vi "SetUpDigi.vi"(0 "Digitizer Settings":T31={"Digitizer delay (us) "=0.0, "rf points per line"=2048, "lines per plane"=128, "Samp Rate (Hz)"=100000000.0, "Additional dig delay (us)"=0.0, "Voltage Scale"=0.4, "Pre-Looks"=0, "Offset delay (us)"=0.0, "bits A/D"=8, "Avg Num"=1, "DigTimeOut"=5.0, "Rel Dig Delay"=0.0, "Dig Ch"=0, "LeCroyCluster"={"LeCroy Channels"=[TRUE, FALSE, FALSE, FALSE], "LC read pt offset"=0.0, "Sweep Avg"=FALSE}, "Main Digitizer"=enum."NI Digitizer", "Dig Config"=enum."Single channel", "Digitizer ID Cluster"={"Acqiris/Alazar/SP ID"=[], "NI Instr Handles"=[], "LeCroy VISA"="", "GaGe Handle"={"Handle"=0, "Sample size"=0, "Resolution"=0, "Offset"=0, "Channels"=0, "Boards"=0}, "ATS Ref"="ATS9350", "Acqiris Address"=["PCI::INSTR0"], "ADQRef"=refnum, "adq_cu_ptr"=refnum}, "Trigger Settings"={"Trig Source"=1, "Trig Coupling"=0, "Trig Slope"=0, "Level (mV)"=1500.0}, "Bulk Acq"=FALSE, "Bulk Start Indexes"=[], "Data Ref RF"=refnum, "NI ID/Channel"=[], "Total Dig CH"=1, "Xtra Ann Trig delay (us)"=10.0, "Fix Z Delay?"=FALSE, "One Way Transmission?"=FALSE, "Data Ref Log"=refnum} {"Trigger Settings"."Trig Slope" items=["Positive", "Negative"]; "Trigger Settings"."Level (mV)" format="%.2f"; "Trigger Settings"."Trig Coupling" items=["DC 1 MOhm", "AC 1 MOhm", "DC 50 Ohm", "AC 50 Ohm"]; "Trigger Settings"."Trig Source" items=["Chan 1", "External"]; "Rel Dig Delay" format="%.2f"; "DigTimeOut" format="%.2f"; "Avg Num" min=1; "Offset delay (us)" format="%.2f"; "Additional dig delay (us)" format="%.2f"; "Digitizer delay (us)" format="%.2f"}, 1 "Motion Settings In":T27={"No Motion?"=FALSE, "Motion System"=enum."NI 735x", "Motion Bd ID"=1, "Motion Profile"="SMAC1", "# Axis"=1, "Reverse Z axis?"=TRUE, "SMAC Axis"=0, "scan pair"=enum."y-(x) scan", "RT fps"=6.0, "Steps per mm"=[1000, 1000, 1000, 1000], "Motor Parameters"={"velocity ct/s"=[10000.0, 10000.0, 10000.0, 50000.0], "accel ct/s^2"=[50000.0, 50000.0, 50000.0, 200000.0]}, "One Way Scan"=FALSE, "Reverse One Way Scan"=FALSE, "Global Position (mm)"=[], "Plane"=0, "Distance between\nscan lines (um)"=0.0, "Distance between\nscan planes (um)"=0.0, "number of scan planes"=1, "Total steps in line"=0, "Xtra plane\ndistance  (um)"=100, "Xtra planes "=1, "Add Axis"=FALSE, "overshoot cts"=200, "BKPT Shift"=0, "Scan Start Time (ms)"=0, "ESP VISA"="GPIB::1::INSTR", "3rd Axis"=1, "GL Ref Out"=refnum, "Galil Address"=""} {"3rd Axis" items=["x", "y", "z", "w"]; "Xtra planes" min=1; "Xtra plane\ndistance  (um)" min=0; "Distance between\nscan planes (um)" format="%.2f"; "Distance between\nscan lines (um)" format="%.2f"; "SMAC Axis" items=["None"=0, "Axis 1"=1, "Axis 2"=2, "Axis 3"=3, "Axis 4"=4, "Axis 5"=5, "Axis 6"=6, "Axis 7"=7, "Axis 8"=8, "Vector Space 1"=17, "Vector Space 2"=18, "Vector Space 3"=19, "Vector Space 4"=20]; "Motion Bd ID" min=1 max=32 step=1}, 3 "Ann Array Params":T23={"Synth Foc?"=FALSE, "Focal Zones"=41, "Switch T/R"=0, "Trans Geometry (mm)"={"Transducer"=0, "Geo Focus"=12.0, "a (radius)"=3.0, "# of rings"=5, "kerf space "=0.1, "Center Freq"=12.0}, "Sub Ap Excite?"=FALSE, "Full Array Scan?"=FALSE, "Xmt/Rcv"={"XMIT"=[TRUE, TRUE, TRUE, TRUE, TRUE], "RCV"=[TRUE, TRUE, TRUE, TRUE, TRUE]}, "PulseSpacing (us)"=0.0, "Xmit Ring"=0, "XMIT CHS"=0, "RCV CHS"=0, "GPU?"=FALSE, "Save TIFF?"=FALSE, "downfactor"=1, "RCV 1CH"=0} {"RCV 1CH" items=["All", "1", "2", "3", "4", "5"]; "Trans Geometry (mm)"."Transducer" items=["6D 12R 40 MHz"=0, "10D 31R 20 MHz"=1, "10D 23R 20 MHz"=2, "6D 23R 40 MHz"=3, "4.5D 10.7R 40 MHz"=4, "9D 23.5R 20 MHz"=5, "9D 25.8R 20MHz"=6, "Enter"=99]; "Switch T/R" min=1 max=5 step=1}, 5 "Type of scan":T2=enum."M scan", 6 "Therapy VISA session":refnum<visa-resource-name>, 7 "Therapy (T)":bool, 8 "QAM Gate?":bool, 9 "Dual XDCR Settings":T3 {"XDCR Settings"."UT340 Controls"."Low Pass Filter (MHz)" min=-6 max=60 step=1; "XDCR Settings"."UT340 Controls"."High Pass Filter (MHz)" min=1 max=20 step=1; "XDCR Settings"."UT340 Controls"."Rep Rate (Hz)" min=20 step=1; "XDCR Settings"."UT340 Controls"."Pulse Width (ns)" min=100.0 max=250.0 step=2.0; "XDCR Settings"."UT340 Controls"."Voltage" min=100 max=250 step=2; "XDCR Settings"."UT340 Controls"."PC Gain (dB)" min=2 max=72; "XDCR Settings"."UT340 Controls"."PE Gain (dB)" min=-6 max=60 step=1; "XDCR Settings"."JSR Complete"."JSR Trigger Settings"."PRF (Hz)" items=["100 Hz"=0.1, "200 Hz"=0.2, "400 Hz"=0.4, "600 Hz"=0.6, "800 Hz"=0.8, "1000 Hz"=1.0, "1250 Hz"=1.25, "1500 Hz"=1.5, "1750 Hz"=1.75, "2000 Hz"=2.0, "2500 Hz"=2.5, "3000 Hz"=3.0, "3500 Hz"=3.5, "4000 Hz"=4.0, "4500 Hz"=4.5, "5000 Hz"=5.0]; "XDCR Settings"."JSR Complete"."JSR Trigger Settings"."Trigger Source" items=["Internal", "External"]; "XDCR Settings"."JSR Complete"."JSR Trigger Settings"."External Trigger Limit" items=["No Limit", "5 kHz"]; "XDCR Settings"."JSR Complete"."JSR Receive Settings"."Gain (dB)" min=-13 max=66 step=1; "XDCR Settings"."JSR Complete"."JSR Receive Settings"."Low Pass Filter" items=["5 MHz"=5, "10 MHz"=10, "15 MHz"=15, "22.5 MHz"=22, "35 MHz"=35, "50 MHz"=50]; "XDCR Settings"."JSR Complete"."JSR Receive Settings"."High Pass Filter" items=["DC"=0, "1 MHz"=1000, "2.5 MHz"=2500, "5 MHz"=5000, "7.5 MHz"=7500, "12.5 MHz"=12500]; "XDCR Settings"."JSR Complete"."JSR Receive Settings"."Receiver Mode" items=["Echo", "Through"]; "XDCR Settings"."JSR Complete"."JSR Pulse Settings"."Pulser Voltage (V)" items=["100"=100, "125"=125, "150"=150, "175"=175, "200"=200, "225"=225, "250"=250, "275"=275, "300"=300, "325"=325, "350"=350, "375"=375, "400"=400, "425"=425, "450"=450, "475"=475]; "XDCR Settings"."JSR Complete"."JSR Pulse Settings"."Pulser Impedance" items=["High z", "Low z"]; "XDCR Settings"."JSR Complete"."JSR Pulse Settings"."Pulse Energy Level" items=["0 (Minimum)", "1", "2", "3 (Maximum)"]; "XDCR Settings"."JSR Complete"."JSR Pulse Settings"."Damping" items=["331 Ohms"=331, "198 Ohms"=198, "142 Ohms"=142, "110 Ohms"=110, "92 Ohms"=92, "77 Ohms"=77, "67 Ohms"=67, "59 Ohms"=59, "52 Ohms"=52, "47 Ohms"=47, "43 Ohms"=43, "39 Ohms"=39, "37 Ohms"=37, "34 Ohms"=34, "32 Ohms"=32, "30 Ohms"=30]; "XDCR Settings"."Panametrics Settings"."FINE ATTENUATION" items=["00.0", "00.5", "01.0", "01.5", "02.0", "02.5", "03.0", "03.5", "04.0", "04.5", "05.0", "05.5", "06.0", "06.5", "07.0", "07.5", "08.0", "08.5", "09.0", "09.5", "10.0", "10.5", "11.0", "11.5", "12.0", "12.5", "13.0", "13.5", "14.0", "14.5", "15.0", "15.5"]; "XDCR Settings"."Panametrics Settings"."COARSE ATTENUATION" items=["00.0", "10.0", "20.0", "30.0", "40.0", "50.0"]; "XDCR Settings"."Panametrics Settings"."GAIN (db)" items=["26.0", "40.0", "54.0"]; "XDCR Settings"."Panametrics Settings"."PRF (KHz)" items=["XREMT", "EXBNC", "0.200", "0.500", "1.000", "2.000", "5.000", "10.00", "20.00"]; "XDCR Settings"."Panametrics Settings"."MODE" items=["P/ E", "THRU", "RPP", "EXT_PLSR"]; "XDCR Settings"."Panametrics Settings"."LP FILT (MHz)" items=["20", "50", "100", "200"]; "XDCR Settings"."Panametrics Settings"."HP FILT (KHz)" items=["1", "1000", "3000", "10000"]; "XDCR Settings"."Panametrics Settings"."DAMPING (Ohm)" items=["7", "10", "16", "20", "26", "30", "40", "50"]; "XDCR Settings"."Panametrics Settings"."ENERGY (uJ)" items=["1", "2", "4", "8", "16", "32"]; "XDCR Settings"."Daxsonics Settings"."Freq (MHz)" items=["4"=4, "5"=5, "6"=6, "8"=8, "10"=10, "12"=12, "14"=14, "15"=15, "16"=16, "17"=17, "18"=18, "20"=20, "25"=25, "30"=30, "35"=35, "40"=40, "45"=45, "50"=50]; "XDCR Settings"."Daxsonics Settings"."Voltage (V)" items=["0"=0, "5"=5, "10"=10, "15"=15, "20"=20, "25"=25, "30"=30, "35"=35, "40"=40, "45"=45, "50"=50, "55"=55, "60"=60, "65"=65, "70"=70, "75"=75, "80"=80, "85"=85, "90"=90, "95"=95, "100"=100, "110"=110, "120"=120, "130"=130, "140"=140, "150"=150, "160"=160, "170"=170, "180"=180, "190"=190]; "XDCR Settings"."Daxsonics Settings"."Gain (dB)" items=["22"=22, "25"=25, "28"=28, "31"=31, "34"=34, "37"=37, "40"=40, "43"=43, "46"=46, "49"=49, "52"=52, "55"=55, "58"=58, "61"=61, "64"=64, "67"=67]; "XDCR Settings"."Digitizer Settings"."Additional dig delay (ms)" format="%.2f"; "XDCR Settings"."Digitizer Settings"."Time scale per Div" items=["100 ns"=0.1, "200 ns"=0.2, "500 ns"=0.5, "1 micros"=1.0, "2 micros"=2.0, "5 micros"=5.0, "10 micros"=10.0, "20 micros"=20.0, "50 micros"=50.0, "100 micros"=100.0, "200 micros"=200.0, "500 micros"=500.0, "1 ms"=1000.0, "2 ms"=2000.0, "5 ms"=5000.0, "10 ms"=10000.0, "20 ms"=20000.0, "50 ms"=50000.0, "100 ms"=100000.0, "200 ms"=200000.0]; "XDCR Settings"."Digitizer Settings"."RF data Sampling"."rf points per line" min=1; "XDCR Settings"."Digitizer Settings"."RF data Sampling"."Ref Delay (ms)" format="%.2f"}, 18 "Equivalent RT delay\ndistance (mm)":dbl=1.5 format="%.4f") -> (11 "Dual XDCR Settings Out":T3 {"XDCR Settings"."UT340 Controls"."Low Pass Filter (MHz)" min=-6 max=60 step=1; "XDCR Settings"."UT340 Controls"."High Pass Filter (MHz)" min=1 max=20 step=1; "XDCR Settings"."UT340 Controls"."Rep Rate (Hz)" min=20 step=1; "XDCR Settings"."UT340 Controls"."Pulse Width (ns)" min=100.0 max=250.0 step=2.0; "XDCR Settings"."UT340 Controls"."Voltage" min=100 max=250 step=2; "XDCR Settings"."UT340 Controls"."PC Gain (dB)" min=2 max=72; "XDCR Settings"."UT340 Controls"."PE Gain (dB)" min=-6 max=60 step=1; "XDCR Settings"."JSR Complete"."JSR Trigger Settings"."PRF (Hz)" items=["100 Hz"=0.1, "200 Hz"=0.2, "400 Hz"=0.4, "600 Hz"=0.6, "800 Hz"=0.8, "1000 Hz"=1.0, "1250 Hz"=1.25, "1500 Hz"=1.5, "1750 Hz"=1.75, "2000 Hz"=2.0, "2500 Hz"=2.5, "3000 Hz"=3.0, "3500 Hz"=3.5, "4000 Hz"=4.0, "4500 Hz"=4.5, "5000 Hz"=5.0]; "XDCR Settings"."JSR Complete"."JSR Trigger Settings"."Trigger Source" items=["Internal", "External"]; "XDCR Settings"."JSR Complete"."JSR Trigger Settings"."External Trigger Limit" items=["No Limit", "5 kHz"]; "XDCR Settings"."JSR Complete"."JSR Receive Settings"."Gain (dB)" min=-13 max=66 step=1; "XDCR Settings"."JSR Complete"."JSR Receive Settings"."Low Pass Filter" items=["5 MHz"=5, "10 MHz"=10, "15 MHz"=15, "22.5 MHz"=22, "35 MHz"=35, "50 MHz"=50]; "XDCR Settings"."JSR Complete"."JSR Receive Settings"."High Pass Filter" items=["DC"=0, "1 MHz"=1000, "2.5 MHz"=2500, "5 MHz"=5000, "7.5 MHz"=7500, "12.5 MHz"=12500]; "XDCR Settings"."JSR Complete"."JSR Receive Settings"."Receiver Mode" items=["Echo", "Through"]; "XDCR Settings"."JSR Complete"."JSR Pulse Settings"."Pulser Voltage (V)" items=["100"=100, "125"=125, "150"=150, "175"=175, "200"=200, "225"=225, "250"=250, "275"=275, "300"=300, "325"=325, "350"=350, "375"=375, "400"=400, "425"=425, "450"=450, "475"=475]; "XDCR Settings"."JSR Complete"."JSR Pulse Settings"."Pulser Impedance" items=["High z", "Low z"]; "XDCR Settings"."JSR Complete"."JSR Pulse Settings"."Pulse Energy Level" items=["0 (Minimum)", "1", "2", "3 (Maximum)"]; "XDCR Settings"."JSR Complete"."JSR Pulse Settings"."Damping" items=["331 Ohms"=331, "198 Ohms"=198, "142 Ohms"=142, "110 Ohms"=110, "92 Ohms"=92, "77 Ohms"=77, "67 Ohms"=67, "59 Ohms"=59, "52 Ohms"=52, "47 Ohms"=47, "43 Ohms"=43, "39 Ohms"=39, "37 Ohms"=37, "34 Ohms"=34, "32 Ohms"=32, "30 Ohms"=30]; "XDCR Settings"."Panametrics Settings"."FINE ATTENUATION" items=["00.0", "00.5", "01.0", "01.5", "02.0", "02.5", "03.0", "03.5", "04.0", "04.5", "05.0", "05.5", "06.0", "06.5", "07.0", "07.5", "08.0", "08.5", "09.0", "09.5", "10.0", "10.5", "11.0", "11.5", "12.0", "12.5", "13.0", "13.5", "14.0", "14.5", "15.0", "15.5"]; "XDCR Settings"."Panametrics Settings"."COARSE ATTENUATION" items=["00.0", "10.0", "20.0", "30.0", "40.0", "50.0"]; "XDCR Settings"."Panametrics Settings"."GAIN (db)" items=["26.0", "40.0", "54.0"]; "XDCR Settings"."Panametrics Settings"."PRF (KHz)" items=["XREMT", "EXBNC", "0.200", "0.500", "1.000", "2.000", "5.000", "10.00", "20.00"]; "XDCR Settings"."Panametrics Settings"."MODE" items=["P/ E", "THRU", "RPP", "EXT_PLSR"]; "XDCR Settings"."Panametrics Settings"."LP FILT (MHz)" items=["20", "50", "100", "200"]; "XDCR Settings"."Panametrics Settings"."HP FILT (KHz)" items=["1", "1000", "3000", "10000"]; "XDCR Settings"."Panametrics Settings"."DAMPING (Ohm)" items=["7", "10", "16", "20", "26", "30", "40", "50"]; "XDCR Settings"."Panametrics Settings"."ENERGY (uJ)" items=["1", "2", "4", "8", "16", "32"]; "XDCR Settings"."Daxsonics Settings"."Freq (MHz)" items=["4"=4, "5"=5, "6"=6, "8"=8, "10"=10, "12"=12, "14"=14, "15"=15, "16"=16, "17"=17, "18"=18, "20"=20, "25"=25, "30"=30, "35"=35, "40"=40, "45"=45, "50"=50]; "XDCR Settings"."Daxsonics Settings"."Voltage (V)" items=["0"=0, "5"=5, "10"=10, "15"=15, "20"=20, "25"=25, "30"=30, "35"=35, "40"=40, "45"=45, "50"=50, "55"=55, "60"=60, "65"=65, "70"=70, "75"=75, "80"=80, "85"=85, "90"=90, "95"=95, "100"=100, "110"=110, "120"=120, "130"=130, "140"=140, "150"=150, "160"=160, "170"=170, "180"=180, "190"=190]; "XDCR Settings"."Daxsonics Settings"."Gain (dB)" items=["22"=22, "25"=25, "28"=28, "31"=31, "34"=34, "37"=37, "40"=40, "43"=43, "46"=46, "49"=49, "52"=52, "55"=55, "58"=58, "61"=61, "64"=64, "67"=67]; "XDCR Settings"."Digitizer Settings"."Additional dig delay (ms)" format="%.2f"; "XDCR Settings"."Digitizer Settings"."Time scale per Div" items=["100 ns"=0.1, "200 ns"=0.2, "500 ns"=0.5, "1 micros"=1.0, "2 micros"=2.0, "5 micros"=5.0, "10 micros"=10.0, "20 micros"=20.0, "50 micros"=50.0, "100 micros"=100.0, "200 micros"=200.0, "500 micros"=500.0, "1 ms"=1000.0, "2 ms"=2000.0, "5 ms"=5000.0, "10 ms"=10000.0, "20 ms"=20000.0, "50 ms"=50000.0, "100 ms"=100000.0, "200 ms"=200000.0]; "XDCR Settings"."Digitizer Settings"."RF data Sampling"."rf points per line" min=1; "XDCR Settings"."Digitizer Settings"."RF data Sampling"."Ref Delay (ms)" format="%.2f"}, 12 "Digitizer Settings Out":T31={"Digitizer delay (us) "=0.0, "rf points per line"=2048, "lines per plane"=128, "Samp Rate (Hz)"=100000000.0, "Additional dig delay (us)"=0.0, "Voltage Scale"=0.4, "Pre-Looks"=0, "Offset delay (us)"=0.0, "bits A/D"=8, "Avg Num"=1, "DigTimeOut"=5.0, "Rel Dig Delay"=0.0, "Dig Ch"=0, "LeCroyCluster"={"LeCroy Channels"=[TRUE, FALSE, FALSE, FALSE], "LC read pt offset"=0.0, "Sweep Avg"=FALSE}, "Main Digitizer"=enum."NI Digitizer", "Dig Config"=enum."Single channel", "Digitizer ID Cluster"={"Acqiris/Alazar/SP ID"=[], "NI Instr Handles"=[], "LeCroy VISA"="", "GaGe Handle"={"Handle"=0, "Sample size"=0, "Resolution"=0, "Offset"=0, "Channels"=0, "Boards"=0}, "ATS Ref"="ATS9350", "Acqiris Address"=["PCI::INSTR0"], "ADQRef"=refnum, "adq_cu_ptr"=refnum}, "Trigger Settings"={"Trig Source"=1, "Trig Coupling"=0, "Trig Slope"=0, "Level (mV)"=1500.0}, "Bulk Acq"=FALSE, "Bulk Start Indexes"=[], "Data Ref RF"=refnum, "NI ID/Channel"=[], "Total Dig CH"=1, "Xtra Ann Trig delay (us)"=10.0, "Fix Z Delay?"=FALSE, "One Way Transmission?"=FALSE, "Data Ref Log"=refnum} {"Trigger Settings"."Trig Slope" items=["Positive", "Negative"]; "Trigger Settings"."Level (mV)" format="%.2f"; "Trigger Settings"."Trig Coupling" items=["DC 1 MOhm", "AC 1 MOhm", "DC 50 Ohm", "AC 50 Ohm"]; "Trigger Settings"."Trig Source" items=["Chan 1", "External"]; "Rel Dig Delay" format="%.2f"; "DigTimeOut" format="%.2f"; "Avg Num" min=1; "Offset delay (us)" format="%.2f"; "Additional dig delay (us)" format="%.2f"; "Digitizer delay (us)" format="%.2f"}, 13 "Motion Settings Out":T27={"No Motion?"=FALSE, "Motion System"=enum."NI 735x", "Motion Bd ID"=1, "Motion Profile"="SMAC1", "# Axis"=1, "Reverse Z axis?"=TRUE, "SMAC Axis"=0, "scan pair"=enum."y-(x) scan", "RT fps"=6.0, "Steps per mm"=[1000, 1000, 1000, 1000], "Motor Parameters"={"velocity ct/s"=[10000.0, 10000.0, 10000.0, 50000.0], "accel ct/s^2"=[50000.0, 50000.0, 50000.0, 200000.0]}, "One Way Scan"=FALSE, "Reverse One Way Scan"=FALSE, "Global Position (mm)"=[], "Plane"=0, "Distance between\nscan lines (um)"=0.0, "Distance between\nscan planes (um)"=0.0, "number of scan planes"=1, "Total steps in line"=0, "Xtra plane\ndistance  (um)"=100, "Xtra planes "=1, "Add Axis"=FALSE, "overshoot cts"=200, "BKPT Shift"=0, "Scan Start Time (ms)"=0, "ESP VISA"="GPIB::1::INSTR", "3rd Axis"=1, "GL Ref Out"=refnum, "Galil Address"=""} {"3rd Axis" items=["x", "y", "z", "w"]; "Xtra planes" min=1; "Xtra plane\ndistance  (um)" min=0; "Distance between\nscan planes (um)" format="%.2f"; "Distance between\nscan lines (um)" format="%.2f"; "SMAC Axis" items=["None"=0, "Axis 1"=1, "Axis 2"=2, "Axis 3"=3, "Axis 4"=4, "Axis 5"=5, "Axis 6"=6, "Axis 7"=7, "Axis 8"=8, "Vector Space 1"=17, "Vector Space 2"=18, "Vector Space 3"=19, "Vector Space 4"=20]; "Motion Bd ID" min=1 max=32 step=1}, 14 "Vert Settings":cluster{dbl, dbl, "Coupling":u16}, 15 "RF data Sampling Out":T36={"Sampling Rate"=6.0, "Ref Delay (ms)"=0.0, "rf points per line"=2048} {"rf points per line" min=1; "Ref Delay (ms)" format="%.2f"; "Sampling Rate" items=["10 MS/s"=10.0, "20 MS/s"=20.0, "25 MS/s"=25.0, "50 MS/s"=50.0, "100 MS/s"=100.0, "200 MS/s"=200.0, "250 MS/s"=250.0, "500 MS/s"=500.0, "1 GS/s"=1000.0]}, 17 "Waveform Graph":cluster{i32, dbl, "Array":dbl[]}(graph), 19 "Ann Array Params out":T23={"Synth Foc?"=FALSE, "Focal Zones"=41, "Switch T/R"=0, "Trans Geometry (mm)"={"Transducer"=0, "Geo Focus"=12.0, "a (radius)"=3.0, "# of rings"=5, "kerf space "=0.1, "Center Freq"=12.0}, "Sub Ap Excite?"=FALSE, "Full Array Scan?"=FALSE, "Xmt/Rcv"={"XMIT"=[TRUE, TRUE, TRUE, TRUE, TRUE], "RCV"=[TRUE, TRUE, TRUE, TRUE, TRUE]}, "PulseSpacing (us)"=0.0, "Xmit Ring"=0, "XMIT CHS"=0, "RCV CHS"=0, "GPU?"=FALSE, "Save TIFF?"=FALSE, "downfactor"=1, "RCV 1CH"=0} {"RCV 1CH" items=["All", "1", "2", "3", "4", "5"]; "Trans Geometry (mm)"."Transducer" items=["6D 12R 40 MHz"=0, "10D 31R 20 MHz"=1, "10D 23R 20 MHz"=2, "6D 23R 40 MHz"=3, "4.5D 10.7R 40 MHz"=4, "9D 23.5R 20 MHz"=5, "9D 25.8R 20MHz"=6, "Enter"=99]; "Switch T/R" min=1 max=5 step=1})   [LabVIEW 2022 SP3]
uses:
  -DigitizerRoutines/DigitizerSettings.ctl
  -DigitizerRoutines/Digitizer.ctl
  -DigitizerRoutines/DigConfig.ctl
  -DigitizerRoutines/DigitizerID.ctl
  C:/Windows/System32/ADQAPI_dotNet_helper.dll
  Windows/System32/ADQAPI_dotNet_helper.dll
  Motion Controllers/NI_controller/-NI_MotionRoutines/MotionParameters.ctl
  Motion Controllers/NI_controller/-NI_MotionRoutines/MotionSys.ctl
  Motion Controllers/-MotionRoutines/ScanAxis.ctl
  Motion Controllers/-MotionRoutines/3rdAxis.ctl
  Annular Array/-AnnularRoutines/AnnularArray.ctl
  Annular Array/-AnnularRoutines/TransGeometry.ctl
  Annular Array/-AnnularRoutines/ArrayGeometry.ctl
  Pulsers/pulser.ctl
  DualXDCR/Dual XDCR Complete Settings.ctl
  DualXDCR/XDCRSettings.ctl
  Pulsers/Daxsonics/-DaxSubroutines/Dax_Control_Cluster.ctl
  Pulsers/Panametrics/Pana5900.ctl
  Pulsers/JSR/Controls/JSR Complete.ctl
  Pulsers/JSR/Controls/JSR Pulse.ctl
  Pulsers/JSR/Controls/Damping.ctl
  Pulsers/JSR/Controls/Energy.ctl
  Pulsers/JSR/Controls/Z.ctl
  Pulsers/JSR/Controls/Volt.ctl
  Pulsers/JSR/Controls/JSR Recieve.ctl
  Pulsers/JSR/Controls/Mode.ctl
  Pulsers/JSR/Controls/HPF.ctl
  Pulsers/JSR/Controls/LPF.ctl
  Pulsers/JSR/Controls/Gain.ctl
  Pulsers/JSR/Controls/JSR Trigger.ctl
  Pulsers/JSR/Controls/Trig Limit.ctl
  Pulsers/JSR/Controls/Trig Source.ctl
  Pulsers/JSR/Controls/PRF.ctl
  Pulsers/UTEX/Controls/UTEX Controls.ctl
  -ScanSystem/Controls/ScanType2.ctl
  Motion Controllers/Galil/Command Menu.ctl
  -ScanSystem/Controls/location.ctl
  <vilib>/DAQmx/write.llb/DAQmx Write (Digital Bool 1Line 1Point).vi
  <vilib>/Analysis/2dsp.llb/Decimate (single shot, DBL).vi
  <vilib>/Analysis/baseanly.llb/Mean (DBL).vi
  Motion Controllers/-MotionRoutines/MotionGlobals.vi
  Pulsers/PulserGlobals.vi
  Switch Modules/SwitchGlobals.vi
  <vilib>/DAQmx/miscellaneous.llb/DAQmx Fill In Error Info.vi
  <vilib>/DAQmx/create/channels.llb/DAQmx Create Channel (CO-Pulse Generation-Frequency).vi
  <vilib>/DAQmx/configure/timing.llb/DAQmx Timing (Implicit).vi
  <vilib>/DAQmx/create/channels.llb/DAQmx Create Channel (CO-Pulse Generation-Time).vi
  <vilib>/DAQmx/configure/trigger.llb/DAQmx Start Trigger (Digital Edge).vi
  <instrlib>/niScope/Acquire/Fetch/niScope Fetch.vi
  <vilib>/Utility/file.llb/Write Delimited Spreadsheet (DBL).vi
  -DigitizerRoutines/DigitizerGlobals.vi
  <resource>/objmgr/daqmx.rc
  <instrlib>/Newport ESP301/Newport ESP301.lvlib
  <instrlib>/Acqiris Dx/Acqiris Dx.lvlib
  <instrlib>/Acqiris Bx/Acqiris Bx.lvlib
  <vilib>/Analysis/NI_AALBase.lvlib
  <vilib>/Analysis/NI_AALPro.lvlib
  <instrlib>/niSwitch/niSwitch.llb/niSwitch Connect Channels (Single).vi
  <vilib>/Motion/FlexMotion/FunctionsVIs/StartStopMotion.llb/Start Motion (8 axes).flx
  <vilib>/Motion/FlexMotion/FunctionsVIs/StartStopMotion.llb/Stop Motion (8 axes).flx
panel:
  out "Samp rate":dbl
  out "AlazarCluster":T1
  in  "Norm Spect?":bool
  in  "Filter":bool
  in  "Filter Prameters":T26={"low cutoff"=5, "order"=81, "high cutoff"=65}
  in  "Inc. Step Size (mm)":dbl=0.5
  in  "Settings Changes":bool
  in  "Crate Spectra":bool
  out "Crate Waveforms":cluster{i32, "Clock (s)":dbl, dbl[][]}(graph)
  in  "Display Channel":i32(slide) min=0 max=5 step=1 scale=0.0..5.0
  in  "Position (mm) (Abs)":dbl format="%.3f"
  in  "Stop Motor":bool
  in  "Axis Tune":enum32{"Axis 1", "Axis 2", "Axis 3", "Axis 4"}(radio)
  in  "Tab Control":T35(tab)
  in  "RF data Sampling":T36={"Sampling Rate"=100.0, "Ref Delay (ms)"=0.0, "rf points per line"=2048} {"rf points per line" min=1; "Ref Delay (ms)" format="%.2f"}
  in  "Trigger Settings":T37={"Trig Source"=1, "Trig Coupling"=0, "Trig Slope"=0, "Level (mV)"=1500.0} {"Trig Slope" items=["Positive", "Negative"]; "Level (mV)" format="%.2f"; "Trig Coupling" items=["DC 1 MOhm", "AC 1 MOhm", "DC 50 Ohm", "AC 50 Ohm"]; "Trig Source" items=["Chan 1", "External"]}
  out "Error Message":string
  in  "Time scale per Div":dbl(ring)=5.0 items=["200 ns"=0.2, "400 ns"=0.4, "1 micros"=1.0, "2 micros"=2.0, "5 micros"=5.0, "10 micros"=10.0, "20 micros"=20.0, "50 micros"=50.0, "100 micros"=100.0]
  out "Total Delay (ms)":dbl=1.5 format="%.3f"
  in  "Channel tab":enum32{"C1", "C2", "C3", "C4"}(tab)
  in  "Volt Scale 1":dbl(ring)=2.0 items=["8 V"=8.0, "4 V"=4.0, "2 V"=2.0, "800 mV"=0.8, "400 mV"=0.4, "200 mV"=0.2, "80 mV"=0.08]
  in  "Coupling C1":u16(ring)=2 items=["DC 1 MOhm", "AC 1 MOhm", "DC 50 Ohm", "AC 50 OHM"]
  in  "Volt Scale 2":dbl(ring)=0.4 items=["8 V"=8.0, "4 V"=4.0, "2 V"=2.0, "800 mV"=0.8, "400 mV"=0.4, "200 mV"=0.2, "80 mV"=0.08]
  in  "Coupling C2":u16(ring)=2 items=["DC 1 MOhm", "AC 1 MOhm", "DC 50 Ohm", "AC 50 OHM"]
  in  "Volt Scale 3":dbl(ring)=0.4 items=["8 V"=8.0, "4 V"=4.0, "2 V"=2.0, "800 mV"=0.8, "400 mV"=0.4, "200 mV"=0.2, "80 mV"=0.08]
  in  "Coupling C3":u16(ring)=2 items=["DC 1 MOhm", "AC 1 MOhm", "DC 50 Ohm", "AC 50 OHM"]
  in  "Volt Scale 4":dbl(ring)=0.4 items=["8 V"=8.0, "4 V"=4.0, "2 V"=2.0, "800 mV"=0.8, "400 mV"=0.4, "200 mV"=0.2, "80 mV"=0.08]
  in  "Coupling C4":u16(ring)=2 items=["DC 1 MOhm", "AC 1 MOhm", "DC 50 Ohm", "AC 50 OHM"]
  in  "Therapy Burst Set Up":T38={"Therapy Set Up"={"Cycles"=1.0, "Frequency (MHz)"=40.0, "Amplitude (mV)"=200.0}, "Divide prf by"=1, "Therapy Delay (ms) "=10.0, "Counter On (T)"=TRUE} {"Therapy Delay (ms)" min=0.025 format="%.3f"; "Therapy Set Up"."Amplitude (mV)" min=50.0 max=1000.0 format="%.2f"; "Therapy Set Up"."Frequency (MHz)" min=0.01 max=200.0 format="%.4f"; "Therapy Set Up"."Cycles" min=1 max=50000 step=1 format="%.3f"}
  out "Lines in burst":i32=1 min=1 max=50000 step=1
  in  "Gate duration (mics)":dbl=12.0 min=0.025
  in  "cycles (f), time(t)":bool=TRUE
  in  "Func Gen":u16(ring)=1 items=["Agilent", "Tabor"]
  in  "Config Breath":bool
  in  "Set Spectrometer":bool
  in  "Delay Corr?":bool=TRUE
  in  "Offset (mV)":dbl
  in  "Custom Waveform":bool
  in  "Pulser":T39
  in  "Offset delay (us)":dbl
  in  "One Way Transmission?":bool
  in  "Attenuation":u8(slide) scale=0.0..63.0
  out "Gage Delay Pts":dbl
  out "CTR Tasks":refnum<k21>[](array[refnum])
  in  "Slave Voltage Scales":bool=TRUE
  out "Nominal Samples":i32
  out "t per div":dbl
  in  "Crate Voltage Scales":dbl[](array[ring])=[2.0, 2.0, 2.0, 2.0] items=["8 V"=8.0, "4 V"=4.0, "2 V"=2.0, "800 mV"=0.8, "400 mV"=0.4, "200 mV"=0.2, "80 mV"=0.08]
  in  "Crate Delay":dbl
  in  "Display Crate?":bool
  in  "Man Cont":bool
  in  "T/R Channel":u32(slide)=1 min=1 max=8 step=1 scale=1.0..5.0
  in  "Save trace?":bool
  in  "Set Pulser":bool
  in  "go to scan type":bool
  in  "ExitSendCmd":bool
  in  "Crate Coupling":u16(ring)=2 items=["DC 1 MOhm", "AC 1 MOhm", "DC 50 Ohm", "AC 50 OHM"]
  out "dup id":i32
  # "Key Board Short Cuts\nX: \t      Autoscale in X\nY: \t      Autoscale in Y\nSpace Bar:           Exit\n\nShift:           Step * 0.1\nCtrl:          Step * 0.01"
  # "Z: \t\t             +W\nC: \t\t              -W\nPageUp:      \t+Z\nPageDown:\t   -Z\nUp Arrow:\t    +Y\nDown Arrow: \t-Y\nLeft Arrow: \t  +X\nRight Arrow:  -X"
  # "© 2000-2022 Weill Cornel"
  # "Array Mode Settings and Display"
  # "Position Adjustment"
  # "Yellow curser used for additional delay. RF data is captured between yellow and red lines."
  # "All"
  # "1-D and 2-D B scan settings"
  # "1-D and 2-D B scan settings"
  # "Scale Settings"
  # "Controls only visible\nwhen needed.."
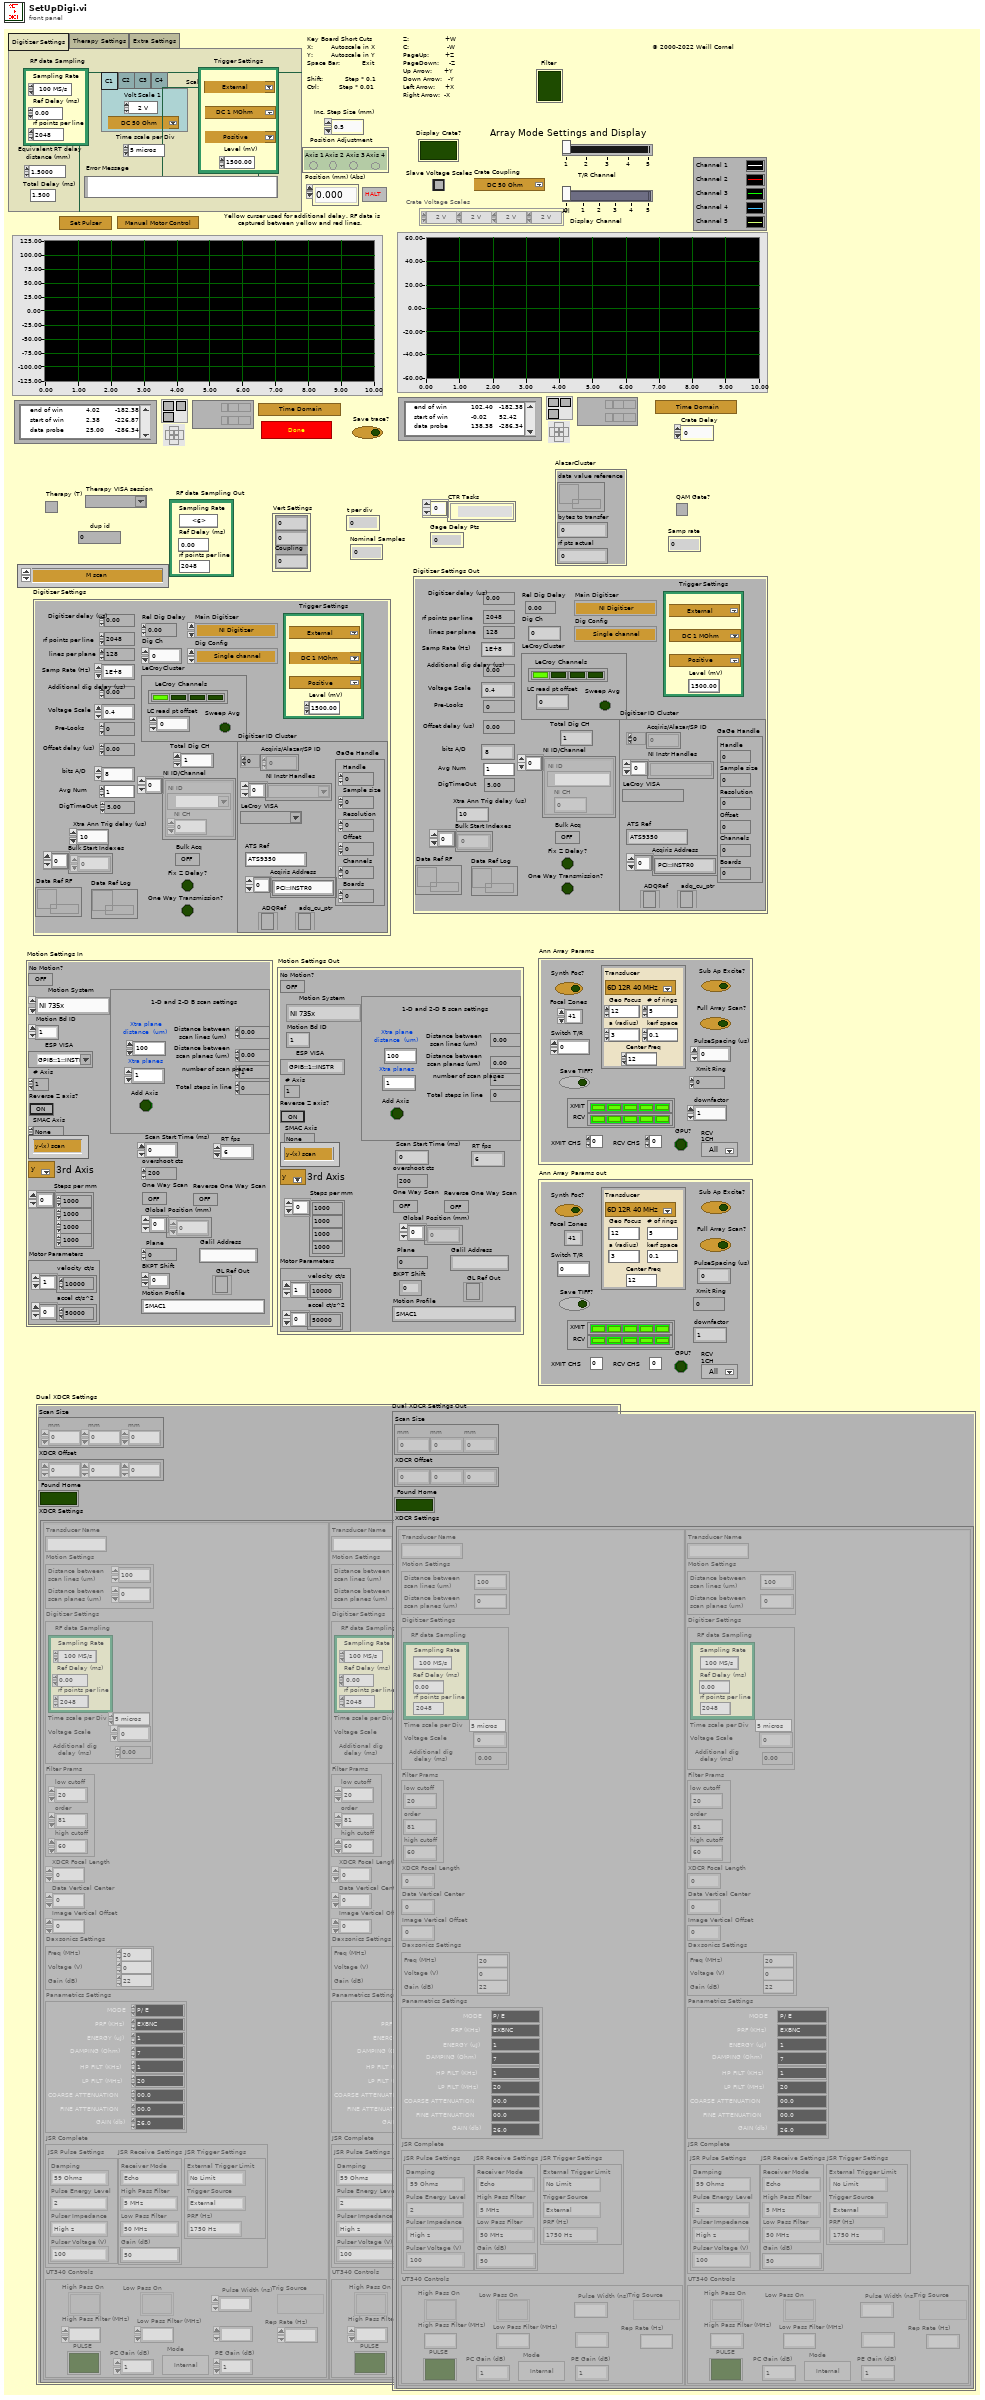
[diagram p1: front panel]
types:
  T1 = cluster{"data value reference":refnum<data-value>, "bytes to transfer":u32, "rf pts actual":u32}
  T2 = typedef "ScanType2.ctl" = enum16{"Therapy With Scan", "M scan", "M Scan With Therapy Burst", "1-D B Scan", "1-D B Scan With Therapy Burst", "2-D B Scan", "2-D B Scan With Therapy Burst", "Rotational Scan", "1-D B-Scan PRF", "2-D B-Scan PRF", "Real-Time Scan", "Contrast Agents", "1-D w/ Real-Time Set Up", "Dual Transducer", "Acoustic Microscopy", "Hydrophone Scanning"}
  T3 = typedef "Dual XDCR Complete Settings.ctl" = cluster{"Scan Size":dbl[], "XDCR Offset":dbl[], "Found Home":bool, "XDCR Settings":T4[]}
  T4 = typedef "XDCRSettings.ctl" = cluster{"Transducer Name":string, "Motion Settings":cluster{"Distance between\nscan lines (um)":sgl, "Distance between\nscan planes (um)":sgl}, "Digitizer Settings":cluster{"RF data Sampling":cluster{"Sampling Rate":dbl, "Ref Delay (ms)":dbl, "rf points per line":i32}, "Time scale per Div":dbl, "Voltage Scale":dbl, "Additional dig delay (ms)":dbl}, "Filter Prams":cluster{"low cutoff":i32, "order":i32, "high cutoff":i32}, "XDCR Focal Length":dbl, "Data Vertical Center":dbl, "Image Vertical Offset":dbl, "Daxsonics Settings":T5, "Panametrics Settings":T6, "JSR Complete":T7, "UT340 Controls":T22}
  T5 = typedef "Dax_Control_Cluster.ctl" = cluster{"Freq (MHz) ":u16, "Voltage (V)":u16, "Gain (dB)":u16}
  T6 = typedef "Pana5900.ctl" = cluster{"ENERGY (uJ)":u16, "DAMPING (Ohm)":u16, "HP FILT (KHz) ":u16, "LP FILT (MHz)":u16, "MODE":u16, "PRF (KHz)":u16, "GAIN (db)":u16, "COARSE ATTENUATION":u16, "FINE ATTENUATION":u16}
  T7 = typedef "JSR Complete.ctl" = cluster{"JSR Pulse Settings":T8, "JSR Receive Settings":T13, "JSR Trigger Settings":T18}
  T8 = typedef "JSR Pulse.ctl" = cluster{"Damping":T9, "Pulse Energy Level":T10, "Pulser Impedance":T11, "Pulser Voltage (V)":T12}
  T9 = typedef "Damping.ctl" = i16
  T10 = typedef "Energy.ctl" = u16
  T11 = typedef "Z.ctl" = u16
  T12 = typedef "Volt.ctl" = i16
  T13 = typedef "JSR Recieve.ctl" = cluster{"Receiver Mode":T14, "High Pass Filter":T15, "Low Pass Filter":T16, "Gain (dB)":T17}
  T14 = typedef "Mode.ctl" = i8
  T15 = typedef "HPF.ctl" = u16
  T16 = typedef "LPF.ctl" = u16
  T17 = typedef "Gain.ctl" = i8
  T18 = typedef "JSR Trigger.ctl" = cluster{"External Trigger Limit":T19, "Trigger Source":T20, "PRF (Hz)":T21}
  T19 = typedef "Trig Limit.ctl" = i8
  T20 = typedef "Trig Source.ctl" = i8
  T21 = typedef "PRF.ctl" = dbl
  T22 = typedef "UTEX Controls.ctl" = cluster{"High Pass On":bool, "High Pass Filter (MHz)":i16, "Low Pass On":bool, "Low Pass Filter (MHz)":i16, "PE Gain (dB)":i16, "Voltage":i16, "Pulse Width (ns)":dbl, "Mode":bool, "PC Gain (dB)":i16, "Trig Source":bool, "Rep Rate (Hz)":i16, "PULSE":bool}
  T23 = typedef "AnnularArray.ctl" = cluster{"Synth Foc?":bool, "Focal Zones":i16, "Switch T/R":i16, "Trans Geometry (mm)":T24, "Sub Ap Excite?":bool, "Full Array Scan?":bool, "Xmt/Rcv":cluster{"XMIT":bool[], "RCV":bool[]}, "PulseSpacing (us)":sgl, "Xmit Ring":i32, "XMIT CHS":u8, "RCV CHS":u8, "GPU?":bool, "Save TIFF?":bool, "downfactor":i32, "RCV 1CH":u16}
  T24 = typedef "TransGeometry.ctl" = cluster{"Transducer":T25, "Geo Focus":dbl, "a (radius)":dbl, "# of rings":i32, "kerf space ":dbl, "Center Freq":dbl}
  T25 = typedef "ArrayGeometry.ctl" = u16
  T26 = cluster{"low cutoff":i32, "order":i32, "high cutoff":i32}
  T27 = typedef "MotionParameters.ctl" = cluster{"No Motion?":bool, "Motion System":T28, "Motion Bd ID":u8, "Motion Profile":string, "# Axis":i8, "Reverse Z axis?":bool, "SMAC Axis":u16, "scan pair":T29, "RT fps":sgl, "Steps per mm":i32[], "Motor Parameters":cluster{"velocity ct/s":dbl[], "accel ct/s^2":dbl[]}, "One Way Scan":bool, "Reverse One Way Scan":bool, "Global Position (mm)":dbl[], "Plane":i32, "Distance between\nscan lines (um)":sgl, "Distance between\nscan planes (um)":sgl, "number of scan planes":i32, "Total steps in line":i32, "Xtra plane\ndistance  (um)":i32, "Xtra planes ":i32, "Add Axis":bool, "overshoot cts":i32, "BKPT Shift":i32, "Scan Start Time (ms)":u32, "ESP VISA":refnum<visa-resource-name>, "3rd Axis":T30, "GL Ref Out":refnum<k7>, "Galil Address":string}
  T28 = typedef "MotionSys.ctl" = enum16{"MM3000", "NI 735x", "Newport ESP", "No Motion Card", "Galil"}
  T29 = typedef "ScanAxis.ctl" = enum16{"y-(x) scan", "x-(y) scan", "z-(x) scan", "z-(y) scan", "y-(z) scan", "x-(z) scan", "w-(x) scan", "w-(y) scan", "w-(z) scan", "x-(w) scan", "y-(w) scan", "z-(w) scan"}
  T30 = typedef "3rdAxis.ctl" = u16
  T31 = typedef "DigitizerSettings.ctl" = cluster{"Digitizer delay (us) ":dbl, "rf points per line":i32, "lines per plane":i32, "Samp Rate (Hz)":dbl, "Additional dig delay (us)":dbl, "Voltage Scale":dbl, "Pre-Looks":i32, "Offset delay (us)":dbl, "bits A/D":i8, "Avg Num":i32, "DigTimeOut":sgl, "Rel Dig Delay":sgl, "Dig Ch":i32, "LeCroyCluster":cluster{"LeCroy Channels":bool[], "LC read pt offset":dbl, "Sweep Avg":bool}, "Main Digitizer":T32, "Dig Config":T33, "Digitizer ID Cluster":T34, "Trigger Settings":cluster{"Trig Source":u16, "Trig Coupling":u16, "Trig Slope":u16, "Level (mV)":dbl}, "Bulk Acq":bool, "Bulk Start Indexes":i32[], "Data Ref RF":refnum<data-value>, "NI ID/Channel":cluster{"NI ID":refnum<k15>, "NI CH":i32}[], "Total Dig CH":i32, "Xtra Ann Trig delay (us)":dbl, "Fix Z Delay?":bool, "One Way Transmission?":bool, "Data Ref Log":refnum<data-value>}
  T32 = typedef "Digitizer.ctl" = enum16{"Acqiris Digitizer", "NI Digitizer", "LeCroy", "GaGe", "AlazarTech", "No Digitizer", "Teledyne"}
  T33 = typedef "DigConfig.ctl" = enum16{"Single channel", "2 Chans w/ 2 Acqiris", "2 Chans w/ 1 Acqiris", "5-CH Pulser New", "5-CH pulser w/ ann array", "5-pass style ann array", "Empty"}
  T34 = typedef "DigitizerID.ctl" = cluster{"Acqiris/Alazar/SP ID":u32[], "NI Instr Handles":refnum<k15>[], "LeCroy VISA":refnum<visa-resource-name>, "GaGe Handle":cluster{"Handle":u32, "Sample size":u32, "Resolution":i32, "Offset":i32, "Channels":u32, "Boards":u32}, "ATS Ref":string, "Acqiris Address":string[], "ADQRef":refnum<k24>, "adq_cu_ptr":refnum<k24>}
  T35 = enum32{"Digitizer Settings", "Therapy Settings", "Extra Settings"}
  T36 = cluster{"Sampling Rate":dbl, "Ref Delay (ms)":dbl, "rf points per line":i32}
  T37 = cluster{"Trig Source":u16, "Trig Coupling":u16, "Trig Slope":u16, "Level (mV)":dbl}
  T38 = cluster{"Therapy Set Up":cluster{"Cycles":sgl, "Frequency (MHz)":dbl, "Amplitude (mV)":dbl}, "Divide prf by":i32, "Therapy Delay (ms) ":dbl, "Counter On (T)":bool}
  T39 = typedef "pulser.ctl" = enum16{"Pan 5900", "Daxsonics", "Agilent 33xxx", "UTEX", "JSR", "WMC Mono-Cycle", "No Pulser", "NYU AVTECH", "Tabor W1281A", "Pan 5800", "Unlisted", "Tabor WX2182B"}
  T40 = typedef "SwitchOption.ctl" = enum16{"Cytex", "Pickering", "NI Switch", "No Switch", "Riverside USB"}
  T41 = typedef "location.ctl" = enum16{"Automatic", "WCM Main", "Hawaii", "Columbia MM3000", "Columbia  NI System", "NYU", "RRI 2", "UHI Allen", "CUMC RT", "Chiba", "Stony Brook", "WCM Microscopy", "WCM Aeoretch", "WCM Optics Lab", "WCM Main 2Axis", "WCM Rotation", "WCM SAM SMAC", "SERI GP"}
  T42 = typedef "Command Menu.ctl" = enum16{"CommandPassThrough", "Abort Motion", "Define Pos", "Velocity", "Acceleration", "Deceleration", "Position Rel", "Postion Abs", "Begin Move", "After Move", "Home", "KI", "KD", "KP", "IL", "Config I/O", "Set Bit", "Clear Bit", "Motor Off", "Moto On", "Status", "Execute", "Halt Execute", "HX Status", "Tell Velocity", "Check Motion", "BreakPoint", "Tell Position", "Current Code Line", "Tell Switches", "OC Force On", "OC Off", "Pos Soft Limit", "Rev Soft Limit"}
  T43 = cluster{dbl, "Clock mode":enum16{"Internal", "External", "Reference"}, "RingText.Text":string, i32, i32, "time out (ms)":dbl, dbl, dbl}
  T44 = enum8{"Enabled", "Disabled", "Disabled and Grayed Out"}
  T45 = enum16{"Absolute Position", "Relative Position", "Velocity", "Relative to Cap Pos", "Modulus Position", "Absolute Contouring", "Relative Contouring"}
  T46 = typedef "LVStringsAndValuesArrayTypeDef_DBL.ctl" = cluster{"String":string, "Value":dbl}[]
  T47 = cluster{"Therapy frequency (MHz)":dbl, "Therapy amplitude (mV)":dbl, "time therapy on (s)":dbl, "Therapy Delay (ms) ":dbl, "Time (s)":dbl}
  T48 = cluster{"time therapy on (s)":dbl, "Therapy frequency (MHz)":dbl, "Therapy amplitude (mV)":dbl}
  T49 = cluster{"Samp Rate (Hz)":dbl, "Digitizer delay (us) ":dbl, "rf points per line":i32}
  T50 = cluster{"Port A bit-0 at logic level":bool, "Port A bit-1 at logic level":bool, "Port A bit-2 at logic level ":bool, "Port A bit-3 at logic level":bool, "Port A bit-4 at logic level":bool, "Port A bit-5 at logic level ":bool, "Port A bit-6 at logic level ":bool, "Port A bit-7 at logic level ":bool, "Port B bit-0 at logic level":bool, "Port B bit-1 at logic level":bool, "Port B bit-2 at logic level ":bool, "Port B bit-3 at logic level":bool, "Port B bit-4 at logic level":bool, "Port B bit-5 at logic level ":bool, "Port B bit-6 at logic level ":bool, "Port B bit-7 at logic level ":bool}
  T51 = cluster{"Handle":u32, "Sample size":u32, "Resolution":i32, "Offset":i32, "Channels":u32, "Boards":u32}
  T52 = cluster{"returnedSamplesPerSeg":i32, "indexFirstPoint":i32, "sampTime":dbl, "vGain":dbl, "vOffset":dbl, "returnedSegments":i32, "nbrAvgWforms":i32, "actualTriggersInAcqLo":u32, "actualTriggersInAcqHi":u32, "reserved3":dbl, "actualDataSize":u32, "missingValue":dbl}
  T53 = cluster{"actualSamples":i32, "absoluteInitialX":dbl, "relativeInitialX":dbl, "xIncrement":dbl, "offset":dbl, "gain":dbl, "reserved1":dbl, "reserved2":dbl}
  T54 = cluster{i32, dbl, "Power Spectrum (V^2 rms)":dbl[][]}
  T55 = typedef "lveventtype.ctl" = enum32{"Null", "Timeout", "Annotation Menu Selection", "Annotation Menu Selection?", "App Instance Close", "App Instance Close?", "Autoscale Range Change", "Bookmark Info Change", "Cell Edit", "Cell Edit?", "Cursor Grab", "Cursor Grab?", "Cursor Menu Selection", "Cursor Menu Selection?", "Cursor Move", "Cursor Release", "Data Change", "Direction Change", "Display State Change", "Drag Ended", "Drag Enter", "Drag Leave", "Drag Over", "Drag Source Update", "Drag Starting", "Drag Starting?", "Drop", "Exec State Change", "Key Down", "Key Down?", "Key Repeat", "Key Repeat?", "Key Up", "Listbox Double Click", "Menu Activation?", "Menu Selection (App)", "Menu Selection? (App)", "Menu Selection (User)", "Mouse Down", "Mouse Down?", "Mouse Enter", "Mouse Leave", "Mouse Move", "Mouse Up", "Mouse Wheel", "NI Security User Change (App)", "Pane Size", "Panel Close", "Panel Close?", "Panel Resize", "Plot Attribute Change", "Scale Range Change", "Shortcut Menu Activation?", "Shortcut Menu Selection (App)", "Shortcut Menu Selection? (App)", "Shortcut Menu Selection (User)", "Tree Double Click", "Tree Drag", "Tree Drag?", "Tree Drop", "Tree Drop?", "Tree Item Close", "Tree Item Close?", "Tree Item Open", "Tree Item Open?", "User Event", "Value Change"}
  T56 = typedef "Daxsonics_Pulsers.ctl" = enum16{"BP1", "BP2_A", "BP2_B", "10ERS8", "New2021"}
  T57 = typedef "eventvkey.ctl" = enum16{"ASCII", "Enter", "Return", "Shift", "Ctrl", "Alt", "Cmd", "Opt", "Caps", "NumLock", "Clear", "Break", "Up", "Down", "Left", "Right", "Insert", "Delete", "Home", "End", "PageUp", "PageDown", "Escape", "Help", "Pause", "ScrollLock", "F1", "F2", "F3", "F4", "F5", "F6", "F7", "F8", "F9", "F10", "F11", "F12", "F13", "F14", "F15", "F16", "F17", "F18", "F19", "F20", "F21", "F22", "F23", "F24", "Play", "VolumeUp", "VolumeDown", "Mute", "Two Byte Char"}
  T58 = cluster{"Shift":bool, "Ctrl":bool, "Alt":bool, "Cmd":bool, "Opt":bool}
  T59 = cluster{"Volt Scale 4":dbl, "Offset (mV)":dbl, "Coupling C4":u16}
  T60 = cluster{"Channel":dbl, dbl, "Crate Coupling":u16}
  T61 = typedef "Resource Out (Enum).flx" = u16
  T62 = typedef "Bd Id Out" = u8
  T63 = cluster{"Cycles":sgl, "Frequency (MHz)":dbl, "Amplitude (mV)":dbl}
  T64 = typedef "Breath_Mode.ctl" = u16
  T65 = typedef "SpectrometerType.ctl" = u16
  T66 = typedef "EKG_Mode.ctl" = u16
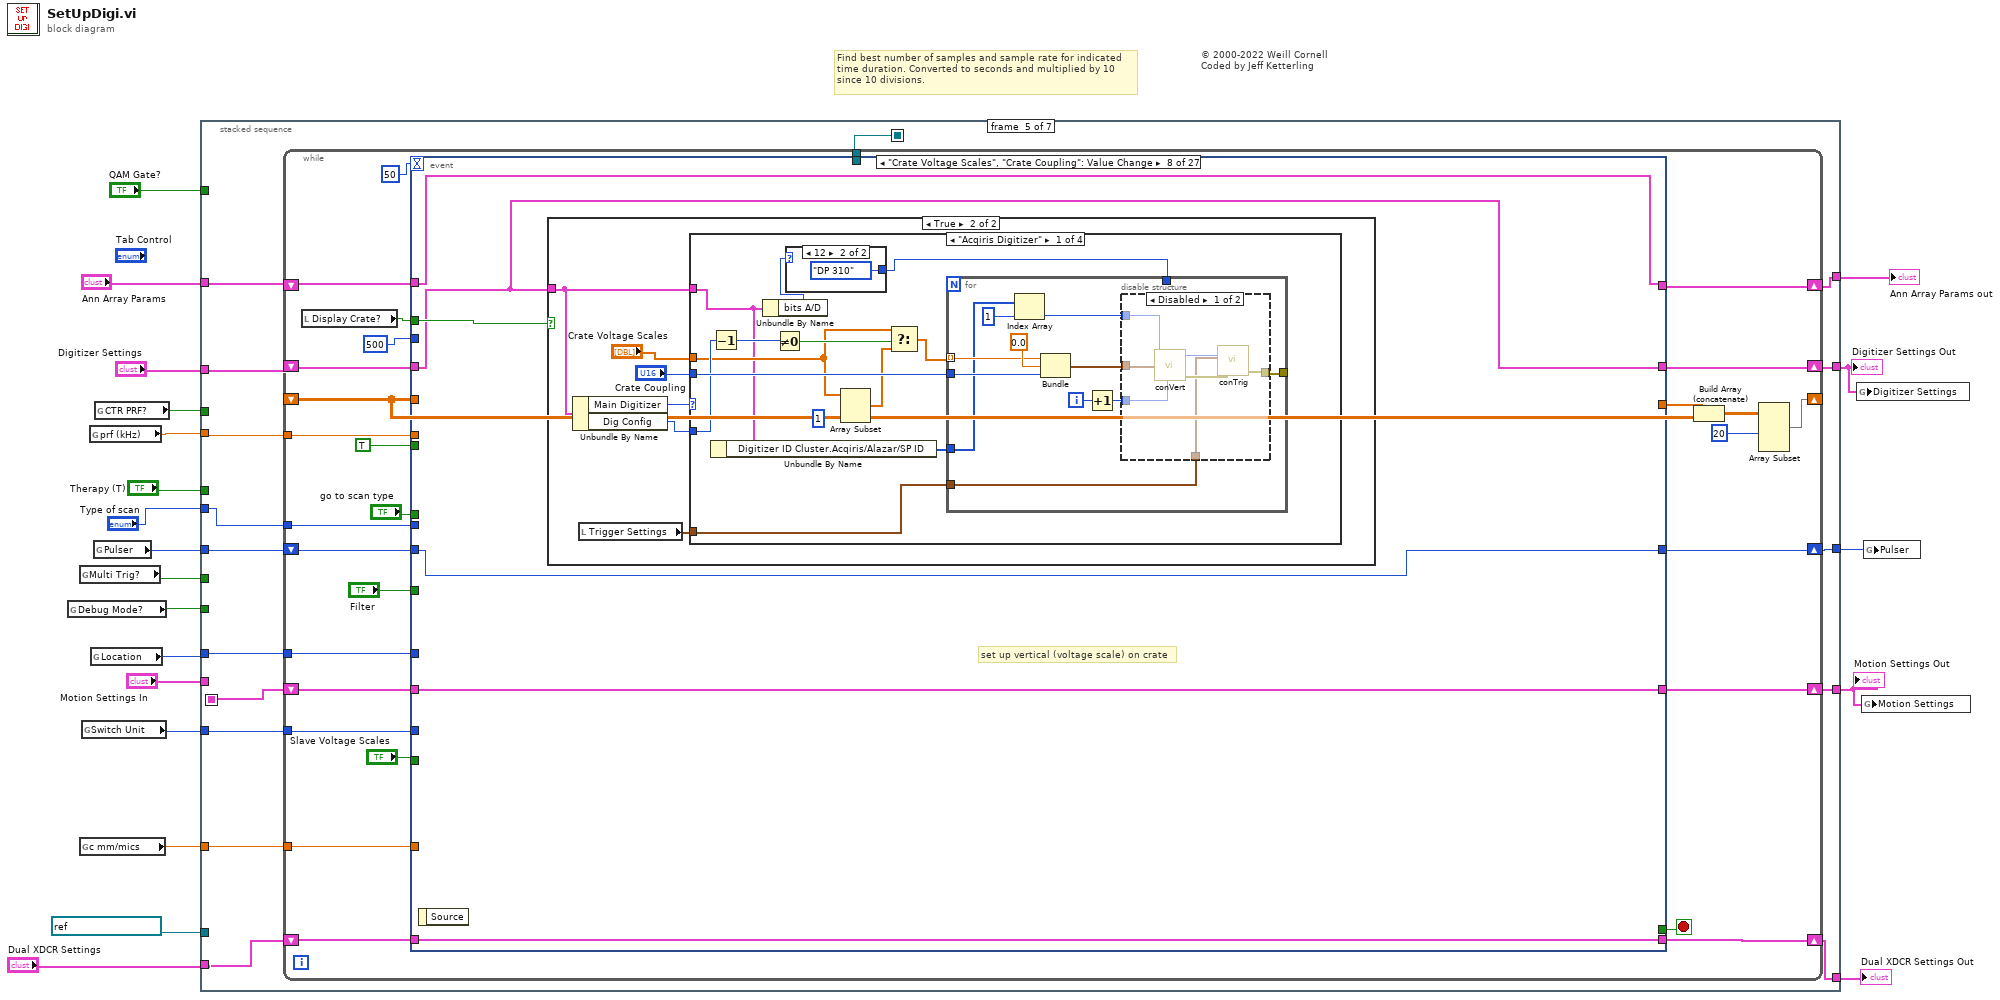
[diagram p0: block diagram]
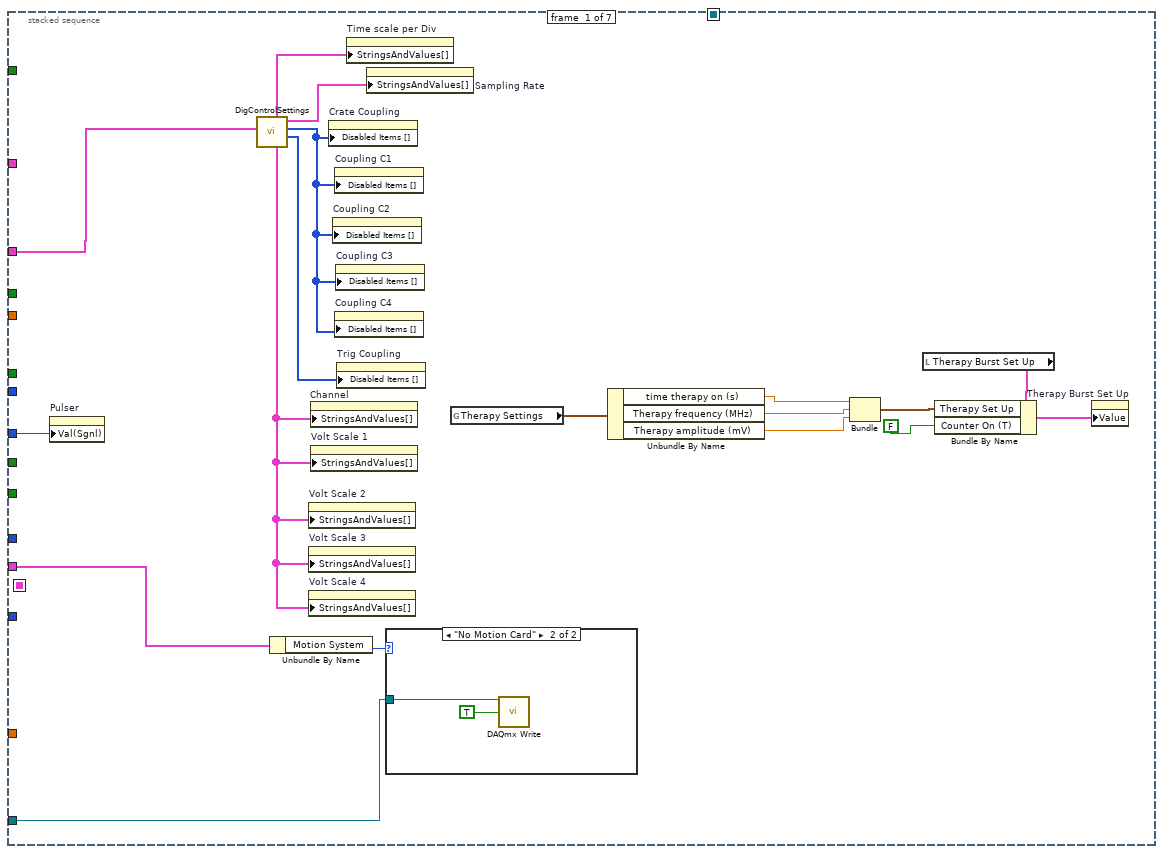
[diagram p2: hidden frame]
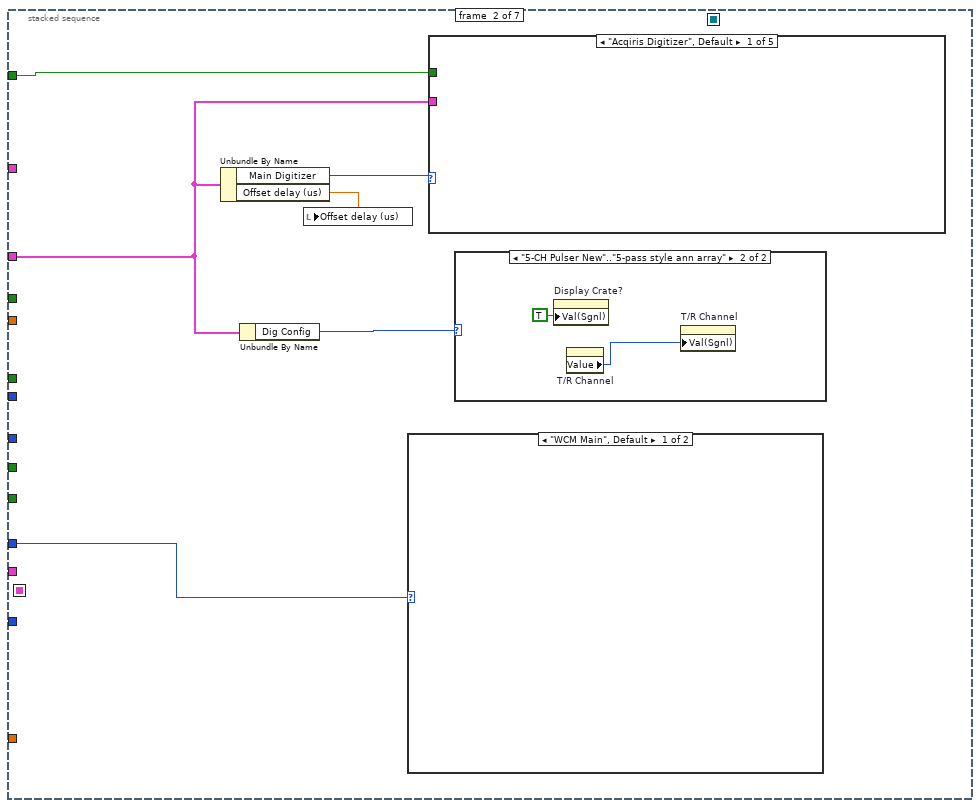
[diagram p4: hidden frame]
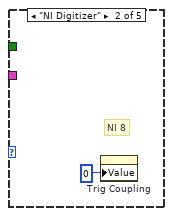
[diagram p5: hidden frame]
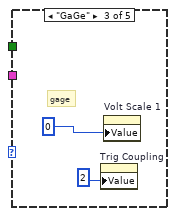
[diagram p6: hidden frame]
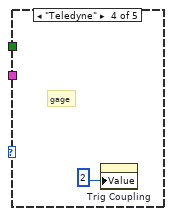
[diagram p7: hidden frame]
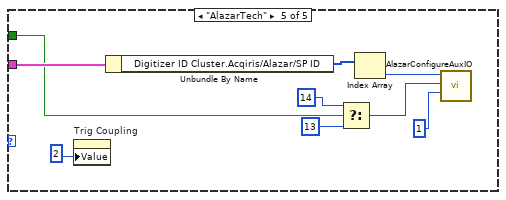
[diagram p8: hidden frame]
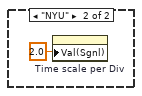
[diagram p9: hidden frame]
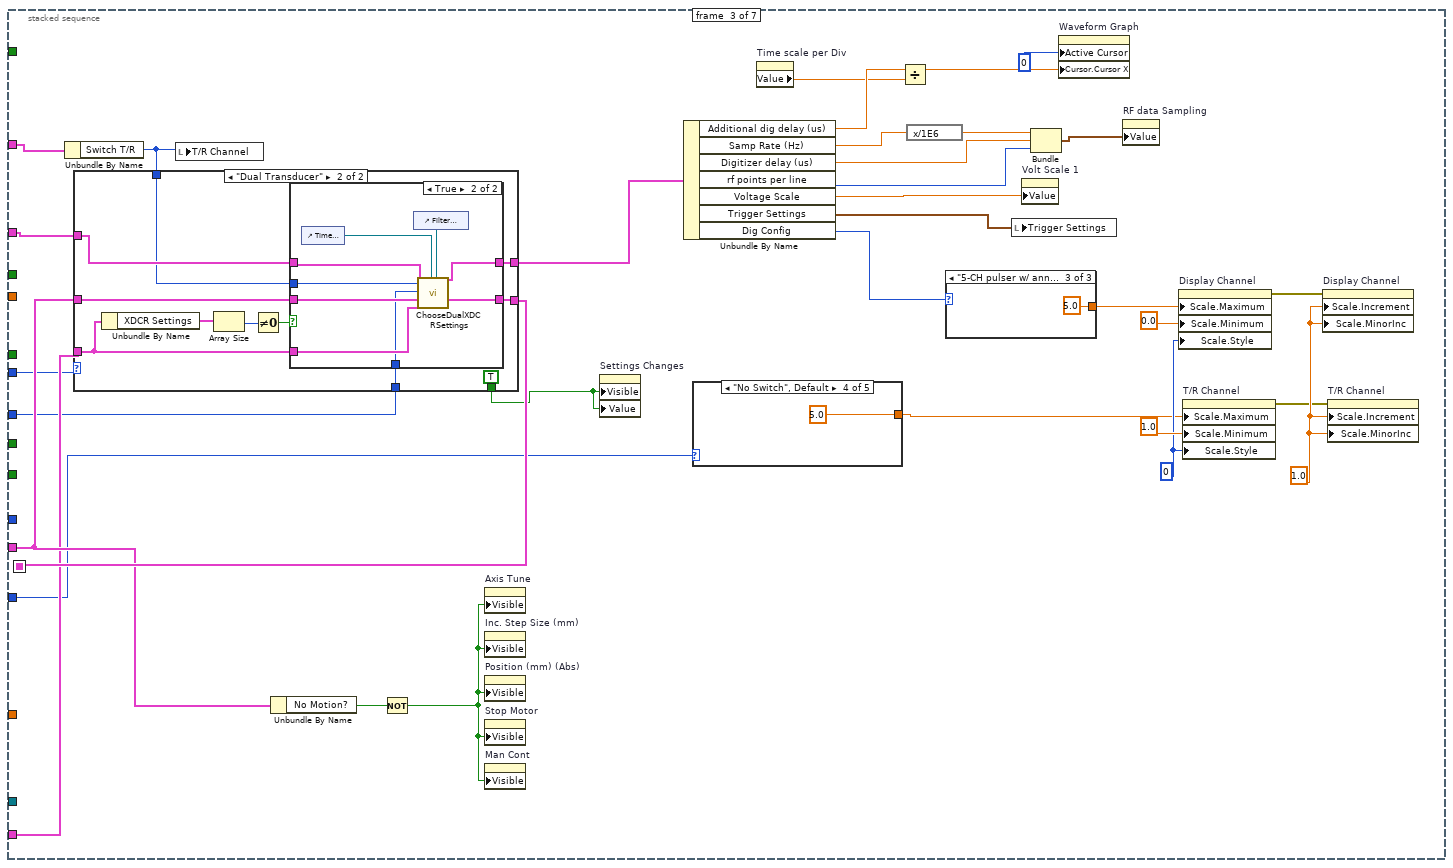
[diagram p11: hidden frame]
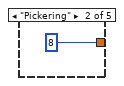
[diagram p13: hidden frame]
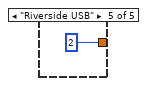
[diagram p15: hidden frame]
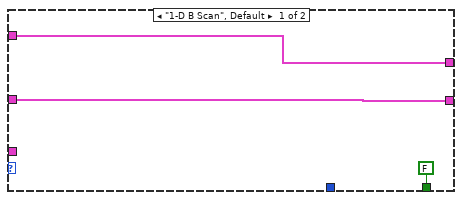
[diagram p16: hidden frame]
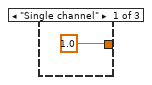
[diagram p18: hidden frame]
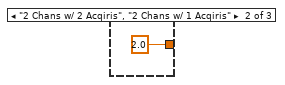
[diagram p19: hidden frame]
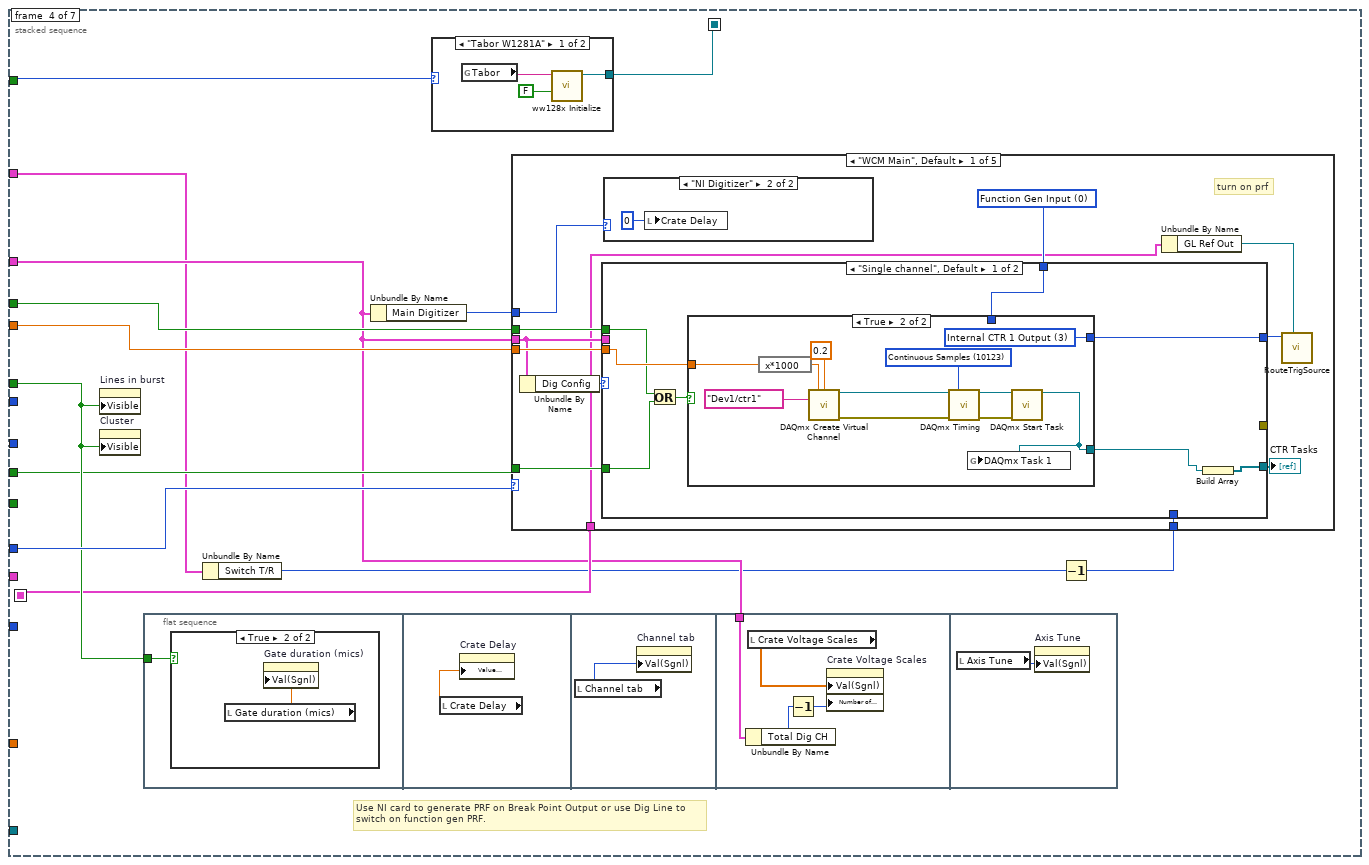
[diagram p20: hidden frame]
diagram:
  # "© 2000-2022 Weill Cornell\nCoded by Jeff Ketterling"
  # "Find best number of samples and sample rate for indicated time duration. Converted to seconds and multiplied by 10 since 10 divisions."
  n1 = global read "MotionGlobals.vi" "Debug Mode?"() -> (w7:bool)
  n2 = global read "MotionGlobals.vi" "Multi Trig?"() -> (w20:bool)
  n3 = global read "MotionGlobals.vi" "c mm/mics"() -> (w4:sgl)
  n4 = global read "SwitchGlobals.vi" "Switch Unit"() -> (w14:T40)
  n5 = global read "PulserGlobals.vi" "prf (kHz)"() -> (w15:dbl)
  n6 = global read "MotionGlobals.vi" "Location"() -> (w2:T41)
  n7 = global read "PulserGlobals.vi" "Pulser"() -> (w13:T39)
  n8 = global read "MotionGlobals.vi" "CTR PRF?"() -> (w19:bool)
  n9 = stacked-sequence {
    seq-local: [_ _ _ w139 _ _ _] -> [_ _ _ _ w263 _ w1656]
    seq-local: [_ _ w79 _ _ _ _] -> [_ _ _ w131 w256 w1631 _]
    tunnel: "Therapy (T)" -> [_ _ _ w138 _ _ w1662]
    tunnel: w2 -> [_ w45 _ w140 w264 w1628 _]
    tunnel: w15 -> [_ _ _ w137 w262 _ _]
    tunnel: w14 -> [_ _ w67 _ w261 _ w1663]
    tunnel: w20 -> [_ _ _ w135 _ _ w1660]
    tunnel: w19 -> [_ _ _ w134 _ _ w1658]
    tunnel: refnum<k21> "QuantFlipFlop" ("task/channels in") -> [w39 _ _ _ _ w1634 _]
    tunnel: w13 -> [w23 _ w68 w133 w260 _ _]
    tunnel: "Digitizer Settings" -> [w22 w43 w81 w130 w259 w1633 _]
    tunnel: [_ _ _ _ w258 _ _] -> w12
    tunnel: "Motion Settings In" -> [w28 _ w72 _ _ _ _]
    tunnel: [_ _ _ _ w257 _ _] -> w16
    tunnel: "Dual XDCR Settings" -> [_ _ w69 _ w255 _ _]
    tunnel: [_ _ _ _ w254 _ _] -> w11
    tunnel: "Ann Array Params" -> [_ _ w78 w129 w253 _ _]
    tunnel: [_ _ _ _ w252 _ _] -> w9
    tunnel: [_ _ _ _ w251 _ _] -> w8
    tunnel: w7 -> [_ _ _ _ _ _ _]
    tunnel: "Type of scan" -> [_ _ w65 _ w250 _ _]
    tunnel: w4 -> [_ _ _ _ w249 _ _]
    tunnel: "QAM Gate?" -> [_ w42 _ _ _ w1627 _]
    frame #0 {
      n10 = property on="Pulser" class="Enum (strict)"("Val(Sgnl)"=w23) -> ()  [unwired: 2 in, 2 out]
      n11 = call "DigControlSettings.vi"("Digitizer Settings"=w22) -> ("Trig Coupling Disable"=w33:i32[], "Ch Coupling Disable"=w31:i32[], "Sampling Rates"=w32:T46, "Voltage Scale"=w29:T46, "Time Scale/Div"=w34:T46)  [unwired: 6 in]
      n12 = Unbundle By Name(w28) -> ("Motion System"=w30:T28)
      n13 = property on="Volt Scale 2" class="Ring (strict)"("StringsAndValues[]"=w29) -> ()  [unwired: 2 in, 2 out]
      n14 = property on="Volt Scale 3" class="Ring (strict)"("StringsAndValues[]"=w29) -> ()  [unwired: 2 in, 2 out]
      n15 = property on="Volt Scale 4" class="Ring (strict)"("StringsAndValues[]"=w29) -> ()  [unwired: 2 in, 2 out]
      n16 = property on="Channel" class="Ring (strict)"("StringsAndValues[]"=w29) -> ()  [unwired: 2 in, 2 out]
      n17 = property on="Volt Scale 1" class="Ring (strict)"("StringsAndValues[]"=w29) -> ()  [unwired: 2 in, 2 out]
      n18 = property on="Crate Coupling" class="Ring (strict)"("Disabled Items []"=w31) -> ()  [unwired: 2 in, 2 out]
      n19 = property on="Coupling C2" class="Ring (strict)"("Disabled Items []"=w31) -> ()  [unwired: 2 in, 2 out]
      n20 = property on="Coupling C1" class="Ring (strict)"("Disabled Items []"=w31) -> ()  [unwired: 2 in, 2 out]
      n21 = property on="Coupling C4" class="Ring (strict)"("Disabled Items []"=w31) -> ()  [unwired: 2 in, 2 out]
      n22 = property on="Coupling C3" class="Ring (strict)"("Disabled Items []"=w31) -> ()  [unwired: 2 in, 2 out]
      n23 = property on="Trig Coupling" class="Ring (strict)"("Disabled Items []"=w33) -> ()  [unwired: 2 in, 2 out]
      n24 = property on="Time scale per Div" class="Ring (strict)"("StringsAndValues[]"=w34) -> ()  [unwired: 2 in, 2 out]
      n25 = property on="Sampling Rate" class="Ring (strict)"("StringsAndValues[]"=w32) -> ()  [unwired: 2 in, 2 out]
      n26 = case shown="\"No Motion Card\"" w30 {
        tunnel: w39 -> [_ w40]
        frame "NI 735x", Default {
        }
        frame "No Motion Card" {
          n27 = call-poly <vilib>:"DAQmx Write.vi"("task/channels in"=w40, "data"=TRUE) -> ()  [unwired: 11 in, 3 out]
        }
      }
      n28 = global read "PulserGlobals.vi" "Therapy Settings"() -> (w27:T47)
      n29 = Unbundle By Name(w27) -> ("time therapy on (s)"=w26:dbl, "Therapy frequency (MHz)"=w25:dbl, "Therapy amplitude (mV)"=w24:dbl)
      n30 = Bundle("time therapy on (s)"=w26, "Therapy frequency (MHz)"=w25, "Therapy amplitude (mV)"=w24) -> (w36:T48)  [unwired: 1 in]
      n31 = local read "Therapy Burst Set Up"() -> (w37:T38)
      n32 = Bundle By Name(cluster=w37, "Therapy Set Up"=w36, "Counter On (T)"=FALSE) -> (w35:T38)
      n33 = property on="Therapy Burst Set Up" class="Clust (strict)"("Value"=w35) -> ()  [unwired: 2 in, 2 out]
    }
    frame #1 {
      n34 = Unbundle By Name(w43) -> ("Main Digitizer"=w44:T32, "Offset delay (us)"=w46:dbl)
      n35 = Unbundle By Name(w43) -> ("Dig Config"=w47:T33)
      n36 = local write "Offset delay (us)"(w46) -> ()
      n37 = case shown="\"WCM Main\", Default" w45 {
        frame "WCM Main", Default {
        }
        frame "NYU" {
          n38 = property on="Time scale per Div" class="Ring (strict)"("Val(Sgnl)"=2.0 ("Value (Signaling)")) -> ()  [unwired: 2 in, 2 out]
        }
      }
      n39 = case shown="\"Acqiris Digitizer\", Default" w44 {
        tunnel: w43 -> [_ _ _ _ w57]
        tunnel: w42 -> [_ _ _ _ w54]
        frame "Acqiris Digitizer", Default {
        }
        frame "NI Digitizer" {
          # "NI 8"
          n40 = property on="Trig Coupling" class="Ring (strict)"("Value"=u16 0) -> ()  [unwired: 2 in, 2 out]
        }
        frame "GaGe" {
          # "gage"
          n41 = property on="Trig Coupling" class="Ring (strict)"("Value"=u16 2) -> ()  [unwired: 2 in, 2 out]
          n42 = property on="Volt Scale 1" class="Ring (strict)"("Value"=0) -> ()  [unwired: 2 in, 2 out]
        }
        frame "Teledyne" {
          # "gage"
          n43 = property on="Trig Coupling" class="Ring (strict)"("Value"=u16 2) -> ()  [unwired: 2 in, 2 out]
        }
        frame "AlazarTech" {
          n44 = property on="Trig Coupling" class="Ring (strict)"("Value"=u16 2) -> ()  [unwired: 2 in, 2 out]
          n45 = Unbundle By Name(w57) -> ("Digitizer ID Cluster.Acqiris/Alazar/SP ID"=w59:u32[])
          n46 = Select(t=u32 14, s=w54, f=u32 13) -> (s? t:f=w53:u32)
          n47 = Index Array(array=w59) -> (element=w58:u32)  [unwired: 1 in]
          n48 = call "AlazarConfigureAuxIO.vi"("Parameter"=u32 1, "Mode"=w53, "Handle"=w58) -> ()  [unwired: 1 in, 3 out]
        }
      }
      n49 = case shown="\"5-CH Pulser New\"..\"5-pass style ann array\"" w47 {
        frame "Single channel", Default {
        }
        frame "5-CH Pulser New".."5-pass style ann array" {
          n50 = property on="Display Crate?" class="Bool (strict)"("Val(Sgnl)"=TRUE ("Value (Signaling)")) -> ()  [unwired: 2 in, 2 out]
          n51 = property on="T/R Channel" class="Slide (strict)"() -> ("Value"=w62:u32)  [unwired: 2 in, 2 out]
          n52 = property on="T/R Channel" class="Slide (strict)"("Val(Sgnl)"=w62) -> ()  [unwired: 2 in, 2 out]
        }
      }
    }
    frame #2 {
      w89 = 1.0 ("Scale.Range:Minor Increment")
      w83 = u8 0 ("Scale.Style")
      n53 = Unbundle By Name(w78) -> ("Switch T/R"=w77:i16)
      n54 = case shown="\"Dual Transducer\"" w65 {
        tunnel: w81 -> [w102 w113]
        tunnel: [w102 w112] -> w80
        tunnel: w72 -> [w101 w111]
        tunnel: [w101 w110] -> w79
        tunnel: w77 -> [_ w109]
        tunnel: w69 -> [_ w105]
        tunnel: w68 -> [_ w104]
        tunnel: [FALSE ("Visible") TRUE ("Visible")] -> w64
        frame "1-D B Scan", Default {
        }
        frame "Dual Transducer" {
          n55 = Unbundle By Name(w105) -> ("XDCR Settings"=w107:T4[])
          n56 = Array Size(array=w107) -> (size(s)=w108:i32)
          n57 = Not Equal To 0?(x=w108) -> (x != 0?=w106:bool)
          n58 = case shown="True" w106 {
            tunnel: w113 -> [w115 w124]
            tunnel: [w115 w123] -> w112
            tunnel: w111 -> [w114 w122]
            tunnel: [w114 w121] -> w110
            tunnel: w109 -> [_ w120]
            tunnel: w105 -> [_ w119]
            tunnel: w104 -> [_ w117]
            frame False {
            }
            frame True {
              n59 = control-ref of="Time scale per Div"() -> (w118:refnum<vi>)
              n60 = control-ref of="Filter Prameters"() -> (w116:refnum<vi>)
              n61 = call "ChooseDualXDCRSettings.vi"("Digitizer Settings in"=w124, "Switch T/R"=w120, "Pulser"=w117, "Motion Settings in"=w122, "Dual XDCR Settings"=w119, "Time scale per Div Ref"=w118, "Filter Parameters Ref"=w116) -> ("Digitizer Settings"=w123:T31, "Motion Settings"=w121:T27)  [unwired: 18 in, 1 out]
            }
          }
        }
      }
      n62 = local write "T/R Channel"(w77) -> ()
      n63 = Unbundle By Name(w72) -> ("No Motion?"=w71:bool)
      n64 = Not(x=w71) -> (.not. x?=w70:bool)
      n65 = property on="Axis Tune" class="RadioBtnsControl (strict)"("Visible"=w70) -> ()  [unwired: 2 in, 2 out]
      n66 = property on="Inc. Step Size (mm)" class="DigNum (strict)"("Visible"=w70) -> ()  [unwired: 2 in, 2 out]
      n67 = property on="Position (mm) (Abs)" class="DigNum (strict)"("Visible"=w70) -> ()  [unwired: 2 in, 2 out]
      n68 = property on="Stop Motor" class="Bool"("Visible"=w70) -> ()  [unwired: 2 in, 2 out]
      n69 = property on="Man Cont" class="Bool"("Visible"=w70) -> ()  [unwired: 2 in, 2 out]
      n70 = property on="Settings Changes" class="Bool (strict)"("Visible"=w64, "Value"=w64) -> ()  [unwired: 2 in, 2 out]
      n71 = Unbundle By Name(w80) -> ("Additional dig delay (us)"=w75:dbl, "Samp Rate (Hz)"=w94:dbl, "Digitizer delay (us)"=w93:dbl, "rf points per line"=w92:i32, "Voltage Scale"=w91:dbl, "Trigger Settings"=w90:T37, "Dig Config"=w82:T33)
      n72 = case shown="\"No Switch\", Default" w67 {
        tunnel: [_ 8 _ 5.0 2] -> w66
        frame "Cytex" {
        }
        frame "Pickering" {
        }
        frame "NI Switch" {
        }
        frame "No Switch", Default {
        }
        frame "Riverside USB" {
        }
      }
      n73 = property on="Time scale per Div" class="Ring (strict)"() -> ("Value"=w73:dbl)  [unwired: 2 in, 2 out]
      n74 = Divide(x=w75, y=w73) -> (x/y=w74:dbl)
      n75 = expression code="x/1E6"(w94) -> (w96:dbl)
      n76 = case shown="\"5-CH pulser w/ ann array\", Default" w82 {
        tunnel: [1.0 2.0 5.0] -> w86
        frame "Single channel" {
        }
        frame "2 Chans w/ 2 Acqiris", "2 Chans w/ 1 Acqiris" {
        }
        frame "5-CH pulser w/ ann array", Default {
        }
      }
      n77 = local write "Trigger Settings"(w90) -> ()
      n78 = property on="Volt Scale 1" class="Ring (strict)"("Value"=w91) -> ()  [unwired: 2 in, 2 out]
      n79 = Bundle("Samp Rate (Hz)"=w96, "Digitizer delay (us)"=w93, "rf points per line"=w92) -> (w95:T49)  [unwired: 1 in]
      n80 = property on="Waveform Graph" class="WFGraph (strict)"("Active Cursor"=u32 0, "Cursor.Cursor X"=w74) -> ()  [unwired: 2 in, 2 out]
      n81 = property on="RF data Sampling" class="Clust (strict)"("Value"=w95) -> ()  [unwired: 2 in, 2 out]
      n82 = property on="Display Channel" class="Slide (strict)"("Scale.Maximum"=w86, "Scale.Minimum"=0.0, "Scale.Style"=w83) -> (error out=w88:errorcluster)  [unwired: 2 in, 1 out]
      n83 = property on="T/R Channel" class="Slide (strict)"("Scale.Maximum"=w66, "Scale.Minimum"=1.0, "Scale.Style"=w83) -> (error out=w87:errorcluster)  [unwired: 2 in, 1 out]
      n84 = property on="Display Channel" class="Slide (strict)"(error in=w88, "Scale.Increment"=w89, "Scale.MinorInc"=w89) -> ()  [unwired: 1 in, 2 out]
      n85 = property on="T/R Channel" class="Slide (strict)"(error in=w87, "Scale.Increment"=w89, "Scale.MinorInc"=w89) -> ()  [unwired: 1 in, 2 out]
    }
    frame #3 {
      # "Use NI card to generate PRF on Break Point Output or use Dig Line to switch on function gen PRF."
      n86 = property on="Lines in burst" class="DigNum (strict)"("Visible"=w138) -> ()  [unwired: 2 in, 2 out]
      n87 = property on="Cluster" class="Clust (strict)"("Visible"=w138) -> ()  [unwired: 2 in, 2 out]
      n88 = flat-sequence {
        tunnel: w138 -> [w144]
        tunnel: w130 -> [w149]
        frame #0 {
          n89 = case shown="True" w144 {
            frame False {
            }
            frame True {
              n90 = local read "Gate duration (mics)"() -> (w145:dbl)
              n91 = property on="Gate duration (mics)" class="DigNum (strict)"("Val(Sgnl)"=w145) -> ()  [unwired: 2 in, 2 out]
            }
          }
        }
        frame #1 {
          n92 = local read "Crate Delay"() -> (w146:dbl)
          n93 = property on="Crate Delay" class="DigNum (strict)"("Value (Signaling)"=w146) -> ()  [unwired: 2 in, 2 out]
        }
        frame #2 {
          n94 = local read "Channel tab"() -> (w147:enum32{"C1", "C2", "C3", "C4"})
          n95 = property on="Channel tab" class="TabCtl (strict)"("Val(Sgnl)"=w147) -> ()  [unwired: 2 in, 2 out]
        }
        frame #3 {
          n96 = Unbundle By Name(w149) -> ("Total Dig CH"=w150:i32)
          n97 = local read "Crate Voltage Scales"() -> (w151:dbl[])
          n98 = Decrement(x=w150) -> (x-1=w148:i32)
          n99 = property on="Crate Voltage Scales" class="Arr (strict)"("Val(Sgnl)"=w151, "Number of Columns"=w148) -> ()  [unwired: 2 in, 2 out]
        }
        frame #4 {
          n100 = local read "Axis Tune"() -> (w152:enum32{"Axis 1", "Axis 2", "Axis 3", "Axis 4"})
          n101 = property on="Axis Tune" class="RadioBtnsControl (strict)"("Val(Sgnl)"=w152) -> ()  [unwired: 2 in, 2 out]
        }
      }
      n102 = Unbundle By Name(w129) -> ("Switch T/R"=w128:i16)
      n103 = Unbundle By Name(w130) -> ("Main Digitizer"=w132:T32)
      n104 = case shown="\"Tabor W1281A\"" w133 {
        tunnel: [w142 _] -> w139
        frame "Tabor W1281A" {
          n105 = global read "PulserGlobals.vi" "Tabor"() -> (w141:string)
          n106 = call <instrlib>:"ww128x Initialize.vi"("reset device (Yes)"=FALSE ("reset device"), "resource name"=w141) -> ("instrument handle out"=w142:refnum<k15>)  [unwired: 2 in, 7 out]
        }
        frame "Pan 5900", Default {
        }
      }
      n107 = Decrement(x=w128) -> (x-1=w136:i16)
      n108 = case shown="\"WCM Main\", Default" w140 {
        tunnel: w132 -> [w164 _ _ _ w240]
        tunnel: w137 -> [w163 _ _ _ _]
        tunnel: w136 -> [w162 _ _ _ w239]
        tunnel: w135 -> [w161 _ _ _ _]
        tunnel: w134 -> [w160 _ _ _ _]
        tunnel: w130 -> [w156 _ _ _ _]
        tunnel: w131 -> [w154 w218 _ w228 _]
        frame "WCM Main", Default {
          w158 = u16 0 items=["Function Gen Input", "Motion Trig", "Internal RT Motion Trig", "Internal CTR 1 Output"] ("Trig Source")
          # "turn on prf"
          n109 = Unbundle By Name(w156) -> ("Dig Config"=w155:T33)
          n110 = case shown="\"Single channel\", Default" w155 {
            tunnel: w163 -> [w172 w193]
            tunnel: w162 -> [_ w192]
            tunnel: [w171 w188] -> w157
            tunnel: w158 -> [w170 w188]
            tunnel: w161 -> [w168 _]
            tunnel: w160 -> [w167 _]
            tunnel: [w166 w189] -> w159
            tunnel: w156 -> [_ w187]
            tunnel: [_ w185] -> _
            frame "Single channel", Default {
              n111 = Or(x=w167, y=w168) -> (x .or. y?=w169:bool)
              n112 = case shown="True" w169 {
                tunnel: w172 -> [_ w179]
                tunnel: [w173 w176] -> w171
                tunnel: w170 -> [w173 _]
                tunnel: [_ w174] -> w165
                frame False {
                }
                frame True {
                  w176 = u16 3 items=["Function Gen Input", "Motion Trig", "Internal RT Motion Trig", "Internal CTR 1 Output"] ("Trig Source")
                  w181 = 10123 items=["Finite Samples"=10178, "Continuous Samples"=10123, "Hardware Timed Single Point"=12522] ("sample mode")
                  n113 = expression code="x*1000"(w179) -> (w180:dbl)
                  n114 = call-poly <vilib>:"DAQmx Create Virtual Channel.vi"("frequency"=w180, "duty cycle"=0.2, "counter"=tag "Dev1/ctr1") -> ("task out"=w183:refnum<k21>, "error out"=w182:errorcluster)  [unwired: 6 in, 5 out]
                  n115 = call-poly <vilib>:"DAQmx Timing.vi"("task/channels in"=w183, "sample mode"=w181, "error in"=w182) -> ("task out"=w175:refnum<k21>, "error out"=w177:errorcluster)  [unwired: 11 in]
                  n116 = call <vilib>:"DAQmx Start Task.vi"("task/channels in"=w175, "error in"=w177) -> ("task out"=w174:refnum<k21>)  [unwired: 12 in, 1 out]
                  n117 = global write "MotionGlobals.vi" "DAQmx Task 1"(w174) -> ()
                }
              }
              n118 = Build Array(w165) -> (w166:refnum<k21>[])
            }
            frame "5-CH pulser w/ ann array" {
              n119 = Unbundle By Name(w187) -> ("Avg Num"=w186:i32)
              n120 = for {
                tunnel: [w196] -> w189 mode=indexing
                tunnel: tag[] ["Timer/ctr0", "Timer/ctr2", "Timer/ctr3", "Timer/ctr4", "Timer/ctr5"] -> [w197] mode=indexing
                tunnel: w193 -> [w195]
                tunnel: w186 -> [w194]
                n121 = case shown="-1" w194 {
                  tunnel: w197 -> [w205 w210]
                  tunnel: [w201 w209] -> w196
                  tunnel: w195 -> [w199 _]
                  frame 0, Default {
                    w200 = 10123 items=["Finite Samples"=10178, "Continuous Samples"=10123, "Hardware Timed Single Point"=12522] ("sample mode")
                    n122 = expression code="x*1000"(w199) -> (w198:dbl)
                    n123 = call-poly <vilib>:"DAQmx Create Virtual Channel.vi"("frequency"=w198, "duty cycle"=0.2, "counter"=w205) -> ("task out"=w203:refnum<k21>, "error out"=w202:errorcluster)  [unwired: 6 in, 5 out]
                    n124 = call-poly <vilib>:"DAQmx Timing.vi"("task/channels in"=w203, "sample mode"=w200, "error in"=w202) -> ("task out"=w201:refnum<k21>)  [unwired: 11 in, 1 out]
                  }
                  frame -1 {
                    n125 = call-poly <vilib>:"DAQmx Create Virtual Channel.vi"("high time"=2e-06, "low time"=1.5e-07 ("duty cycle"), "counter"=w210) -> ("task out"=w213:refnum<k21>, "error out"=w212:errorcluster)  [unwired: 6 in, 5 out]
                    n126 = call-poly <vilib>:"DAQmx Trigger.vi"("task/channels in"=w213, "source"=tag "/Dev1/PFI9", "error in"=w212) -> ("task out"=w207:refnum<k21>, "error out"=w208:errorcluster)  [unwired: 11 in]
                    n127 = property class="DAQmx Trigger"(reference=w207, error in=w208, "Start.Retriggerable"=TRUE) -> (reference out=w209:refnum<k21>)  [unwired: 1 out]
                  }
                }
              }
              n128 = Index Array(array=w189, index=w192) -> (element=w191:refnum<k21>)
              n129 = call <vilib>:"DAQmx Start Task.vi"("task/channels in"=w191) -> ("error out"=w185:errorcluster)  [unwired: 13 in, 1 out]
            }
          }
          "CTR Tasks" <- w159
          n130 = case shown="\"NI Digitizer\"" w164 {
            frame "Acqiris Digitizer", Default {
            }
            frame "NI Digitizer" {
              n131 = local write "Crate Delay"(0) -> ()
            }
          }
          n132 = Unbundle By Name(w154) -> ("GL Ref Out"=w153:refnum<k7>)
          n133 = call "RouteTrigSource.vi"("Galil.IGalil"=w153, "Trig Source"=w157) -> ()  [unwired: 9 in, 1 out]
        }
        frame "Hawaii", "SERI GP" {
          n134 = Unbundle By Name(w218) -> ("Motion System"=w217:T28)
          n135 = case shown="\"Galil\"" w217 {
            tunnel: w218 -> [_ w219 w226]
            frame "MM3000", Default {
            }
            frame "NI 735x" {
              n136 = disable-structure shown="Disabled" {
                disable-tunnel: w219 -> [w221 _]
                frame Disabled {
                  n137 = Unbundle By Name(w221) -> ("Motion Bd ID"=w220:u8)
                  n138 = call <vilib>:"Run Program.flx"("Program (1)"=3, "Board ID"=w220) -> ()  [unwired: 1 in, 6 out]
                }
                frame Enabled {
                }
              }
            }
            frame "Galil" {
              n139 = Unbundle By Name(w226) -> ("GL Ref Out"=w225:refnum<k7>)
              n140 = call "GL Command Set.vi"("Command"=Command_Menu."Execute", "Text Input"="#PRF", "Galil.IGalil"=w225) -> ()  [unwired: 4 in, 5 out]
            }
          }
        }
        frame "Columbia MM3000" {
          (unwired) "SB3"
          # "Old send command mm2k dend command"
        }
        frame "UHI Allen" {
          n141 = Unbundle By Name(w228) -> ("ESP VISA"=w227:refnum<visa-resource-name>)
          n142 = call <instrlib>:"Get DIO Port AB Bit Status.vi"("VISA resource name"=w227) -> ("error out"=w230:errorcluster, "DIO Port A status"=w233:T50, "VISA resource name out"=w229:refnum<visa-resource-name>)  [unwired: 4 in]
          n143 = Bundle By Name(cluster=w233, "Port A bit-1 at logic level"=FALSE) -> (w231:T50)
          n144 = call <instrlib>:"Set DIO Port AB Bit Status.vi"("error in (no error)"=w230, "DIO Port status"=w231, "VISA resource name"=w229) -> ()  [unwired: 3 in, 2 out]
        }
        frame "CUMC RT" {
          w235 = 0.8 items=["8 V"=8.0, "4 V"=4.0, "2 V"=2.0, "800 mV"=0.8, "400 mV"=0.4, "200 mV"=0.2] ("Voltage Scale 1")
          n145 = case shown="\"NI Digitizer\"" w240 {
            frame "Acqiris Digitizer", Default {
            }
            frame "NI Digitizer" {
              n146 = local write "Crate Delay"(0) -> ()
            }
          }
          n147 = for {
            tunnel: [w246] -> w236 mode=indexing
            tunnel: tag[] ["Timer/ctr0", "Timer/ctr2", "Timer/ctr3", "Timer/ctr4", "Timer/ctr5"] -> [w247] mode=indexing
            w241 = 10123 items=["Finite Samples"=10178, "Continuous Samples"=10123, "Hardware Timed Single Point"=12522] ("sample mode")
            n148 = call-poly <vilib>:"DAQmx Create Virtual Channel.vi"("frequency"=1000.0 ("high time"), "duty cycle"=0.2, "counter"=w247) -> ("task out"=w243:refnum<k21>, "error out"=w242:errorcluster)  [unwired: 6 in, 5 out]
            n149 = call-poly <vilib>:"DAQmx Timing.vi"("task/channels in"=w243, "sample mode"=w241, "error in"=w242) -> ("task out"=w246:refnum<k21>)  [unwired: 11 in, 1 out]
          }
          n150 = property on="Sampling Rate" class="Ring (strict)"("Value"=125.0) -> ()  [unwired: 2 in, 2 out]
          n151 = property on="Volt Scale 1" class="Ring (strict)"("Value"=w235) -> ()  [unwired: 2 in, 2 out]
          n152 = local write "CTR Tasks"(w236) -> ()
          n153 = Index Array(array=w236, index=w239) -> (element=w237:refnum<k21>)
          n154 = call <vilib>:"DAQmx Start Task.vi"("task/channels in"=w237) -> ()  [unwired: 13 in, 2 out]
        }
      }
    }
    frame #4 {
      n155 = while {
        shift-left: _ -> [w286]
        shift-right: [w291] -> _
        tunnel: w264 -> [w284]
        tunnel: w263 -> [w288]
        tunnel: w262 -> [w282]
        tunnel: w261 -> [w281]
        shift-right: [w279] -> w258
        shift-left: w259 -> [w275]
        shift-right: [w277] -> w257
        shift-left: w256 -> [w278]
        shift-right: [w273] -> w254
        shift-left: w255 -> [w274]
        shift-right: [w271] -> w252
        shift-left: w253 -> [w272]
        shift-right: [w270] -> w251
        shift-left: w260 -> [w280]
        tunnel: w250 -> [w268]
        tunnel: w249 -> [w267]
        stop <- w276 stop-if-true
        n156 = local read "Display Crate?"() -> (w285:bool)
        n157 = event shown="[7] \"Crate Voltage Scales\", \"Crate Coupling\": Value Change" {
          selector: _ -> [_ _ _ _ _ _ _ _ _ _ _ _ _ _ _ _ _ _ _ _ _ _ _ _ _ _ _]
          dyn-events: _ -> [_ _ _ _ _ _ _ _ _ _ _ _ _ _ _ _ _ _ _ _ _ _ _ _ _ _ _]
          timeout: 50 -> [_ _ _ _ _ _ _ _ _ _ _ _ _ _ _ _ _ _ _ _ _ _ _ _ _ _ _]
          tunnel: w284 -> [_ _ _ _ _ _ _ _ _ _ w1267 _ _ _ _ _ _ _ _ _ _ _ _ _ _ _ _]
          tunnel: "go to scan type" -> [w300 _ _ _ _ _ _ _ _ _ _ _ _ _ _ _ _ _ _ w1546 _ _ _ _ _ _ _]
          tunnel: w280 -> [w302 w765 w996 w1001 w1015 w1035 w1044 w1144 w1236 w1247 w1256 w1396 _ w1430 w1434 w1439 w1461 w1483 w1514 w1539 w1558 w1574 w1589 w1599 w1609 w1614 w1620]
          tunnel: w288 -> [_ _ _ _ _ _ _ _ _ _ _ w1394 _ _ _ _ _ _ _ _ _ w1582 _ _ _ _ _]
          tunnel: w286 -> [w309 _ _ _ _ _ _ _ _ _ _ _ _ _ _ _ _ _ _ _ _ _ _ _ _ _ _]
          tunnel: [w308 _ _ _ _ _ _ _ _ _ _ _ _ _ _ _ _ _ _ _ _ _ _ _ _ _ _] -> w293
          tunnel: w285 -> [w307 w764 _ _ _ _ _ w1149 _ _ _ _ _ _ _ _ _ _ _ _ _ _ _ _ _ _ _]
          tunnel: "Slave Voltage Scales" -> [_ _ _ _ _ _ w1060 _ _ _ _ _ _ _ _ _ _ _ _ _ _ _ _ _ _ _ _]
          tunnel: w282 -> [_ _ _ _ _ _ _ _ _ _ w1254 _ _ _ _ _ _ _ _ _ w1563 _ _ _ _ _ _]
          tunnel: w281 -> [_ w762 _ _ _ w1039 w1048 _ _ _ w1266 w1401 _ _ _ _ _ _ _ _ _ _ _ _ _ _ _]
          tunnel: w275 -> [w299 w763 w1000 w1008 w1034 w1042 w1046 w1148 w1241 w1251 w1265 w1399 w1421 w1429 w1438 w1445 w1467 w1487 w1518 w1543 w1562 w1578 w1593 w1603 w1613 w1618 w1626]
          tunnel: [w298 w759 w1000 w1008 w1034 w1042 w1050 w1148 w1241 w1251 w1264 w1399 w1419 w1427 w1438 w1445 w1467 w1487 w1518 w1543 w1562 w1578 w1593 w1603 w1613 w1618 w1626] -> w279
          tunnel: w278 -> [w296 w760 w999 w1014 w1017 w1041 w1051 w1147 w1240 w1250 w1262 w1400 w1426 w1433 w1437 w1444 w1466 w1474 w1513 w1542 w1561 w1577 w1592 w1602 w1612 w1617 w1625]
          tunnel: [w296 w758 w999 w1014 w1017 w1041 w1051 w1147 w1240 w1250 w1261 w1400 w1426 w1433 w1437 w1442 w1464 w1474 w1517 w1542 w1561 w1577 w1592 w1602 w1612 w1617 w1625] -> w277
          tunnel: [_ _ _ _ w1025 _ _ _ _ _ _ _ _ _ _ _ _ _ _ _ _ _ _ _ _ _ w1624] -> w276
          tunnel: w274 -> [w305 w757 w998 w1013 w1031 w1038 w1049 w1146 w1238 w1249 w1260 w1398 w1425 w1432 w1436 w1441 w1463 w1485 w1516 w1541 w1560 w1576 w1591 w1601 w1611 w1616 w1623]
          tunnel: [w305 w756 w998 w1013 w1031 w1037 w1043 w1146 w1238 w1249 w1260 w1397 w1425 w1432 w1436 w1441 w1463 w1485 w1516 w1541 w1560 w1576 w1591 w1601 w1611 w1616 w1623] -> w273
          tunnel: w272 -> [w303 w753 w997 w1012 w1024 w1036 w1045 w1145 w1237 w1248 w1259 w1395 w1424 w1431 w1435 w1440 w1462 w1484 w1515 w1540 w1559 w1575 w1590 w1600 w1610 w1615 w1621]
          tunnel: [w303 w753 w997 w1012 w1024 w1036 w1045 w1145 w1237 w1248 w1257 w1395 w1424 w1431 w1435 w1440 w1462 w1484 w1515 w1540 w1559 w1575 w1590 w1600 w1610 w1615 w1621] -> w271
          tunnel: [w302 w765 w996 w1001 w1015 w1035 w1044 w1144 w1236 w1247 w1256 w1396 "Pulser" w1430 w1434 w1439 w1461 w1483 w1514 w1539 w1558 w1574 w1589 w1599 w1609 w1614 w1620] -> w270
          tunnel: "Filter" -> [w301 _ _ _ _ _ _ _ _ _ _ _ _ _ _ _ _ _ _ _ _ _ _ _ _ _ _]
          tunnel: w268 -> [_ _ _ _ _ _ _ _ _ _ w1255 _ _ _ _ _ _ _ _ _ _ _ _ _ _ _ _]
          tunnel: w267 -> [_ w754 w992 _ _ _ _ _ _ _ _ _ _ _ _ _ _ _ _ _ _ _ _ _ _ _ _]
          tunnel: TRUE -> [w295 w752 _ _ _ _ _ _ _ _ _ _ _ _ _ _ _ _ _ _ _ _ _ _ _ _ _]
          tunnel: 500 ("Channels") -> [w294 w751 _ _ _ _ _ _ _ _ _ _ _ _ _ _ _ _ _ _ _ _ _ _ _ _ _]
          event Timeout {
            n158 = event-data() -> ()  [unwired: 2 out]
            n159 = local read "Nominal Samples"() -> (w306:i32)
            n160 = Unbundle By Name(w299) -> ("Main Digitizer"=w304:T32)
            n161 = property on="Norm Spect?" class="Bool (strict)"("Visible"=w300) -> ()  [unwired: 2 in, 2 out]
            n162 = local read "AlazarCluster"() -> (w297:T1)
            n163 = stacked-sequence {
              seq-local: [_ w461 _ _] -> [_ _ w615 _]
              seq-local: [w311 _ _ _] -> [_ w448 w608 _]
              seq-local: [_ w449 _ _] -> [_ _ w609 _]
              tunnel: w307 -> [w317 _ w617 _]
              tunnel: w309 -> [_ w452 _ _]
              tunnel: [_ w465 _ _] -> w308
              tunnel: w300 -> [_ w464 w616 _]
              tunnel: w306 -> [_ w460 w614 _]
              tunnel: w304 -> [w314 w463 w613 _]
              tunnel: w299 -> [w312 w456 w612 w744]
              tunnel: w301 -> [_ w457 w611 _]
              tunnel: [w312 _ _ _] -> w298
              tunnel: w297 -> [_ w450 w610 _]
              tunnel: w295 -> [w310 _ _ w743]
              tunnel: w294 -> [_ w447 _ _]
              frame #0 {
                n164 = case shown="\"Acqiris Digitizer\", Default" w314 {
                  tunnel: w317 -> [w320 w363 w391 _ _]
                  tunnel: [w319 w361 w388 _ w430] -> w313
                  tunnel: w312 -> [w318 w360 w385 w418 w440]
                  tunnel: [_ _ _ w414 _] -> w311
                  tunnel: [_ _ _ w404 _] -> _
                  tunnel: [_ _ _ w403 _] -> _
                  tunnel: [_ _ _ w402 _] -> _
                  tunnel: w310 -> [_ _ _ w401 _]
                  frame "Acqiris Digitizer", Default {
                    n165 = disable-structure shown="Disabled" {
                      disable-tunnel: w320 -> [w326 _]
                      disable-tunnel: [w322 _] -> w319
                      disable-tunnel: w318 -> [w321 _]
                      frame Disabled {
                        n166 = flat-sequence {
                          tunnel: w326 -> [w336]
                          tunnel: [w333] -> w332
                          tunnel: [w337] -> w331
                          tunnel: [w335] -> w330
                          tunnel: w321 -> [w334]
                          tunnel: w332 -> [w347]
                          tunnel: w331 -> [w346]
                          tunnel: [w347] -> w329
                          tunnel: [w346] -> w328
                          tunnel: [w344] -> w327
                          tunnel: w330 -> [w344]
                          tunnel: w329 -> [w349]
                          tunnel: w328 -> [w352]
                          tunnel: [w351] -> w323
                          tunnel: [w350] -> w324
                          tunnel: w327 -> [w348]
                          frame #0 {
                            # "Start Acq"
                            n167 = Unbundle By Name(w334) -> ("Digitizer ID Cluster.Acqiris/Alazar/SP ID"=w335:u32[])
                            n168 = Select(t=2, s=w336, f=1) -> (s? t:f=w333:i32)
                            n169 = for {
                              N: w333 -> [_]
                              tunnel: [w343] -> w337
                              tunnel: w335 -> [w341] mode=indexing
                              n170 = call <instrlib>:"Stop Acquisition.vi"("Instrument ID"=w341) -> ("error out"=w342:errorcluster, "dup Instrument ID"=w340:u32)  [unwired: 1 in, 4 out]
                              n171 = call <instrlib>:"Start Acquisition.vi"("error in (no error)"=w342, "Instrument ID"=w340) -> ("error out"=w343:errorcluster)  [unwired: 2 in, 1 out]
                            }
                          }
                          frame #1 {
                            n172 = Wait (ms)(milliseconds to wait=10) -> ()  [unwired: 1 out]
                          }
                          frame #2 {
                            # "wait for end of acquistion"
                            n173 = for {
                              N: w349 -> [_]
                              tunnel: [w358] -> _
                              shift-right: [w357] -> w351
                              shift-left: w352 -> [w354]
                              tunnel: [w356] -> w350
                              tunnel: w348 -> [w355] mode=indexing
                              n174 = call "WaitForSegs.vi"("Acqiris ID"=w355, "lines per plane"=1, "error in"=w354, "Timeout"=500) -> ("dup Instrument ID"=w356:u32, "status"=w358:bool, "error out"=w357:errorcluster)  [unwired: 1 out]
                            }
                          }
                        }
                        n175 = call <instrlib>:"Error Message.vi"("Instrument ID"=w324, "Type of Dialog (1: OK Msg)"=i16 0, "error in (no error)"=w323) -> ("Error Message"=w322:string)  [unwired: 6 out]
                      }
                      frame Enabled {
                      }
                    }
                  }
                  frame "NI Digitizer" {
                    n176 = case shown="True" w363 {
                      tunnel: [w367 w371] -> w362
                      tunnel: w360 -> [w365 w369]
                      frame False {
                        n177 = Unbundle By Name(w365) -> ("Digitizer ID Cluster.NI Instr Handles"=w364:refnum<k15>[])
                        n178 = Index Array(array=w364) -> (element=w366:refnum<k15>)  [unwired: 1 in]
                        n179 = call <instrlib>:"niScope Initiate Acquisition.vi"("instrument handle"=w366) -> ("error out"=w367:errorcluster)  [unwired: 1 in, 13 out]
                      }
                      frame True {
                        # "Arm other cards"
                        n180 = Unbundle By Name(w369) -> ("Digitizer ID Cluster.NI Instr Handles"=w368:refnum<k15>[])
                        n181 = case shown="0, Default" 0 {
                          tunnel: [w373 w379] -> w371
                          tunnel: w368 -> [w372 w376]
                          frame 0, Default {
                            n182 = for {
                              tunnel: w372 -> [w374] mode=indexing
                              tunnel: [w375] -> w373
                              n183 = call <instrlib>:"niScope Initiate Acquisition.vi"("instrument handle"=w374) -> ("error out"=w375:errorcluster)  [unwired: 1 in, 13 out]
                            }
                          }
                          frame 4, 5 {
                            n184 = for {
                              tunnel: w376 -> [w384] mode=indexing
                              tunnel: [w383] -> w378 mode=indexing
                              tunnel: [w382] -> w377
                              n185 = call <instrlib>:"niScope Get Session Reference.vi"("instrument handle"=w384) -> ("session reference"=w383:refnum<k20>, "error out"=w382:errorcluster)  [unwired: 1 in, 12 out]
                            }
                            n186 = call <instrlib>:"niTClk Configure For Homogeneous Triggers.vi"("error in (no error)"=w377, "sessions"=w378) -> ("error out"=w380:errorcluster, "sessions out"=w381:refnum<k20>[])  [unwired: 8 out]
                            n187 = call <instrlib>:"niTClk Initiate.vi"("error in (no error)"=w380, "sessions"=w381) -> ("error out"=w379:errorcluster)  [unwired: 9 out]
                          }
                        }
                      }
                    }
                    n188 = Unbundle(w362) -> ("source"=w361:string)  [unwired: 2 out]
                  }
                  frame "GaGe" {
                    n189 = flat-sequence {
                      tunnel: w391 -> [_]
                      tunnel: w385 -> [w394]
                      tunnel: [w393] -> w390
                      tunnel: [w392] -> w386
                      tunnel: w390 -> [w397]
                      tunnel: [w397] -> w389
                      tunnel: [w395] -> w387
                      tunnel: w386 -> [w395]
                      tunnel: w389 -> [_]
                      tunnel: [w400] -> w388
                      tunnel: w387 -> [w398]
                      frame #0 {
                        # "Start Acq"
                        n190 = Unbundle By Name(w394) -> ("Digitizer ID Cluster.GaGe Handle"=w392:T51)
                        n191 = call "CsTool-CaptureFill.vi"("Handle Cluster"=w392) -> ("Error Code"=w393:i32)
                      }
                      frame #1 {
                        n192 = Wait (ms)(milliseconds to wait=u32 20) -> ()  [unwired: 1 out]
                      }
                      frame #2 {
                        # "wait for end of acquistion"
                        n193 = call "GaGe_TimeoutFill.vi"("TimeOut (s)"=sgl 0.5, "GaGe Handle"=w398) -> ("String"=w400:string)  [unwired: 8 in, 1 out]
                      }
                    }
                  }
                  frame "AlazarTech" {
                    w407 = u32 268435537 items=["Data Width"=268435465, "Set/Get Async BuffSize"=268435513, "Set/Get Async Buffcount"=268435520, "Get Data Format"=268435522, "Get Samples Per Timestamp Clock"=268435524, "Get Records Captured"=268435525, "Get Async Buffers Pending"=268435536, "Get Async Buffers Pending Full"=268435537, "Get Async Buffers Pending Empty"=268435538, "ECC Mode"=268435528, "Get Aux Input Level"=268435529, "Get Channels Per Board"=268435568, "Pack Mode"=268435570, "Get FPGA Temperature"=268435584] ("Parameter")
                    w406 = u32 268435536 items=["Data Width"=268435465, "Set/Get Async BuffSize"=268435513, "Set/Get Async Buffcount"=268435520, "Get Data Format"=268435522, "Get Samples Per Timestamp Clock"=268435524, "Get Records Captured"=268435525, "Get Async Buffers Pending"=268435536, "Get Async Buffers Pending Full"=268435537, "Get Async Buffers Pending Empty"=268435538, "ECC Mode"=268435528, "Get Aux Input Level"=268435529, "Get Channels Per Board"=268435568, "Pack Mode"=268435570, "Get FPGA Temperature"=268435584] ("Parameter")
                    w405 = u32 268435520 items=["Data Width"=268435465, "Set/Get Async BuffSize"=268435513, "Set/Get Async Buffcount"=268435520, "Get Data Format"=268435522, "Get Samples Per Timestamp Clock"=268435524, "Get Records Captured"=268435525, "Get Async Buffers Pending"=268435536, "Get Async Buffers Pending Full"=268435537, "Get Async Buffers Pending Empty"=268435538, "ECC Mode"=268435528, "Get Aux Input Level"=268435529, "Get Channels Per Board"=268435568, "Pack Mode"=268435570, "Get FPGA Temperature"=268435584] ("Parameter")
                    w415 = 0.0 ("Offset delay (us)")
                    n194 = Unbundle By Name(w418) -> ("Digitizer ID Cluster.Acqiris/Alazar/SP ID"=w422:u32[])
                    n195 = local read "Samp rate"() -> (w416:dbl)
                    n196 = Bundle By Name(cluster=w418, "Offset delay (us)"=w415, "Additional dig delay (us)"=w415, "Samp Rate (Hz)"=w416) -> (w417:T31)
                    n197 = Index Array(array=w422) -> (element=w421:u32)  [unwired: 1 in]
                    n198 = call "DelayPtsAdjust.vi"("Digitizer Settings"=w417) -> ("PostDelayCorrection"=w414:u32)  [unwired: 9 in, 1 out]
                    n199 = case shown="False" w401 {
                      tunnel: w421 -> [w426 w427]
                      tunnel: [w425 w427] -> w413
                      tunnel: [w424 _] -> w412
                      tunnel: u32 50 ("milliseconds to wait") -> [w423 w428]
                      tunnel: [w423 w428] -> w419
                      frame False {
                        n200 = call "AlazarStartCapture.vi"("Handle"=w426) -> ("Handle"=w425:u64, "error out"=w424:errorcluster)  [unwired: 1 in, 1 out]
                      }
                      frame True {
                      }
                    }
                    n201 = Wait (ms)(milliseconds to wait=w419) -> ()  [unwired: 1 out]
                    n202 = call "AlazarGetParameter.vi"("error in (no error)"=w412, "Parameter"=w405, "Handle"=w413) -> ("error out"=w411:errorcluster, "Value"=w404:i32, "Handle"=w409:u64)  [unwired: 1 in, 1 out]
                    n203 = call "AlazarGetParameter.vi"("error in (no error)"=w411, "Parameter"=w406, "Handle"=w409) -> ("error out"=w410:errorcluster, "Value"=w403:i32, "Handle"=w408:u64)  [unwired: 1 in, 1 out]
                    n204 = call "AlazarGetParameter.vi"("error in (no error)"=w410, "Parameter"=w407, "Handle"=w408) -> ("Value"=w402:i32)  [unwired: 1 in, 3 out]
                  }
                  frame "Teledyne" {
                    n205 = Unbundle By Name(w440) -> ("Digitizer ID Cluster.ADQRef"=w435:refnum<k24>, "Digitizer ID Cluster.adq_cu_ptr"=w431:refnum<k24>, "Digitizer ID Cluster.GaGe Handle.Boards"=w433:u32)
                    n206 = call "SPADQ_DisarmArmTrigger.vi"("adq_num"=w433, "adq_cu_ptr in"=w431, "ADQAPI Ref"=w435) -> ("error out"=w432:errorcluster, "ADQAPI Ref (out)"=w434:refnum<k24>)  [unwired: 7 in]
                    n207 = call "SPADQ_ArmTrigger.vi"("error in (no error)"=w432, "adq_num"=w433, "adq_cu_ptr in"=w431, "ADQAPI Ref"=w434) -> ("error out"=w438:errorcluster, "ADQAPI Ref (out)"=w439:refnum<k24>)  [unwired: 6 in]
                    n208 = call "SPADQ_AcquisitionStatus.vi"("WaitTime (ms)"=1000.0, "error in (no error)"=w438, "adq_num"=w433, "adq_cu_ptr in"=w431, "ADQAPI Ref"=w439) -> ("error out"=w436:errorcluster, "Error Text"=w430:string, "ADQAPI Ref (out)"=w437:refnum<k24>)  [unwired: 3 in, 1 out]
                    n209 = disable-structure shown="Disabled" {
                      disable-tunnel: w437 -> [w444 _]
                      disable-tunnel: w436 -> [w443 _]
                      disable-tunnel: w433 -> [w442 _]
                      disable-tunnel: w431 -> [w441 _]
                      frame Disabled {
                        n210 = call "SPADQ_DisarmArmTrigger.vi"("error in (no error)"=w443, "adq_num"=w442, "adq_cu_ptr in"=w441, "ADQAPI Ref"=w444) -> ()  [unwired: 6 in, 2 out]
                      }
                      frame Enabled {
                      }
                    }
                  }
                }
                "Error Message" <- w313
                n211 = property class="VI"() -> (reference out=w316:refnum<vi>, "Front Panel.IsFrontmost"=w315:bool)  [unwired: 2 in, 1 out]
                n212 = case shown="False" w315 {
                  tunnel: w316 -> [w446 _]
                  frame False {
                    n213 = property class="VI"(reference=w446, "Front Panel.IsFrontmost"=TRUE) -> ()  [unwired: 1 in, 2 out]
                  }
                  frame True {
                  }
                }
              }
              frame #1 {
                # "Can View Spectrum Also"
                # "Read voltage and convery to MV. Make plot\nshowing what will be captured as RF data. Yellow\ncurser can be moved to provide addtional time shift for digitizer\ndealy."
                n214 = local read "Channel tab"() -> (w462:enum32{"C1", "C2", "C3", "C4"})
                n215 = case shown="\"Acqiris Digitizer\"" w463 {
                  tunnel: [w483 w504 w512 w538 w569] -> w458
                  tunnel: w460 -> [w478 w495 w506 w537 w574]
                  tunnel: w462 -> [w481 w500 w516 w534 _]
                  tunnel: w456 -> [w479 w497 w509 w535 w572]
                  tunnel: [_ w496 _ _ _] -> _
                  tunnel: [w482 w502 w507 w539 w579] -> w449
                  tunnel: [w478 w495 w506 w537 w573] -> w451
                  tunnel: w450 -> [_ _ _ w536 _]
                  tunnel: w448 -> [_ _ _ w533 _]
                  tunnel: w447 -> [_ _ _ w532 _]
                  frame "Acqiris Digitizer" {
                    n216 = Unbundle By Name(w479) -> ("Digitizer ID Cluster.Acqiris/Alazar/SP ID"=w480:u32[])
                    n217 = disable-structure shown="Disabled" {
                      disable-tunnel: [w494 _] -> w483
                      disable-tunnel: [w491 _] -> w482
                      disable-tunnel: w481 -> [w488 _]
                      disable-tunnel: w480 -> [w485 _]
                      disable-tunnel: w478 -> [w484 _]
                      frame Disabled {
                        w487 = 1
                        n218 = Index Array(array=w485) -> (element=w493:u32)  [unwired: 1 in]
                        n219 = Add(x=w487, y=w488) -> (x+y=w486:u32)
                        n220 = call "GetWaveform.vi"("Acq ID Out"=w493, "Read Mode"=enum32{"ADC", "Volts"}."Volts", "Num Samps"=w484, "Num Segs"=w487, "Channel"=w486) -> ("Acq ID Out"=→"dup id":u32, "first row"=w494:dbl[], "dataDesc"=w492:T52)  [unwired: 1 in, 7 out]
                        n221 = Unbundle By Name(w492) -> ("sampTime"=w491:dbl)
                      }
                      frame Enabled {
                      }
                    }
                  }
                  frame "NI Digitizer", Default {
                    n222 = Unbundle By Name(w497) -> ("Digitizer ID Cluster.NI Instr Handles"=w498:refnum<k15>[])
                    n223 = Index Array(array=w498) -> (element=w499:refnum<k15>)  [unwired: 1 in]
                    n224 = Number To Decimal String(number=w500) -> (decimal integer string=w501:string)  [unwired: 1 out]
                    n225 = call-poly <instrlib>:"niScope Fetch (poly).vi"("timeout"=2.0, "numSamples"=w495, "channels"=w501, "instrument handle"=w499) -> ("error out"=w496:errorcluster, "wfm"=w504:dbl[], "wfm info"=w503:T53)  [unwired: 1 in, 4 out]
                    n226 = Unbundle By Name(w503) -> ("xIncrement"=w502:dbl)
                  }
                  frame "GaGe" {
                    n227 = Unbundle By Name(w509) -> ("Digitizer ID Cluster.GaGe Handle"=w510:T51)
                    n228 = flat-sequence {
                      tunnel: w516 -> [w521]
                      tunnel: [w523] -> w515
                      tunnel: [w521] -> w514
                      tunnel: w510 -> [w522]
                      tunnel: [w522] -> w508
                      tunnel: [w531] -> w513
                      tunnel: [w530] -> w507
                      tunnel: w515 -> [w530]
                      tunnel: w514 -> [w529]
                      tunnel: [w528] -> w511
                      tunnel: w508 -> [w526]
                      tunnel: w506 -> [w525]
                      frame #0 {
                        n229 = call "CsTool-QueryAcquisitionParametersFill.vi"("Handle Cluster"=w522) -> ("Sample Rate"=w524:dbl)  [unwired: 10 out]
                        n230 = Reciprocal(x=w524) -> (1/x=w523:dbl)
                      }
                      frame #1 {
                        n231 = call "CsTool-TransferFill.vi"("Channel (0)"=w529, "Handle Cluster"=w526) -> ("Actual Length"=w527:dbl, "Data in Volts"=w531:dbl[])  [unwired: 4 in, 2 out]
                        n232 = Greater?(x=w527, y=w525) -> (0:w528:bool)
                      }
                    }
                    n233 = case shown="True" w511 {
                      tunnel: [w517 w520] -> w512
                      tunnel: w513 -> [w517 w519]
                      tunnel: w506 -> [_ w518]
                      frame False {
                      }
                      frame True {
                        n234 = Array Subset(array=w519, length=w518) -> (w520:dbl[])  [unwired: 1 in]
                      }
                    }
                  }
                  frame "AlazarTech" {
                    n235 = stacked-sequence {
                      seq-local: [_ w552 _] -> [_ _ w565]
                      seq-local: [w543 _ _] -> [_ w551 _]
                      seq-local: [w541 _ _] -> [_ w550 _]
                      seq-local: [w540 _ _] -> [_ w549 _]
                      tunnel: [_ w562 _] -> w539
                      tunnel: [_ w561 _] -> w538
                      tunnel: w536 -> [_ w560 _]
                      tunnel: w535 -> [w546 _ _]
                      tunnel: w534 -> [w542 _ _]
                      tunnel: w533 -> [_ w553 _]
                      tunnel: w532 -> [_ w547 _]
                      frame #0 {
                        n236 = call "AlazarCardChannel.vi"("Channel tab"=w542, "Digitizer Settings"=w546) -> ("ChansOnOneCard"=w540:i32, "Channel"=w541:u32, "Card ID"=w545:u32)  [unwired: 7 in]
                        n237 = Build Array(w545) -> (w544:u32[])
                        n238 = Bundle By Name(cluster=w546, "Digitizer ID Cluster.Acqiris/Alazar/SP ID"=w544) -> (w543:T31)
                      }
                      frame #1 {
                        w557 = 1000
                        n239 = call "AlazarStackChannels5Pass.vi"("lines per plane"=w547, "AlazarCluster"=w560, "Digitizer Settings"=w551, "Channels"=w549) -> ("Voltage Scale"=w555:dbl, "Return Code"=w552:u32, "ChStackDataOut"=w559:i16[][][])  [unwired: 4 in, 1 out]
                        n240 = local read "Time scale per Div"() -> (w564:dbl)
                        n241 = Decrement(x=w550) -> (x-1=w548:u32)
                        n242 = Index Array(array=w559, index (dim 0)=w548, index (dim 1)=0) -> (element=w558:i16[])  [unwired: 1 in]
                        n243 = Array Subset(array=w558, index=w553, length=w557) -> (w556:i16[])
                        n244 = expression code="x*1E-5"(w564) -> (w563:dbl)
                        n245 = Multiply(x=w555, y=w556) -> (x*y=w561:dbl[])
                        n246 = Divide(x=w563, y=w557) -> (x/y=w562:dbl)
                      }
                      frame #2 {
                        n247 = local read "Crate Delay"() -> (w566:dbl)
                        n248 = case shown="0, Default" w565 {
                          tunnel: w566 -> [w567 _]
                          frame 0, Default {
                            n249 = property on="Crate Delay" class="DigNum (strict)"("Val(Sgnl)"=w567) -> ()  [unwired: 2 in, 2 out]
                          }
                          frame 512 {
                          }
                        }
                      }
                    }
                  }
                  frame "Teledyne" {
                    n250 = local read "Time scale per Div"() -> (w582:dbl)
                    n251 = Bundle By Name(cluster=w572, "lines per plane"=1, "rf points per line"=w574) -> (w577:T31)
                    n252 = Multiply(x=w582, y=100.0) -> (x*y=w575:dbl)
                    n253 = call "SPADQ_GetData.vi"("Digitizer Settings"=w577) -> ("Data Out"=w578:i16[][])  [unwired: 8 in, 2 out]
                    n254 = Multiply(x=w575, y=1e-10) -> (x*y=w579:dbl)
                    n255 = Index Array(array=w578) -> (element=w580:i16[])  [unwired: 2 in]
                    n256 = call "Alazar_ConvertRaw.vi"("Digitizer Settings"=w572) -> ("Voltage multiplier"=w570:dbl)  [unwired: 9 in, 1 out]
                    n257 = Divide(x=w574, y=w575) -> (x/y=w573:dbl)
                    n258 = call-poly <vilib>:"Decimate (single shot).vi"("decimating factor"=w575, "X"=w580) -> ("Decimated Array"=w571:dbl[])  [unwired: 8 in, 1 out]
                    n259 = Multiply(x=w570, y=w571) -> (x*y=w569:dbl[])
                  }
                }
                n260 = Unbundle By Name(w456) -> ("bits A/D"=w455:i8)
                n261 = property on="Filter Prameters" class="Clust (strict)"("Visible"=w457) -> ()  [unwired: 2 in, 2 out]
                n262 = case shown="True" w457 {
                  tunnel: w458 -> [w468 w477]
                  tunnel: [w468 w470] -> w459
                  tunnel: w449 -> [_ w472]
                  tunnel: w455 -> [_ w469]
                  frame False {
                  }
                  frame True {
                    w473 = u16 4 items=["Mean from lines", "Mean just lines", "Poly Mean", "No mean", "Filter"] ("Type of Mean")
                    n263 = Build Array(w477) -> (w476:dbl[][])
                    n264 = expression code="1/x*1E-6"(w472) -> (w471:dbl)
                    n265 = call "SubMean.vi"("Bit Depth"=w469, "Scan Data In"=w476, "Samp Rate (MHz)"=w471, "Filter Prams"="Filter Prameters", "Type of Mean"=w473) -> ("Array"=w475:dbl[][])  [unwired: 1 in, 2 out]
                    n266 = Index Array(array=w475) -> (element=w470:dbl[])  [unwired: 2 in]
                  }
                }
                n267 = case shown="False" w464 {
                  tunnel: [w586 w593] -> w453
                  tunnel: w459 -> [w587 w598]
                  tunnel: [w584 w592] -> w454
                  tunnel: w452 -> [_ w597]
                  tunnel: w449 -> [_ w596]
                  tunnel: [i32[] [] w594] -> w465
                  tunnel: w451 -> [w583 _]
                  frame False {
                    n268 = Divide(x=10, y=w583) -> (x/y=w584:dbl)
                    n269 = expression code="x*1000"(w587) -> (w586:dbl[])
                  }
                  frame True {
                    n270 = Transpose 2D Array(2D array=w597) -> (transposed array=w599:dbl[][])
                    n271 = for {
                      tunnel: w599 -> [w607] mode=indexing
                      tunnel: [w606] -> w591 mode=indexing
                      n272 = call-poly <vilib>:"Mean.vi"("X"=w607) -> ("mean"=w606:dbl)  [unwired: 1 out]
                    }
                    n273 = case shown="True" "Norm Spect?" {
                      tunnel: [w601 w603] -> w590
                      tunnel: w591 -> [w601 w604]
                      frame False {
                      }
                      frame True {
                        n274 = Absolute Value(x=w604) -> (abs(x)=w605:dbl[])
                        n275 = Array Max & Min(array=w605) -> (max value=w602:dbl)  [unwired: 3 out]
                        n276 = Divide(x=w604, y=w602) -> (x/y=w603:dbl[])
                      }
                    }
                    n277 = call <vilib>:"Auto Power Spectrum.vi"("dt"=w596, "Signal (V)"=w598) -> ("df"=w595:dbl, "Power Spectrum (V^2 rms)"=w594:dbl[])
                    n278 = expression code="log(x)*10"(w590) -> (w593:dbl[])
                    n279 = Multiply(x=w595, y=1e-06) -> (x*y=w592:dbl)
                  }
                }
                n280 = expression code="x*1000"(w458) -> (w461:dbl[])
                n281 = Bundle(0, w454, "Array"=w453) -> (→"Waveform Graph":cluster{i32, dbl, "Array":dbl[]})  [unwired: 1 out]
              }
              frame #2 {
                n282 = case shown="True" w617 {
                  tunnel: w615 -> [_ w638]
                  tunnel: w616 -> [_ w637]
                  tunnel: w614 -> [_ w628]
                  tunnel: w613 -> [_ w636]
                  tunnel: w612 -> [_ w622]
                  tunnel: w611 -> [_ w624]
                  tunnel: w610 -> [_ w620]
                  tunnel: w609 -> [_ w619]
                  tunnel: w608 -> [_ w618]
                  frame False {
                  }
                  frame True {
                    n283 = Unbundle By Name(w622) -> ("bits A/D"=w623:i8)
                    n284 = Unbundle By Name(w622) -> ("Dig Config"=w621:T33)
                    n285 = case shown="\"Acqiris Digitizer\"" w636 {
                      tunnel: [w689 w714 w733 _] -> w635
                      tunnel: w638 -> [w688 w712 _ _]
                      tunnel: w637 -> [w687 _ _ _]
                      tunnel: w628 -> [w686 w716 _ _]
                      tunnel: w622 -> [w681 w713 w735 _]
                      tunnel: w621 -> [w677 _ _ _]
                      tunnel: w620 -> [_ _ w732 _]
                      tunnel: w618 -> [_ _ w734 _]
                      frame "Acqiris Digitizer" {
                        w682 = 1
                        n286 = Not Equal?(x=w682, y=w677) -> (x != y?=w684:bool)
                        n287 = Unbundle By Name(w681) -> ("Digitizer ID Cluster.Acqiris/Alazar/SP ID"=w679:u32[])
                        n288 = Select(t=4, s=w684, f=w682) -> (s? t:f=w685:i32)
                        n289 = Index Array(array=w679, index=1) -> (element=w678:u32)
                        n290 = for {
                          N: w685 -> [_]
                          tunnel: w686 -> [w695]
                          tunnel: [w692] -> w690 mode=indexing
                          tunnel: w687 -> [w694]
                          tunnel: w678 -> [w691]
                          i -> [w696]
                          n291 = disable-structure shown="Disabled" {
                            disable-tunnel: w696 -> [w702 _]
                            disable-tunnel: w695 -> [w700 _]
                            disable-tunnel: [w699 _] -> w693
                            disable-tunnel: w691 -> [w697 _]
                            frame Disabled {
                              n292 = Increment(x=w702) -> (x+1=w703:i32)
                              n293 = call "GetWaveform.vi"("Acq ID Out"=w697, "Read Mode"=enum32{"ADC", "Volts"}."Volts", "Num Samps"=w700, "Num Segs"=1, "Channel"=w703) -> ("first row"=w699:dbl[])  [unwired: 1 in, 9 out]
                            }
                            frame Enabled {
                            }
                          }
                          n294 = case shown="True" w694 {
                            tunnel: w693 -> [w705 w708]
                            tunnel: [w704 w706] -> w692
                            frame False {
                              n295 = expression code="x*1000"(w705) -> (w704:dbl[])
                            }
                            frame True {
                              n296 = call <vilib>:"Auto Power Spectrum.vi"("Signal (V)"=w708) -> ("Power Spectrum (V^2 rms)"=w707:dbl[])  [unwired: 1 in, 1 out]
                              n297 = expression code="log(x)*10"(w707) -> (w706:dbl[])
                            }
                          }
                        }
                        n298 = Build Array (concatenate)(w690, w688) -> (w689:dbl[][])
                      }
                      frame "NI Digitizer" {
                        n299 = Unbundle By Name(w713) -> ("NI ID/Channel"=w711:cluster{"NI ID":refnum<k15>, "NI CH":i32}[])
                        n300 = Array Subset(array=w711, index=1) -> (w709:cluster{"NI ID":refnum<k15>, "NI CH":i32}[])  [unwired: 1 in]
                        n301 = for {
                          tunnel: [w722] -> w715 mode=indexing
                          tunnel: w716 -> [w724]
                          tunnel: [w723] -> _ mode=indexing
                          tunnel: w709 -> [w720] mode=indexing
                          n302 = Unbundle By Name(w720) -> ("NI ID"=w719:refnum<k15>, "NI CH"=w718:i32)
                          n303 = Number To Decimal String(number=w718) -> (decimal integer string=w717:string)  [unwired: 1 out]
                          n304 = call-poly <instrlib>:"niScope Fetch (poly).vi"("timeout"=0.1, "numSamples"=w724, "channels"=w717, "instrument handle"=w719) -> ("error out"=w723:errorcluster, "wfm"=w721:dbl[])  [unwired: 1 in, 5 out]
                          n305 = expression code="x*1000"(w721) -> (w722:dbl[])
                        }
                        n306 = Build Array (concatenate)(w712, w715) -> (w714:dbl[][])
                      }
                      frame "AlazarTech" {
                        w726 = 4
                        # "Annular array 4 channel grab"
                        n307 = call "AlazarStackChannels5Pass.vi"("lines per plane"=1, "AlazarCluster"=w732, "Digitizer Settings"=w735, "Channels"=w726) -> ("Voltage Scale"=w729:dbl, "ChStackDataOut"=w728:i16[][][])  [unwired: 4 in, 2 out]
                        n308 = for {
                          N: w726 -> [_]
                          tunnel: w734 -> [w739]
                          tunnel: [w737] -> w730 mode=indexing
                          tunnel: w728 -> [w736]
                          i -> [w742]
                          n309 = Index Array(array=w736, index (dim 0)=w742, index (dim 1)=0 ("disabled index (row)")) -> (element=w740:i16[])  [unwired: 1 in]
                          n310 = Array Subset(array=w740, index=w739, length=1000) -> (w737:i16[])
                        }
                        n311 = Multiply(x=w730, y=w729) -> (x*y=w731:dbl[][])
                        n312 = expression code="x*1000"(w731) -> (w733:dbl[][])
                      }
                      frame "No Digitizer", Default {
                      }
                    }
                    n313 = Decrement(x="Display Channel") -> (x-1=w633:i32)
                    n314 = case shown="-1" w633 {
                      selector: w633 -> [_ w676]
                      tunnel: [w672 w673] -> w625
                      tunnel: w635 -> [w672 w675]
                      frame -1 {
                      }
                      frame 0, Default {
                        n315 = Array Subset(array=w675, index (row)=w676, length (row)=1 ("length")) -> (w673:dbl[][])  [unwired: 2 in]
                      }
                    }
                    n316 = for {
                      tunnel: [w642] -> w626 mode=indexing
                      tunnel: w625 -> [w643] mode=indexing
                      tunnel: w624 -> [w641]
                      tunnel: w623 -> [w640]
                      tunnel: w619 -> [w639]
                      n317 = case shown="True" w641 {
                        tunnel: w643 -> [w644 w653]
                        tunnel: [w644 w647] -> w642
                        tunnel: w639 -> [_ w649]
                        tunnel: w640 -> [_ w645]
                        frame False {
                        }
                        frame True {
                          w650 = u16 4 items=["Mean from lines", "Mean just lines", "Poly Mean", "No mean", "Filter"] ("Type of Mean")
                          n318 = property on="Filter Prameters" class="Clust (strict)"() -> ("Value"=w646:T26)  [unwired: 2 in, 2 out]
                          n319 = Build Array(w653) -> (w652:dbl[][])
                          n320 = expression code="1/x*1E-6"(w649) -> (w648:dbl)
                          n321 = call "SubMean.vi"("Bit Depth"=w645, "Scan Data In"=w652, "Samp Rate (MHz)"=w648, "Filter Prams"=w646, "Type of Mean"=w650) -> ("Array"=w651:dbl[][])  [unwired: 1 in, 2 out]
                          n322 = Index Array(array=w651) -> (element=w647:dbl[])  [unwired: 2 in]
                        }
                      }
                    }
                    n323 = case shown="False" "Crate Spectra" {
                      tunnel: w626 -> [w657 w660]
                      tunnel: [w654 w662] -> w627
                      tunnel: [w657 w661] -> w629
                      tunnel: w628 -> [w655 _]
                      frame False {
                        n324 = Divide(x=10, y=w655) -> (x/y=w654:dbl)
                      }
                      frame True {
                        n325 = Array Size(array=w660) -> (size(s)=w659:i32[])
                        n326 = Index Array(array=w659) -> (element=w658:i32)  [unwired: 1 in]
                        n327 = for {
                          N: w658 -> [_]
                          tunnel: [w666] -> w661 mode=indexing
                          tunnel: [w669] -> w662
                          tunnel: w660 -> [w668]
                          i -> [w667]
                          n328 = Index Array(array=w668, index (row)=w667) -> (element=w664:dbl[])  [unwired: 1 in]
                          n329 = expression code="x/1000"(w664) -> (w665:dbl[])
                          n330 = call <vilib>:"Auto Power Spectrum.vi"("Signal (V)"=w665) -> ("df"=w670:dbl, "Power Spectrum (V^2 rms)"=w663:dbl[])  [unwired: 1 in]
                          n331 = expression code="log(x)*10"(w663) -> (w666:dbl[])
                          n332 = Multiply(x=w670, y=1e-06) -> (x*y=w669:dbl)
                        }
                      }
                    }
                    n333 = Bundle(0, w627, "Power Spectrum (V^2 rms)"=w629) -> (→"Crate Waveforms":T54)  [unwired: 1 out]
                  }
                }
              }
              frame #3 {
                n334 = case shown="True" w743 {
                  tunnel: w744 -> [w745 _]
                  frame False {
                    n335 = Unbundle By Name(w745) -> ("Digitizer ID Cluster.Acqiris/Alazar/SP ID"=w746:u32[])
                    n336 = Index Array(array=w746) -> (element=w747:u32)  [unwired: 1 in]
                    n337 = call "AlazarAbortAsyncRead.vi"("Handle"=w747) -> ()  [unwired: 1 in, 3 out]
                  }
                  frame True {
                    n338 = case shown="True" FALSE {
                      frame False {
                      }
                      frame True {
                        # "Hack to better deal with no trigger source"
                        n339 = property on="Crate Delay" class="DigNum (strict)"() -> (error out=w749:errorcluster, "Value"=w750:dbl)  [unwired: 2 in, 1 out]
                        n340 = property on="Crate Delay" class="DigNum (strict)"(error in=w749, "Val(Sgnl)"=w750) -> ()  [unwired: 1 in, 2 out]
                      }
                    }
                  }
                }
              }
            }
          }
          event "Waveform Graph": Cursor Move; "Crate Delay", "RF data Sampling", "Delay Corr?": Value Change; "Waveform Graph": Cursor Release {
            n341 = event-data() -> ("Type"=w755:T55)  [unwired: 1 out]
            n342 = stacked-sequence {
              seq-local: [w773 _ _] -> [_ w811 _]
              seq-local: [w771 _ _] -> [_ w785 _]
              seq-local: [w770 _ _] -> [_ w797 _]
              seq-local: [_ w794 _] -> [_ _ w977]
              seq-local: [_ w784 _] -> [_ _ w971]
              tunnel: w765 -> [_ _ _]
              tunnel: "RF data Sampling" -> [w772 w795 _]
              tunnel: w764 -> [_ _ _]
              tunnel: w763 -> [w766 w793 _]
              tunnel: w762 -> [_ _ w978]
              tunnel: w760 -> [_ _ w974]
              tunnel: [_ w794 _] -> w759
              tunnel: [_ _ w974] -> w758
              tunnel: w757 -> [_ _ w976]
              tunnel: [_ _ w975] -> w756
              tunnel: w755 -> [_ _ _]
              tunnel: w754 -> [_ w790 _]
              tunnel: w752 -> [_ w781 _]
              tunnel: w751 -> [_ w780 _]
              frame #0 {
                # "Set up delays"
                # "in microseconds"
                # "in microseconds"
                n343 = Unbundle By Name(w772) -> ("Ref Delay (ms)"=w771:dbl, "rf points per line"=w769:i32)
                n344 = Unbundle By Name(w766) -> ("Offset delay (us)"=w767:dbl)
                n345 = Bundle By Name(cluster=w766, "Digitizer delay (us)"=w771, "rf points per line"=w769, "Rel Dig Delay"="Crate Delay") -> (w770:T31)
                n346 = Add(x=w767, y=w771) -> (x+y=w779:dbl)
                n347 = Add(x=w779, y="Crate Delay") -> (x+y=w778:dbl)
                n348 = Build Array(w779, w778) -> (w777:dbl[])
                n349 = expression code="x*1E-6"(w777) -> (w776:dbl[])
                n350 = In Range and Coerce(upper limit=1, x=w776, lower limit=0) -> (coerced(x)=w773:dbl[])  [unwired: 1 out]
                "RF data Sampling Out" <- w772
              }
              frame #1 {
                w817 = u32 1 ("Write Attribute")
                # "TGC Settings"
                # "Handle neg delay case"
                # "Take care of data window display"
                n351 = Unbundle By Name(w795) -> ("Ref Delay (ms)"=w789:dbl, "rf points per line"=w807:i32, "Sampling Rate"=w800:dbl)
                n352 = property on="Waveform Graph" class="WFGraph (strict)"("Active Cursor"=w817) -> ("Cursor.Cursor Position:Cursor X"=w819:dbl)  [unwired: 2 in, 2 out]
                n353 = Unbundle By Name(w793) -> ("Main Digitizer"=w792:T32)
                n354 = expression code="x*10"("Time scale per Div") -> (w806:dbl)
                n355 = expression code="x*1E-5"("Time scale per Div") -> (w809:dbl)
                n356 = Less Than 0?(x=w819) -> (x < 0?=w818:bool)
                n357 = case shown="True" w818 {
                  tunnel: w819 -> [w967 _]
                  tunnel: [w967 w968] -> w815
                  tunnel: w817 -> [_ w970]
                  frame False {
                  }
                  frame True {
                    w968 = 0
                    n358 = property on="Waveform Graph" class="WFGraph (strict)"("X Scale.Range:Minimum"=w968, "X Scale.Range:Maximum"=10, "Active Cursor"=w970, "Cursor.Cursor Position:Cursor X"=w968) -> ()  [unwired: 2 in, 2 out]
                  }
                }
                n359 = Divide(x=w789, y=w806) -> (x/y=w805:dbl)
                n360 = expression code="x*100"(w805) -> (w804:dbl)
                n361 = In Range and Coerce(upper limit=100.0, x=w804, lower limit=0.0) -> (coerced(x)=w801:dbl)  [unwired: 1 out]
                n362 = case shown="\"Acqiris Digitizer\", Default" w792 {
                  tunnel: w811 -> [w828 w860 w884 w906 w964]
                  tunnel: "Display Crate?" -> [w827 w854 _ _ _]
                  tunnel: [w826 w858 w894 w907 w944] -> w814
                  tunnel: [w825 w855 w881 w905 w946] -> w808
                  tunnel: w809 -> [w824 w859 w895 w908 w966]
                  tunnel: w801 -> [_ w856 _ _ _]
                  tunnel: w793 -> [w823 w850 w880 w904 w949]
                  tunnel: "Time scale per Div" -> [_ _ _ _ w963]
                  tunnel: w781 -> [_ _ _ w903 _]
                  tunnel: w780 -> [_ _ _ w902 _]
                  frame "Acqiris Digitizer", Default {
                    n363 = Unbundle By Name(w823) -> ("Digitizer ID Cluster.Acqiris/Alazar/SP ID"=w822:u32[])
                    n364 = disable-structure shown="Disabled" {
                      disable-tunnel: w828 -> [w837 _]
                      disable-tunnel: w827 -> [w833 _]
                      disable-tunnel: [w832 _] -> w826
                      disable-tunnel: [w831 _] -> w825
                      disable-tunnel: w824 -> [w830 _]
                      disable-tunnel: w822 -> [w829 _]
                      frame Disabled {
                        n365 = Select(t=2, s=w833, f=1) -> (s? t:f=w834:i32)
                        n366 = for {
                          N: w834 -> [_]
                          tunnel: w830 -> [w845]
                          tunnel: w837 -> [w847] mode=indexing
                          tunnel: [w846] -> w832
                          tunnel: [w840] -> w831
                          tunnel: w829 -> [w844] mode=indexing
                          n367 = call <instrlib>:"Query Best Sampling Interval.vi"("Time Window (1E-6 s)"=w845, "Maximum Samples (10000)"=2000, "Instrument ID"=w844) -> ("error out"=w838:errorcluster, "Sampling Interval (s)"=w846:dbl, "Nominal Samples"=w840:i32, "dup Instrument ID"=w839:u32)  [unwired: 1 in]
                          n368 = call <instrlib>:"Configure Horizontal Settings.vi"("error in (no error)"=w838, "Delay Time (0 s)"=w847, "Sampling Interval (10 ns)"=w846, "Instrument ID"=w839) -> ("error out"=w842:errorcluster, "dup Instrument ID"=w843:u32)  [unwired: 2 out]
                          n369 = call <instrlib>:"Configure Memory Settings.vi"("error in (no error)"=w842, "Number of Samples (1000)"=w840, "Number of Segments (1)"=1, "Instrument ID"=w843) -> ()  [unwired: 4 out]
                        }
                      }
                      frame Enabled {
                      }
                    }
                  }
                  frame "NI Digitizer" {
                    w855 = 1000
                    n370 = Unbundle By Name(w850) -> ("Digitizer ID Cluster.NI Instr Handles"=w849:refnum<k15>[])
                    n371 = Divide(x=w859, y=w855) -> (x/y=w858:dbl)
                    n372 = Array Size(array=w849) -> (size(s)=w853:i32)
                    n373 = Reciprocal(x=w858) -> (1/x=w857:dbl)
                    n374 = Select(t=w853, s=w854, f=1) -> (s? t:f=w851:i32)
                    n375 = for {
                      N: w851 -> [_]
                      tunnel: w860 -> [w869]
                      tunnel: w857 -> [w874]
                      tunnel: w856 -> [_]
                      tunnel: w855 -> [w861]
                      tunnel: w849 -> [w870] mode=indexing
                      tunnel: [w863] -> _
                      i -> [w867]
                      n376 = In Range and Coerce(upper limit=1, x=w867, lower limit=0) -> (coerced(x)=w864:i32)  [unwired: 1 out]
                      n377 = call <instrlib>:"niScope Configure Horizontal Timing.vi"("instrument handle"=w870, "min sample rate"=w874, "reference position"=0.0 ("lower limit"), "min record length"=w861) -> ("instrument handle out"=w875:refnum<k15>, "error out"=w873:errorcluster)  [unwired: 3 in, 7 out]
                      n378 = Index Array(array=w869, index=w864) -> (element=w868:dbl)
                      n379 = property class="niScope"(reference=w875, error in=w873, "Trigger Delay"=w868, "Fetch Record Number"=0, "Fetch Number of Records"=-1 ("Fetch:Fetch Number of Records")) -> (error out=w863:errorcluster)  [unwired: 1 out]
                    }
                  }
                  frame "GaGe" {
                    w888 = u16 0 items=["Single", "Dual", "Quad", "Octal"] ("Mode")
                    w881 = 1000
                    # "Pt total\nw/ delay"
                    # "Delay in pts"
                    n380 = Unbundle By Name(w880) -> ("Digitizer ID Cluster.GaGe Handle"=w879:T51)
                    n381 = Divide(x=w895, y=w881) -> (x/y=w894:dbl)
                    n382 = Reciprocal(x=w894) -> (1/x=w890:dbl)
                    n383 = Index Array(array=w884) -> (element=w891:dbl)  [unwired: 1 in]
                    n384 = Multiply(x=w890, y=w891) -> (x*y=w882:dbl)
                    "Gage Delay Pts" <- w882
                    n385 = Index Array(array=string[] ["Single", "Dual", "Quad", "Octal"], index=w888) -> (element=w887:string)
                    n386 = Add(x=w882, y=w881) -> (x+y=w883:dbl)
                    n387 = Bundle(cluster=T43 {0.0, "Clock mode"=enum."Internal", "RingText.Text"="", 1024, 1024, "time out (ms)"=0.0, 0.0, 0.0} ("output cluster"), w890, "RingText.Text"=w887, w883, w883) -> (w893:T43)  [unwired: 4 in]
                    n388 = call "CsTool-ErrorHandlerAll.vi"("StopOnError (true)"=FALSE, "Error Code"=w886, "Handle Cluster"=w876) -> ()  [unwired: 1 out]
                    n389 = flat-sequence {
                      tunnel: w893 -> [w897]
                      tunnel: w879 -> [w896]
                      tunnel: [w896] -> w878
                      tunnel: [w896] -> w877
                      tunnel: [w900] -> w886
                      tunnel: w878 -> [w899]
                      tunnel: [w898] -> w876
                      tunnel: w877 -> [w898]
                      frame #0 {
                        n390 = call "CsTool-ConfigureAcquisitionAll.vi"("Handle Cluster"=w896, "Acquisition"=w897) -> ()  [unwired: 3 in, 1 out]
                      }
                      frame #1 {
                        w901 = TRUE
                        n391 = call "CsTool-CommitAll.vi"("OnlyOnChange (t)"=w901, "Coerce Flag (f)"=w901, "Handle Cluster"=w899) -> ("Error Code"=w900:i32)  [unwired: 1 out]
                      }
                    }
                    n392 = call "CsTool-QueryAcquisitionParametersFill.vi"("Handle Cluster"=w876) -> ()  [unwired: 11 out]
                  }
                  frame "AlazarTech" {
                    n393 = stacked-sequence {
                      seq-local: [w910 _] -> [_ w927]
                      tunnel: w908 -> [w918 _]
                      tunnel: [w909 _] -> w907
                      tunnel: w906 -> [w917 _]
                      tunnel: [w916 _] -> w905
                      tunnel: w904 -> [w911 _]
                      tunnel: w903 -> [_ w920]
                      tunnel: w902 -> [_ w919]
                      frame #0 {
                        w912 = 0.0 ("Additional dig delay (us)")
                        w916 = 1000
                        n394 = Divide(x=w918, y=w916) -> (x/y=w909:dbl)
                        n395 = Index Array(array=w917) -> (element=w914:dbl)  [unwired: 1 in]
                        n396 = Reciprocal(x=w909) -> (1/x=w915:dbl)
                        "Samp rate" <- w915
                        n397 = expression code="x*1E6"(w914) -> (w913:dbl)
                        n398 = Bundle By Name(cluster=w911, "Digitizer delay (us)"=w913, "rf points per line"=w916, "Samp Rate (Hz)"=w915, "Additional dig delay (us)"=w912, "Offset delay (us)"=w912) -> (w910:T31)
                      }
                      frame #1 {
                        n399 = Unbundle By Name(w927) -> ("rf points per line"=w924:i32, "Digitizer ID Cluster.Acqiris/Alazar/SP ID"=w923:u32[], "Digitizer ID Cluster.GaGe Handle.Boards"=w921:u32)
                        n400 = case shown="2, Default" w921 {
                          tunnel: [w937 w938] -> w925
                          frame 2, Default {
                            w937 = u32 3 items=["A"=1, "B"=2, "A + B"=3, "C"=4, "A + C"=5, "A + B"=6, "D"=8, "A + D"=9, "B + D"=10, "C + D"=12, "A + B + C + D"=15] ("Channel")
                          }
                          frame 16 {
                            w938 = u32 15 items=["A"=1, "B"=2, "A + B"=3, "C"=4, "A + C"=5, "A + B"=6, "D"=8, "A + D"=9, "B + D"=10, "C + D"=12, "A + B + C + D"=15] ("Channel")
                          }
                        }
                        n401 = Index Array(array=w923) -> (element=w922:u32)  [unwired: 1 in]
                        n402 = for {
                          tunnel: [w936] -> w928
                          tunnel: w923 -> [w935] mode=indexing
                          tunnel: w927 -> [w933]
                          tunnel: [w932] -> w926
                          tunnel: w925 -> [w931]
                          tunnel: w924 -> [w930]
                          tunnel: w919 -> [w929]
                          n403 = call "AlazarAcqPrep - ATS-SDK.vi"("Handle"=w935, "Digitizer Settings"=w933, "Channel"=w931, "BuffCount"=4, "rf points per line"=w930, "rf lines per buffer"=w929) -> ("AlazarCluster"=w932:T1, "error out"=w936:errorcluster)  [unwired: 6 in, 2 out]
                        }
                        "AlazarCluster" <- w926
                        n404 = case shown="True" w920 {
                          tunnel: w922 -> [w939 w943]
                          tunnel: [w939 w941] -> _
                          tunnel: [_ w940] -> _
                          tunnel: w928 -> [_ w942]
                          frame False {
                          }
                          frame True {
                            n405 = call "AlazarStartCapture.vi"("Handle"=w943, "error in (no error)"=w942) -> ("Handle"=w941:u64, "error out"=w940:errorcluster)  [unwired: 1 out]
                          }
                        }
                      }
                    }
                  }
                  frame "Teledyne" {
                    (unwired) 1e-10  # samp rate (10 GS/s)
                    # "extra shift needed to hit delay"
                    # "Delay in pts"
                    n406 = Multiply(x=w963, y=100.0) -> (x*y=w961:dbl)
                    n407 = Unbundle By Name(w949) -> ("Digitizer ID Cluster.ADQRef"=w956:refnum<k24>, "Digitizer ID Cluster.adq_cu_ptr"=w958:refnum<k24>, "Digitizer ID Cluster.GaGe Handle.Boards"=w957:u32)
                    n408 = Multiply(x=w961, y=1000) -> (x*y=w946:dbl)
                    n409 = Divide(x=w966, y=w946) -> ()  [unwired: 1 out]
                    n410 = Index Array(array=w964) -> (element=w965:dbl)  [unwired: 1 in]
                    n411 = call "SPADQ_ConfigSampRate.vi"("adq_num"=w957, "adq_cu_ptr in"=w958, "ADQAPI Ref"=w956) -> ("error out"=w952:errorcluster, "SampleRateHz"=w945:dbl, "ADQAPI Ref (out)"=w955:refnum<k24>)  [unwired: 5 in, 1 out]
                    n412 = Reciprocal(x=w945) -> (1/x=w944:dbl)
                    n413 = Multiply(x=w945, y=w965) -> (x*y=w951:dbl)
                    n414 = call "DelayPtsAdjust.vi"("CalcPt?"=FALSE, "Digitizer Settings"=w949, "Delay in Pts"=w951) -> ("Actual Delay pts"=w950:u32, "PostDelayCorrection"=w947:u32)  [unwired: 7 in]
                    n415 = call "SPADQ_TrigDelay.vi"("Delay in Pts"=w950, "error in (no error)"=w952, "adq_num"=w957, "adq_cu_ptr in"=w958, "ADQAPI Ref"=w955) -> ("error out"=w953:errorcluster, "ADQAPI Ref (out)"=w954:refnum<k24>)  [unwired: 4 in, 1 out]
                    n416 = Add(x=w947, y=w946) -> ()  [unwired: 1 out]
                    n417 = call "SPADQ_MultiRecord.vi"("Records"=u32 1 ("nofRecords"), "Pts to Acquire"=w946, "error in (no error)"=w953, "adq_num"=w957, "adq_cu_ptr in"=w958, "ADQAPI Ref"=w954) -> ()  [unwired: 3 in, 3 out]
                  }
                }
                "Nominal Samples" <- w808
                n418 = expression code="x*1E6"(w800) -> (w799:dbl)
                n419 = Multiply(x="Time scale per Div", y=w815) -> (x*y=w796:dbl)
                n420 = call "RFWindow.vi"("rf points per line"=w807, "Sample Time"=w814, "Sampling (Hz) In"=w799) -> ("curser position"=w812:dbl, "Sampling (Hz)"=w798:dbl)  [unwired: 1 in, 2 out]
                n421 = Add(x=w796, y=w785) -> (x+y=w783:dbl)
                "Total Delay (ms)" <- w783
                n422 = Divide(x=10, y=w808) -> (x/y=w813:dbl)
                n423 = Multiply(x=w812, y=w813) -> (x*y=w816:dbl)
                n424 = Bundle By Name(cluster=w797, "Samp Rate (Hz)"=w798, "Additional dig delay (us)"=w796) -> (w794:T31)
                n425 = Multiply(x=w783, y=w790) -> (x*y=w791:dbl)
                n426 = Add(x=w816, y=w815) -> (x+y=w788:dbl)
                n427 = property on="Equivalent RT delay\ndistance (mm)" class="DigNum (strict)"("Value"=w791) -> ()  [unwired: 2 in, 2 out]
                n428 = Multiply(x=w788, y="Time scale per Div") -> (x*y=w786:dbl)
                n429 = property on="Waveform Graph" class="WFGraph (strict)"("Active Cursor"=u32 0, "Cursor.Cursor Position:Cursor X"=w788) -> ()  [unwired: 2 in, 2 out]
                n430 = Add(x=w786, y=w785) -> (x+y=w782:dbl)
                n431 = Bundle(w783, w782) -> (w784:cluster{dbl, dbl})  [unwired: 1 in]
                "t per div" <- "Time scale per Div"
              }
              frame #2 {
                n432 = global read "PulserGlobals.vi" "Daxsonics Name"() -> (w972:T56)
                n433 = local read "Settings Changes"() -> (w973:bool)
                n434 = case shown="True" w973 {
                  tunnel: w974 -> [_ w987]
                  tunnel: w978 -> [_ w986]
                  tunnel: w977 -> [_ w985]
                  tunnel: w976 -> [w982 w984]
                  tunnel: [w982 w983] -> w975
                  frame False {
                  }
                  frame True {
                    n435 = local read "T/R Channel"() -> (w988:u32)
                    n436 = call "UpdateDualXDCRSettings.vi"("Digitizer Settings in"=w985, "Motion Settings in"=w987, "Switch T/R"=w988, "Dual XDCR Settings In"=w984, "Switch Unit"=w986) -> ("Dual XDCR Settings"=w983:T3)  [unwired: 3 in]
                  }
                }
                n437 = case shown="\"New2021\"" w972 {
                  selector: w972 -> [_ w979]
                  tunnel: w971 -> [_ w981]
                  frame "BP1", Default {
                  }
                  frame "New2021" {
                    n438 = global read "PulserGlobals.vi" "Daxsonics VISA"() -> (w980:refnum<visa-resource-name>)
                    n439 = call "DAXSetTGC.vi"("Daxsonics Name"=w979, "TGC Times"=w981, "VISA resource name"=w980) -> ()  [unwired: 8 in, 1 out]
                  }
                }
              }
            }
          }
          event "Equivalent RT delay\ndistance (mm)": Value Change {
            n440 = event-data() -> ("NewVal"=w995:dbl, "OldVal"=w994:dbl)  [unwired: 1 out]
            n441 = Subtract(x=w995, y=w994) -> (x-y=w993:dbl)
            n442 = property on="Ref Delay (ms)" class="DigNum (strict)"() -> ("Value"=w990:dbl)  [unwired: 2 in, 2 out]
            n443 = Divide(x=w993, y=w992) -> (x/y=w991:dbl)
            n444 = Add(x=w990, y=w991) -> (x+y=w989:dbl)
            n445 = property on="Ref Delay (ms)" class="DigNum (strict)"("Val(Sgnl)"=w989) -> ()  [unwired: 2 in, 2 out]
          }
          event "Time scale per Div": Value Change {
            n446 = event-data() -> ()  [unwired: 7 out]
            n447 = Unbundle By Name(w1008) -> ("Additional dig delay (us)"=w1007:dbl)
            n448 = property on="Time scale per Div" class="Ring (strict)"() -> ("Value"=w1010:dbl)  [unwired: 2 in, 2 out]
            n449 = Divide(x=w1007, y=w1010) -> (x/y=w1009:dbl)
            n450 = In Range and Coerce(upper limit=9.9, x=w1009, lower limit=0.0) -> (coerced(x)=w1004:dbl)  [unwired: 1 out]
            n451 = property on="Waveform Graph" class="WFGraph (strict)"("Active Cursor"=u32 1, "Cursor.Cursor X"=w1004) -> ()  [unwired: 2 in, 2 out]
            n452 = property on="RF data Sampling" class="Clust (strict)"() -> (error out=w1006:errorcluster, "Value"=w1005:T36)  [unwired: 2 in, 1 out]
            n453 = property on="RF data Sampling" class="Clust (strict)"(error in=w1006, "Val(Sgnl)"=w1005) -> ()  [unwired: 1 in, 2 out]
          }
          event Key Down {
            n454 = event-data() -> ("VKey"=w1032:T57, "Char"=w1029:i16, "PlatMods"=w1030:T58)  [unwired: 1 out]
            n455 = property on="Position (mm) (Abs)" class="DigNum (strict)"() -> ("Key Focus"=w1018:bool)  [unwired: 2 in, 2 out]
            n456 = property on="Inc. Step Size (mm)" class="DigNum (strict)"() -> ("Key Focus"=w1023:bool)  [unwired: 2 in, 2 out]
            n457 = property on="Level (mV)" class="DigNum (strict)"() -> ("Key Focus"=w1022:bool)  [unwired: 2 in, 2 out]
            n458 = property on="rf points per line" class="DigNum (strict)"() -> ("Key Focus"=w1021:bool)  [unwired: 2 in, 2 out]
            n459 = property on="Ref Delay (ms)" class="DigNum (strict)"() -> ("Key Focus"=w1020:bool)  [unwired: 2 in, 2 out]
            n460 = Unbundle By Name(w1017) -> ("No Motion?"=w1016:bool)
            n461 = control-ref of="Axis Tune"() -> (w1027:refnum<vi>)
            n462 = control-ref of="Position (mm) (Abs)"() -> (w1026:refnum<vi>)
            n463 = Compound Arithmetic op=OR(w1016, w1023, w1022, w1021, w1020, w1018) -> (w1019:bool)
            n464 = control-ref of="Waveform Graph"() -> (w1028:refnum<vi>)
            n465 = call "KeyboardNudge.vi"("WaveformGraph Refnum"=w1028, "Axis Tune Refnum"=w1027, "Char"=w1029, "Position (mm) Refnum"=w1026, "Ignore Key Down"=w1019, "VKey"=w1032, "PlatMods"=w1030, "Inc. Step Size (mm)"="Inc. Step Size (mm)", "Motion Settings"=w1017) -> ("Quit"=w1025:bool)  [unwired: 9 in, 1 out]
          }
          event "Settings Changes": Value Change {
            n466 = event-data() -> ()  [unwired: 7 out]
            n467 = local read "T/R Channel"() -> (w1040:u32)
            n468 = call "UpdateDualXDCRSettings.vi"("Digitizer Settings in"=w1042, "Motion Settings in"=w1041, "Switch T/R"=w1040, "Dual XDCR Settings In"=w1038, "Switch Unit"=w1039) -> ("Dual XDCR Settings"=w1037:T3)  [unwired: 3 in]
          }
          event "Volt Scale 1", "Coupling C1", "Trigger Settings", "Channel tab", "Volt Scale 2", "Coupling C2", "Volt Scale 3", "Coupling C3", "Coupling C4", "Volt Scale 4", "Offset (mV)": Value Change {
            # "Slave all voltage scales to center element."
            # "set up vertical (voltage scale)"
            n469 = event-data() -> ()  [unwired: 2 out]
            n470 = case shown="\"C1\", Default" "Channel tab" {
              tunnel: ["Coupling C1" "Coupling C2" "Coupling C3" "Coupling C4"] -> w1059
              tunnel: ["Volt Scale 1" "Volt Scale 2" "Volt Scale 3" "Volt Scale 4"] -> w1053
              tunnel: w1046 -> [w1070 w1073 w1076 w1079]
              tunnel: [w1069 w1073 w1076 w1079] -> w1057
              frame "C1", Default {
                n471 = Bundle By Name(cluster=w1070, "Voltage Scale"="Volt Scale 1") -> (w1069:T31)
              }
              frame "C2" {
              }
              frame "C3" {
              }
              frame "C4" {
              }
            }
            n472 = Unbundle By Name(w1046) -> ("Main Digitizer"=w1052:T32)
            n473 = case shown="True" w1060 {
              tunnel: w1053 -> [_ w1086]
              tunnel: w1046 -> [_ w1085]
              frame False {
              }
              frame True {
                n474 = Unbundle By Name(w1085) -> ("Total Dig CH"=w1084:i32)
                n475 = Decrement(x=w1084) -> (x-1=w1083:i32)
                n476 = Initialize Array(w1086, w1083) -> (w1082:dbl[])
                n477 = property on="Crate Voltage Scales" class="Arr (strict)"("Val(Sgnl)"=w1082) -> ()  [unwired: 2 in, 2 out]
              }
            }
            n478 = expression code="x/1000"("Offset (mV)") -> (w1054:dbl)
            n479 = Bundle("Volt Scale 4"=w1053, "Offset (mV)"=w1054, "Coupling C4"=w1059) -> (w1061:T59)  [unwired: 1 out]
            "Vert Settings" <- w1061
            n480 = case shown="\"Acqiris Digitizer\"" w1052 {
              tunnel: w1061 -> [w1093 w1110 w1118 w1130 w1139]
              tunnel: "Trigger Settings" -> [w1094 w1109 w1115 w1128 w1141]
              tunnel: "Channel tab" -> [w1092 w1108 _ w1129 w1137]
              tunnel: [_ w1107 w1119 _ _] -> _
              tunnel: w1057 -> [w1089 w1106 w1120 w1124 w1138]
              tunnel: w1053 -> [w1087 _ _ _ w1140]
              frame "Acqiris Digitizer" {
                n481 = Unbundle By Name(w1089) -> ("Digitizer ID Cluster.Acqiris/Alazar/SP ID"=w1088:u32[])
                n482 = Add(x=1, y=w1092) -> (x+y=w1090:u32)
                n483 = disable-structure shown="Disabled" {
                  disable-tunnel: w1094 -> [w1100 _]
                  disable-tunnel: w1093 -> [w1099 _]
                  disable-tunnel: w1090 -> [w1098 _]
                  disable-tunnel: w1088 -> [w1097 _]
                  disable-tunnel: w1087 -> [w1096 _]
                  frame Disabled {
                    n484 = Index Array(array=w1097) -> (element=w1095:u32)  [unwired: 1 in]
                    n485 = call "conVert.vi"("InstrumentID"=w1095, "V scale"=w1099, "Channel (1)"=w1098) -> ("Status"=w1101:i32, "error out"=w1102:errorcluster)  [unwired: 2 in, 1 out]
                    n486 = call "conTrig.vi"("error in"=w1102, "Voltage Scale"=w1096, "Trigger"=w1100, "InstrumentID"=w1101) -> ()  [unwired: 1 in, 2 out]
                  }
                  frame Enabled {
                  }
                }
              }
              frame "NI Digitizer", Default {
                n487 = Unbundle By Name(w1106) -> ("NI ID/Channel"=w1105:cluster{"NI ID":refnum<k15>, "NI CH":i32}[])
                n488 = Index Array(array=w1105) -> (element=w1104:cluster{"NI ID":refnum<k15>, "NI CH":i32})  [unwired: 1 in]
                n489 = Unbundle By Name(w1104) -> ("NI ID"=w1103:refnum<k15>)
                n490 = call "NIconVert.vi"("InstrumentID"=w1103, "V scale"=w1110, "Channel (0)"=w1108) -> ("Status"=w1111:refnum<k15>, "error out"=w1112:errorcluster)  [unwired: 1 in, 2 out]
                n491 = call "NIconTrig.vi"("error in"=w1112, "Trigger"=w1109, "InstrumentID"=w1111) -> ("error out"=w1107:errorcluster)  [unwired: 2 out]
              }
              frame "Teledyne" {
                (unwired) u32 1 ("channel")
                n492 = Unbundle By Name(w1120) -> ("Digitizer ID Cluster.ADQRef"=w1113:refnum<k24>, "Digitizer ID Cluster.adq_cu_ptr"=w1116:refnum<k24>, "Digitizer ID Cluster.GaGe Handle.Boards"=w1114:u32)
                n493 = Unbundle By Name(w1118) -> ("Coupling C4"=w1117:u16)
                n494 = case shown="2, Default" w1117 {
                  tunnel: [1 0] -> _
                  frame 0 {
                  }
                  frame 2, Default {
                  }
                }
                n495 = call "SPconTrig.vi"("Trigger"=w1115, "adq_num"=w1114, "adq_cu_ptr"=w1116, "ADQAPI Ref"=w1113) -> ("error out"=w1119:errorcluster)  [unwired: 5 in, 2 out]
              }
              frame "GaGe" {
                w1126 = TRUE
                n496 = Unbundle By Name(w1124) -> ("Digitizer ID Cluster.GaGe Handle"=w1123:T51)
                n497 = call "GaGe_ChannelConfigAll.vi"("Channel (0)"=w1129, "V scale"=w1130, "Handle Cluster"=w1123) -> ("Handle Cluster Out"=w1127:T51)  [unwired: 2 in]
                n498 = call "GaGe_TrigConfigAll.vi"("Trigger"=w1128, "Handle Cluster"=w1127) -> ("Handle Cluster Out"=w1125:T51)  [unwired: 3 in]
                n499 = call "CsTool-CommitAll.vi"("OnlyOnChange (t)"=w1126, "Coerce Flag (f)"=w1126, "Handle Cluster"=w1125) -> ()  [unwired: 2 out]
              }
              frame "AlazarTech" {
                n500 = call "AlazarCardChannel.vi"("Channel tab"=w1137, "Digitizer Settings"=w1138) -> ("Channel"=w1136:u32, "Card ID"=w1133:u32)  [unwired: 7 in, 1 out]
                n501 = call "AlazarAbortAsyncRead.vi"("Handle"=w1133) -> ("Handle"=w1132:u64, "error out"=w1131:errorcluster)  [unwired: 1 in, 1 out]
                n502 = call "Alazar_ChannelConfig - ATS-SDK.vi"("error in (no error)"=w1131, "V scale"=w1139, "Channel"=w1136, "Handle in"=w1132) -> ("error out"=w1142:errorcluster, "Handle_Out"=w1143:u32)  [unwired: 1 in, 1 out]
                n503 = property on="Crate Delay" class="DigNum (strict)"() -> (error out=w1135:errorcluster, "Value"=w1134:dbl)  [unwired: 2 in, 1 out]
                n504 = call "Alazar_conTrig - ATS-SDK.vi"("error in (no error)"=w1142, "Trigger"=w1141, "Voltage Scale"=w1140, "Handle in"=w1143) -> ()  [unwired: 1 in, 2 out]
                n505 = property on="Crate Delay" class="DigNum (strict)"(error in=w1135, "Val(Sgnl)"=w1134) -> ()  [unwired: 1 in, 2 out]
              }
            }
            n506 = local read "Settings Changes"() -> (w1047:bool)
            n507 = Bundle By Name(cluster=w1057, "Trigger Settings"="Trigger Settings") -> (w1050:T31)
            n508 = case shown="True" w1047 {
              tunnel: w1051 -> [_ w1067]
              tunnel: w1048 -> [_ w1066]
              tunnel: w1050 -> [_ w1065]
              tunnel: w1049 -> [w1062 w1064]
              tunnel: [w1062 w1063] -> w1043
              frame False {
              }
              frame True {
                n509 = local read "T/R Channel"() -> (w1068:u32)
                n510 = call "UpdateDualXDCRSettings.vi"("Digitizer Settings in"=w1065, "Motion Settings in"=w1067, "Switch T/R"=w1068, "Dual XDCR Settings In"=w1064, "Switch Unit"=w1066) -> ("Dual XDCR Settings"=w1063:T3)  [unwired: 3 in]
              }
            }
          }
          event "Crate Voltage Scales", "Crate Coupling": Value Change {
            # "set up vertical (voltage scale) on crate"
            n511 = event-data() -> ()  [unwired: 2 out]
            n512 = case shown="True" w1149 {
              tunnel: w1148 -> [_ w1152]
              frame False {
              }
              frame True {
                n513 = Unbundle By Name(w1152) -> ("Main Digitizer"=w1151:T32, "Dig Config"=w1150:T33)
                n514 = local read "Trigger Settings"() -> (w1154:T37)
                n515 = case shown="\"Acqiris Digitizer\"" w1151 {
                  tunnel: "Crate Voltage Scales" -> [w1161 w1194 w1215 _]
                  tunnel: w1154 -> [w1168 w1193 w1214 _]
                  tunnel: "Crate Coupling" -> [w1167 w1195 w1216 _]
                  tunnel: w1150 -> [w1165 _ _ _]
                  tunnel: w1152 -> [w1156 w1192 w1213 _]
                  frame "Acqiris Digitizer" {
                    n516 = Decrement(x=w1165) -> (x-1=w1166:T33)
                    n517 = Unbundle By Name(w1156) -> ("Digitizer ID Cluster.Acqiris/Alazar/SP ID"=w1158:u32[])
                    n518 = Unbundle By Name(w1156) -> ("bits A/D"=w1157:i8)
                    n519 = Not Equal To 0?(x=w1166) -> (x != 0?=w1164:bool)
                    n520 = case shown="12" w1157 {
                      tunnel: [enum16{"DP 110", "DP 310"}."DP 110" ("Card Type") enum16{"DP 110", "DP 310"}."DP 310" ("Card Type")] -> w1159
                      frame 8, Default {
                      }
                      frame 12 {
                      }
                    }
                    n521 = Array Subset(array=w1161, length=1) -> (w1162:dbl[])  [unwired: 1 in]
                    n522 = Select(t=w1161, s=w1164, f=w1162) -> (s? t:f=w1163:dbl[])
                    n523 = for {
                      tunnel: w1167 -> [w1175]
                      tunnel: w1168 -> [w1174]
                      tunnel: [w1173] -> _
                      tunnel: w1163 -> [w1172] mode=indexing
                      tunnel: w1159 -> [_]
                      tunnel: w1158 -> [w1171]
                      i -> [w1179]
                      n524 = Index Array(array=w1171, index=1) -> (element=w1176:u32)
                      n525 = Bundle("Channel"=w1172, 0.0, "Crate Coupling"=w1175) -> (w1180:T60)  [unwired: 1 out]
                      n526 = Increment(x=w1179) -> (x+1=w1178:i32)
                      n527 = disable-structure shown="Disabled" {
                        disable-tunnel: w1180 -> [w1188 _]
                        disable-tunnel: w1178 -> [w1185 _]
                        disable-tunnel: w1176 -> [w1184 _]
                        disable-tunnel: w1174 -> [w1183 _]
                        disable-tunnel: [w1182 _] -> w1173
                        frame Disabled {
                          n528 = call "conVert.vi"("InstrumentID"=w1184, "V scale"=w1188, "Channel (1)"=w1185) -> ("Status"=w1186:i32, "error out"=w1187:errorcluster)  [unwired: 2 in, 1 out]
                          n529 = call "conTrig.vi"("error in"=w1187, "Trigger"=w1183, "InstrumentID"=w1186) -> ("error out"=w1182:errorcluster)  [unwired: 2 in, 1 out]
                        }
                        frame Enabled {
                        }
                      }
                    }
                  }
                  frame "NI Digitizer" {
                    n530 = Unbundle By Name(w1192) -> ("NI ID/Channel"=w1191:cluster{"NI ID":refnum<k15>, "NI CH":i32}[])
                    n531 = Array Subset(array=w1191, index=1) -> (w1190:cluster{"NI ID":refnum<k15>, "NI CH":i32}[])  [unwired: 1 in]
                    n532 = for {
                      tunnel: w1195 -> [w1205]
                      tunnel: w1194 -> [w1204] mode=indexing
                      tunnel: w1193 -> [w1200]
                      tunnel: [w1199] -> _
                      tunnel: w1190 -> [w1198] mode=indexing
                      n533 = Unbundle By Name(w1198) -> ("NI ID"=w1196:refnum<k15>, "NI CH"=w1197:i32)
                      n534 = Bundle("Channel"=w1204, 0.0, "Crate Coupling"=w1205) -> (w1203:T60)  [unwired: 1 out]
                      n535 = call "NIconVert.vi"("InstrumentID"=w1196, "V scale"=w1203, "Channel (0)"=w1197) -> ("Status"=w1202:refnum<k15>, "error out"=w1201:errorcluster)  [unwired: 1 in, 2 out]
                      n536 = call "NIconTrig.vi"("error in"=w1201, "Trigger"=w1200, "InstrumentID"=w1202) -> ("error out"=w1199:errorcluster)  [unwired: 2 out]
                    }
                  }
                  frame "AlazarTech" {
                    # "Handle two card case"
                    n537 = Unbundle By Name(w1213) -> ("Digitizer ID Cluster.Acqiris/Alazar/SP ID"=w1211:u32[])
                    n538 = Array Size(array=w1211) -> (size(s)=w1212:i32)
                    n539 = case shown="2" w1212 {
                      tunnel: w1211 -> [w1229 w1235]
                      tunnel: [w1226 w1232] -> w1210
                      tunnel: [w1230 w1231] -> w1209
                      frame 2 {
                        w1230 = u32[] [2, 1, 2] items=["A"=1, "B"=2, "C"=4, "D"=8]
                        n540 = Index Array(array=w1229) -> (element #1=w1228:u32, element #2=w1227:u32)  [unwired: 2 in]
                        n541 = Build Array(w1228, w1227, w1227) -> (w1226:u32[])
                      }
                      frame 1, Default {
                        w1231 = u32[] [2, 4, 8] items=["A"=1, "B"=2, "C"=4, "D"=8]
                        n542 = Index Array(array=w1235) -> (element=w1234:u32)  [unwired: 1 in]
                        n543 = Initialize Array(w1234, 3 ("dimension size")) -> (w1232:u32[])
                      }
                    }
                    n544 = for {
                      tunnel: w1216 -> [w1224]
                      tunnel: w1215 -> [w1218] mode=indexing
                      tunnel: w1214 -> [w1222]
                      tunnel: w1210 -> [w1221] mode=indexing
                      tunnel: w1209 -> [w1219] mode=indexing
                      n545 = Bundle("Channel"=w1218, 0.0, "Crate Coupling"=w1224) -> (w1220:T60)  [unwired: 1 out]
                      n546 = call "Alazar_ChannelConfig - ATS-SDK.vi"("V scale"=w1220, "Channel"=w1219, "Handle in"=w1221) -> ("error out"=w1217:errorcluster, "Handle_Out"=w1223:u32)  [unwired: 2 in, 1 out]
                      n547 = call "Alazar_conTrig - ATS-SDK.vi"("error in (no error)"=w1217, "Trigger"=w1222, "Voltage Scale"=w1218, "Handle in"=w1223) -> ()  [unwired: 1 in, 2 out]
                    }
                    n548 = property on="Crate Delay" class="DigNum (strict)"() -> (error out=w1208:errorcluster, "Value"=w1207:dbl)  [unwired: 2 in, 1 out]
                    n549 = property on="Crate Delay" class="DigNum (strict)"(error in=w1208, "Val(Sgnl)"=w1207) -> ()  [unwired: 1 in, 2 out]
                  }
                  frame "No Digitizer", Default {
                  }
                }
              }
            }
          }
          event "Slave Voltage Scales": Value Change {
            n550 = event-data() -> ("NewVal"=w1242:bool)  [unwired: 2 out]
            n551 = case shown="True" w1242 {
              frame False {
              }
              frame True {
                n552 = local read "Channel tab"() -> (w1246:enum32{"C1", "C2", "C3", "C4"})
                n553 = property on="Channel tab" class="TabCtl (strict)"("Val(Sgnl)"=w1246) -> ()  [unwired: 2 in, 2 out]
              }
            }
            n554 = Select(t=T44."Disabled and Grayed Out" ("Disabled"), s=w1242, f=T44."Enabled" ("Disabled")) -> (s? t:f=w1243:T44)
            n555 = property on="Crate Voltage Scales" class="Arr (strict)"("DisabledEnum"=w1243) -> ()  [unwired: 2 in, 2 out]
            n556 = property on="Crate Voltage Scales" class="Arr (strict)"("Visible"=TRUE) -> ()  [unwired: 2 in, 2 out]
          }
          event "Display Crate?": Value Change {
            n557 = event-data() -> ()  [unwired: 2 out]
            n558 = local read "Crate Voltage Scales"() -> (w1252:dbl[])
            n559 = local read "Crate Delay"() -> (w1253:dbl)
            n560 = property on="Crate Delay" class="DigNum (strict)"("Val(Sgnl)"=w1253) -> ()  [unwired: 2 in, 2 out]
            n561 = property on="Crate Voltage Scales" class="Arr (strict)"("Val(Sgnl)"=w1252) -> ()  [unwired: 2 in, 2 out]
          }
          event "T/R Channel": Value Change {
            n562 = event-data() -> ("NewVal"=w1258:u32, "OldVal"=w1263:u32)  [unwired: 1 out]
            n563 = Bundle By Name(cluster=w1259, "Switch T/R"=w1258) -> (w1257:T23)
            n564 = case shown="\"No Switch\", Default" w1266 {
              tunnel: w1258 -> [w1270 w1273 w1277 w1298 w1353]
              tunnel: w1267 -> [_ _ _ w1296 _]
              tunnel: w1263 -> [_ _ _ w1297 _]
              tunnel: w1265 -> [w1268 w1271 w1275 w1291 w1352]
              tunnel: [w1268 w1271 w1275 w1291 w1349] -> w1264
              tunnel: w1262 -> [w1269 w1272 w1276 w1292 w1351]
              tunnel: [w1269 w1272 w1276 w1292 w1350] -> w1261
              tunnel: w1260 -> [_ _ _ _ w1348]
              tunnel: w1257 -> [_ _ _ w1293 _]
              tunnel: w1256 -> [_ _ _ _ w1347]
              tunnel: w1255 -> [_ _ _ _ w1346]
              tunnel: w1254 -> [_ _ _ w1289 _]
              frame "Cytex" {
                n565 = call "Cytex.vi"("Xmit Ring"=w1270) -> ()  [unwired: 2 in, 3 out]
              }
              frame "Pickering" {
                n566 = disable-structure shown="Disabled" {
                  disable-tunnel: w1273 -> [w1274 _]
                  frame Disabled {
                    n567 = call "PickeringBlank.vi"("Xmit Ring"=w1274) -> ()  [unwired: 5 out]
                  }
                  frame Enabled {
                  }
                }
              }
              frame "NI Switch" {
                n568 = disable-structure shown="Disabled" {
                  disable-tunnel: w1277 -> [w1288 _]
                  frame Disabled {
                    n569 = Decrement(x=w1288) -> (x-1=w1287:u32)
                    n570 = Number To Decimal String(number=w1287) -> (decimal integer string=w1286:string)  [unwired: 1 in]
                    n571 = Concatenate Strings("ch", w1286) -> (w1278:string)
                    n572 = global read "MotionGlobals.vi" "NI Switch"() -> (w1280:refnum<k15>)
                    n573 = call <instrlib>:"niSwitch Disconnect All Channels.vi"("instrument handle"=w1280) -> ("error out"=w1282:errorcluster, "instrument handle out"=w1281:refnum<k15>)  [unwired: 9 in]
                    n574 = call-poly <instrlib>:"niSwitch Connect Channels.vi"("error in (no error)"=w1282, "channel 2"="com0", "channel 1"=w1278, "instrument handle"=w1281) -> ("error out"=w1283:errorcluster, "instrument handle out"=w1284:refnum<k15>)  [unwired: 6 in]
                    n575 = call <instrlib>:"niSwitch Wait For Debounce.vi"("error in (no error)"=w1283, "instrument handle"=w1284) -> ()  [unwired: 8 in, 2 out]
                  }
                  frame Enabled {
                  }
                }
              }
              frame "No Switch", Default {
                n576 = Unbundle By Name(w1291) -> ("Dig Config"=w1290:T33)
                n577 = Unbundle By Name(w1293) -> ("Trans Geometry (mm)"=w1295:T24, "Sub Ap Excite?"=w1294:bool)
                n578 = case shown="\"5-CH Pulser New\"" w1290 {
                  tunnel: w1298 -> [w1305 w1341]
                  tunnel: w1297 -> [w1304 _]
                  tunnel: w1296 -> [w1303 _]
                  tunnel: w1291 -> [w1301 _]
                  tunnel: w1295 -> [w1300 _]
                  tunnel: w1294 -> [w1299 _]
                  tunnel: w1289 -> [_ w1338]
                  frame "Single channel", Default {
                    n579 = local read "CTR Tasks"() -> (w1302:refnum<k21>[])
                    n580 = case shown="False" w1299 {
                      tunnel: w1305 -> [w1312 w1331]
                      tunnel: w1304 -> [w1310 _]
                      tunnel: [_ w1328] -> _
                      tunnel: w1303 -> [_ w1327]
                      tunnel: w1302 -> [w1306 w1324]
                      tunnel: w1301 -> [_ w1321]
                      tunnel: w1300 -> [_ w1320]
                      frame False {
                        w1307 = 5
                        w1308 = 1
                        n581 = In Range and Coerce(upper limit=w1308, x=w1312, lower limit=w1307) -> (coerced(x)=w1311:u32)  [unwired: 1 out]
                        n582 = In Range and Coerce(upper limit=w1308, x=w1310, lower limit=w1307) -> (coerced(x)=w1309:u32)  [unwired: 1 out]
                        n583 = Decrement(x=w1311) -> (x-1=w1319:u32)
                        n584 = Decrement(x=w1309) -> (x-1=w1315:u32)
                        n585 = Array Subset(array=w1306, length=5) -> (w1314:refnum<k21>[])  [unwired: 1 in]
                        n586 = Index Array(array=w1314, index=w1319) -> (element=w1318:refnum<k21>)
                        n587 = Index Array(array=w1314, index=w1315) -> (element=w1316:refnum<k21>)
                        n588 = call <vilib>:"DAQmx Stop Task.vi"("task/channels in"=w1316) -> ("error out"=w1317:errorcluster)  [unwired: 13 in, 1 out]
                        n589 = call <vilib>:"DAQmx Start Task.vi"("task/channels in"=w1318, "error in"=w1317) -> ()  [unwired: 12 in, 2 out]
                      }
                      frame True {
                        n590 = Equal?(x=location."WCM Main" ("Location"), y=w1327) -> (x = y?=w1322:bool)
                        n591 = for {
                          tunnel: w1324 -> [w1333] mode=indexing
                          tunnel: [w1332] -> w1323
                          n592 = call <vilib>:"DAQmx Clear Task.vi"("task in"=w1333) -> ("error out"=w1332:errorcluster)  [unwired: 14 in]
                        }
                        n593 = Decrement(x=w1331) -> (x-1=w1330:u32)
                        n594 = call "5ChTrigs_ABUT.vi"("xmit ring"=w1330, "Trans Geometry (mm)"=w1320, "Digitizer Settings"=w1321, "M-mode?"=w1322, "error in"=w1323) -> ("5CH Pulser Tasks"=w1325:refnum<k21>[], "error out"=w1329:errorcluster)  [unwired: 4 in]
                        n595 = local write "CTR Tasks"(w1325) -> ()
                        n596 = for {
                          tunnel: w1325 -> [w1336] mode=indexing
                          shift-right: [w1334] -> w1328
                          shift-left: w1329 -> [w1335]
                          n597 = call <vilib>:"DAQmx Start Task.vi"("task/channels in"=w1336, "error in"=w1335) -> ("error out"=w1334:errorcluster)  [unwired: 12 in, 1 out]
                        }
                      }
                    }
                  }
                  frame "5-CH Pulser New" {
                    # "Turn off transmits except for selected"
                    n598 = Decrement(x=w1341) -> (x-1=w1340:u32)
                    n599 = expression code="1E6/x"(w1338) -> (w1337:dbl)
                    n600 = Replace Array Subset(array=i32[] [-1, -1, -1, -1, -1], new element=0, index=w1340) -> (w1343:i32[])
                    n601 = Build Array(w1343) -> (w1342:i32[][])
                    n602 = global read "PulserGlobals.vi" "Daxsonics VISA"() -> (w1345:refnum<visa-resource-name>)
                    n603 = call "DelayTableLoad.vi"("PRI (ns)"=w1337, "Delay Table (ns)"=w1342, "VISA Refnum in"=w1345) -> ()  [unwired: 9 in]
                  }
                }
              }
              frame "Riverside USB" {
                n604 = case shown="\"Dual Transducer\"" w1346 {
                  tunnel: w1353 -> [w1355 w1374]
                  tunnel: w1352 -> [w1358 w1373]
                  tunnel: w1351 -> [w1357 w1372]
                  tunnel: [w1357 w1370] -> w1350
                  tunnel: [w1358 w1368] -> w1349
                  tunnel: w1348 -> [_ w1362]
                  tunnel: w1347 -> [_ w1360]
                  frame "Therapy With Scan", Default {
                    n605 = global read "SwitchGlobals.vi" "USB Switch"() -> (w1356:string)
                    n606 = Decrement(x=w1355) -> (x-1=w1354:u32)
                    n607 = call "RiversideRelaySetChannel.vi"("serial_number"=w1356, "Transducer"=w1354) -> ()  [unwired: 3 in, 3 out]
                  }
                  frame "Dual Transducer" {
                    n608 = control-ref of="Time scale per Div"() -> (w1366:refnum<vi>)
                    n609 = control-ref of="RF data Sampling"() -> (w1365:refnum<vi>)
                    n610 = Unbundle By Name(w1362) -> ("XDCR Offset"=w1361:dbl[])
                    n611 = control-ref of="Filter Prameters"() -> (w1359:refnum<vi>)
                    n612 = call "ChooseDualXDCRSettings.vi"("Digitizer Settings in"=w1373, "Switch T/R"=w1374, "Pulser"=w1360, "Motion Settings in"=w1372, "Dual XDCR Settings"=w1362, "Time scale per Div Ref"=w1366, "RF data Sampling Ref"=w1365, "Filter Parameters Ref"=w1359) -> ("Digitizer Settings"=w1368:T31, "Change Polarity"=w1369:i32, "Motion Settings"=w1371:T27)  [unwired: 17 in]
                    n613 = Array Size(array=w1361) -> (size(s)=w1364:i32)
                    n614 = Not Equal To 0?(x=w1364) -> (x != 0?=w1363:bool)
                    n615 = case shown="True" w1363 {
                      tunnel: w1371 -> [w1375 w1383]
                      tunnel: [w1375 w1381] -> w1370
                      tunnel: w1369 -> [_ w1382]
                      tunnel: w1361 -> [_ w1376]
                      frame False {
                      }
                      frame True {
                        n616 = Two Button Dialog(message="Move XDCR Offset?", 1:"Dont Move" ("F button name (\"Cancel\")"), 2:"Move" ("T button name (\"OK\")")) -> (T button?=w1377:bool)
                        n617 = case shown="True" w1377 {
                          tunnel: w1383 -> [w1384 w1393]
                          tunnel: w1382 -> [_ w1391]
                          tunnel: [w1384 w1388] -> w1381
                          tunnel: w1376 -> [_ w1385]
                          frame False {
                          }
                          frame True {
                            n618 = local read "Axis Tune"() -> (w1392:enum32{"Axis 1", "Axis 2", "Axis 3", "Axis 4"})
                            n619 = call "MultiAxisMove.vi"("Find Location"=TRUE, "Position Mode (Rel)"=T45."Relative Position" ("Position Mode (Absolute)"), "Distance to move (mm)"=w1385, "Move Polarity"=w1391, "Motion Settings"=w1393) -> ("location (mm)"=w1389:dbl[], "Motion Settings Out"=w1388:T27)  [unwired: 4 in, 1 out]
                            n620 = Index Array(array=w1389, index=w1392) -> (element=w1387:dbl)
                            n621 = property on="Position (mm) (Abs)" class="DigNum (strict)"("Value"=w1387) -> ()  [unwired: 2 in, 2 out]
                          }
                        }
                      }
                    }
                    n622 = Unbundle By Name(w1368) -> ("Voltage Scale"=w1367:dbl)
                    n623 = property on="Volt Scale 1" class="Ring (strict)"("Val(Sgnl)"=w1367) -> ()  [unwired: 2 in, 2 out]
                  }
                }
              }
            }
          }
          event "Set Pulser": Value Change {
            # "set up Panametrics if option is selected"
            n624 = event-data() -> ()  [unwired: 2 out]
            n625 = flat-sequence {
              tunnel: w1396 -> [w1403]
              tunnel: w1394 -> [w1402]
              tunnel: w1401 -> [w1410]
              tunnel: w1400 -> [w1409]
              tunnel: w1399 -> [w1408]
              tunnel: w1398 -> [w1407]
              tunnel: [w1406] -> w1397
              frame #0 {
                n626 = call "SetAllPulsersGUI.vi"("Init Tabor?"=FALSE ("Init?"), "Tabor handle in"=w1402, "Pulser"=w1403) -> ()  [unwired: 9 in]
              }
              frame #1 {
                n627 = local read "Settings Changes"() -> (w1405:bool)
                n628 = case shown="True" w1405 {
                  tunnel: w1409 -> [_ w1417]
                  tunnel: w1408 -> [_ w1416]
                  tunnel: w1410 -> [_ w1414]
                  tunnel: w1407 -> [w1411 w1413]
                  tunnel: [w1411 w1412] -> w1406
                  frame False {
                  }
                  frame True {
                    n629 = local read "T/R Channel"() -> (w1415:u32)
                    n630 = call "UpdateDualXDCRSettings.vi"("Digitizer Settings in"=w1416, "Motion Settings in"=w1417, "Switch T/R"=w1415, "Dual XDCR Settings In"=w1413, "Switch Unit"=w1414) -> ("Dual XDCR Settings"=w1412:T3)  [unwired: 3 in]
                  }
                }
              }
            }
          }
          event Value Change {
            n631 = event-data() -> ()  [unwired: 7 out]
            n632 = call "PulserSettingsSwitch.vi"("Pulser"="Pulser", "Digitizer Settings in"=w1421, "Offset delay (us)"="Offset delay (us)", "Delay Corr?"="Delay Corr?") -> ("Digitizer Settings out"=w1419:T31)  [unwired: 9 in, 2 out]
            n633 = Unbundle By Name(w1419) -> ("Offset delay (us)"=w1418:dbl)
            n634 = property on="Offset delay (us)" class="DigNum (strict)"("Value"=w1418) -> ()  [unwired: 2 in, 2 out]
          }
          event "One Way Transmission?": Value Change {
            n635 = event-data() -> ()  [unwired: 7 out]
            n636 = Bundle By Name(cluster=w1429, "One Way Transmission?"="One Way Transmission?") -> (w1427:T31)
          }
          event "Custom Waveform": Value Change {
            n637 = event-data() -> ()  [unwired: 3 out]
            n638 = call "Chirp.vi"() -> ()  [unwired: 6 in, 1 out]
          }
          event "Man Cont": Value Change {
            n639 = event-data() -> ()  [unwired: 2 out]
            n640 = Unbundle By Name(w1444) -> ("Motion System"=w1443:T28)
            n641 = case shown="\"NI 735x\", Default" w1443 {
              tunnel: w1444 -> [w1447 w1449 w1455 w1457 w1460]
              tunnel: [w1447 w1448 w1454 w1457 w1459] -> w1442
              frame "MM3000" {
                # "Old send command mm2k control"
              }
              frame "NI 735x", Default {
                n642 = disable-structure shown="Disabled" {
                  disable-tunnel: w1449 -> [w1451 w1453]
                  disable-tunnel: [w1450 w1453] -> w1448
                  frame Disabled {
                    n643 = call "NI_controller.VI"("Motion Settings"=w1451, "Initialize"=FALSE) -> ("Motion Settings Out"=w1450:T27)  [unwired: 3 in, 1 out]
                  }
                  frame Enabled {
                  }
                }
              }
              frame "Newport ESP" {
                n644 = call "ESPControl.vi"("Motion Settings"=w1455, "# Axis"=u16 2) -> ("Motion Settings Out"=w1454:T27)  [unwired: 3 in, 1 out]
              }
              frame "No Motion Card" {
              }
              frame "Galil" {
                n645 = call "GL_controller.VI"("Motion Settings"=w1460, "Initialize"=FALSE) -> ("Motion Settings Out"=w1459:T27)  [unwired: 3 in, 1 out]
              }
            }
            n646 = local read "Axis Tune"() -> (w1446:enum32{"Axis 1", "Axis 2", "Axis 3", "Axis 4"})
            n647 = property on="Axis Tune" class="RadioBtnsControl (strict)"("Val(Sgnl)"=w1446) -> ()  [unwired: 2 in, 2 out]
          }
          event "Axis Tune": Value Change {
            # "move to global location"
            n648 = event-data() -> ()  [unwired: 4 out]
            n649 = Unbundle By Name(w1466) -> ("Motion System"=w1465:T28)
            n650 = case shown="\"NI 735x\", Default" w1465 {
              tunnel: w1466 -> [w1469 w1473]
              tunnel: [w1468 w1473] -> w1464
              frame "NI 735x", Default {
                n651 = call "FindLocation.vi"("Motion Settings"=w1469) -> ("Motion Settings Out"=w1468:T27, "location (mm)"=w1471:dbl[])  [unwired: 2 in, 2 out]
                n652 = Index Array(array=w1471, index="Axis Tune") -> (element=w1470:dbl)
                n653 = local write "Position (mm) (Abs)"(w1470) -> ()
              }
              frame "MM3000", "Newport ESP", "No Motion Card" {
              }
            }
          }
          event "Position (mm) (Abs)": Value Change {
            # "Update axis location"
            n654 = event-data() -> ()  [unwired: 4 out]
            n655 = Unbundle By Name(w1474) -> ("Reverse Z axis?"=w1479:bool, "Steps per mm"=w1481:i32[])
            n656 = local read "Axis Tune"() -> (w1476:enum32{"Axis 1", "Axis 2", "Axis 3", "Axis 4"})
            n657 = Index Array(array=w1481, index=w1476) -> (element=w1480:i32)
            n658 = Multiply(x="Position (mm) (Abs)", y=w1480) -> (x*y=w1477:dbl)
            n659 = To Byte Integer(number=w1476) -> (8bit integer=w1478:i8)
            n660 = case shown="2" w1478 {
              tunnel: w1477 -> [w1488 w1491]
              tunnel: [w1488 w1490] -> w1475
              tunnel: w1479 -> [_ w1489]
              frame 0, Default {
              }
              frame 2 {
                n661 = Negate(x=w1491) -> (-x=w1492:dbl)
                n662 = Select(t=w1492, s=w1489, f=w1491) -> (s? t:f=w1490:dbl)
              }
            }
            n663 = Unbundle By Name(w1474) -> ("Motion System"=w1486:T28)
            n664 = case shown="\"NI 735x\", Default" w1486 {
              tunnel: w1474 -> [_ w1494 w1511]
              tunnel: w1478 -> [_ w1495 w1508]
              tunnel: w1475 -> [_ w1493 w1507]
              frame "MM3000", "Newport ESP", "No Motion Card" {
              }
              frame "NI 735x", Default {
                n665 = disable-structure shown="Disabled" {
                  disable-tunnel: w1495 -> [w1499 _]
                  disable-tunnel: w1494 -> [w1498 _]
                  disable-tunnel: w1493 -> [w1496 _]
                  frame Disabled {
                    n666 = Unbundle By Name(w1498) -> ("Motion Bd ID"=w1497:u8)
                    n667 = Increment(x=w1499) -> (x+1=w1506:i8)
                    n668 = call <vilib>:"Set Operation Mode.flx"("Axis or Vector Space"=w1506, "Board ID"=w1497) -> ("error out"=w1505:errorcluster, "Resource Output"=w1503:T61, "Bd ID Out"=w1504:T62)  [unwired: 4 in]
                    n669 = call <vilib>:"Load Target Position.flx"("Target Position (0)"=w1496, "error in (no error)"=w1505, "Axis"=w1503, "Board ID"=w1504) -> ("error out"=w1501:errorcluster, "Resource Output"=w1500:T61, "Bd ID Out"=w1502:T62)  [unwired: 3 in]
                    n670 = call-poly <vilib>:"Start Motion.flx"("error in (no error)"=w1501, "Axis or Vector Space"=w1500, "Board ID"=w1502) -> ()  [unwired: 3 in, 3 out]
                  }
                  frame Enabled {
                  }
                }
              }
              frame "Galil" {
                n671 = Unbundle By Name(w1511) -> ("GL Ref Out"=w1510:refnum<k7>)
                n672 = call "GL Set Operation Mode.vi"("position cts (abs/rel)"=w1507, "Start Now?"=TRUE, "Axis"=w1508, "Galil.IGalil"=w1510) -> ()  [unwired: 5 in, 3 out]
              }
            }
          }
          event "Stop Motor": Value Change {
            n673 = event-data() -> ()  [unwired: 4 out]
            n674 = Unbundle By Name(w1513) -> ("Motion System"=w1512:T28)
            n675 = case shown="\"NI 735x\"" w1512 {
              tunnel: w1513 -> [w1519 w1521 w1536]
              tunnel: [w1519 w1520 w1535] -> w1517
              frame "MM3000", Default {
              }
              frame "NI 735x" {
                n676 = disable-structure shown="Disabled" {
                  disable-tunnel: w1521 -> [w1523 _]
                  disable-tunnel: [w1522 _] -> w1520
                  frame Disabled {
                    n677 = Unbundle By Name(w1523) -> ("Motion Bd ID"=w1524:u8)
                    n678 = local read "Axis Tune"() -> (w1527:enum32{"Axis 1", "Axis 2", "Axis 3", "Axis 4"})
                    n679 = Increment(x=w1527) -> (x+1=w1530:enum32{"Axis 1", "Axis 2", "Axis 3", "Axis 4"})
                    n680 = call-poly <vilib>:"Stop Motion.flx"("Stop Type (Decel)"=enum16{"Decelerate", "Halt", "Kill"}."Halt", "Axis or Vector Space"=w1530, "Board ID"=w1524) -> ("error out"=w1528:errorcluster)  [unwired: 4 in, 2 out]
                    n681 = call "FindLocation.vi"("Motion Settings"=w1523, "error in (no error)"=w1528) -> ("Motion Settings Out"=w1522:T27, "location (mm)"=w1526:dbl[])  [unwired: 1 in, 2 out]
                    n682 = Index Array(array=w1526, index=w1527) -> (element=w1525:dbl)
                    n683 = local write "Position (mm) (Abs)"(w1525) -> ()
                  }
                  frame Enabled {
                  }
                }
              }
              frame "Galil" {
                n684 = Unbundle By Name(w1536) -> ("GL Ref Out"=w1532:refnum<k7>)
                n685 = call "GL Command Set.vi"("Command"=Command_Menu."Abort Motion", "Galil.IGalil"=w1532) -> ("error out"=w1531:errorcluster)  [unwired: 5 in, 4 out]
                n686 = call "FindLocation.vi"("Motion Settings"=w1536, "error in (no error)"=w1531) -> ("Motion Settings Out"=w1535:T27, "location (mm)"=w1538:dbl[])  [unwired: 1 in, 2 out]
                n687 = local read "Axis Tune"() -> (w1533:enum32{"Axis 1", "Axis 2", "Axis 3", "Axis 4"})
                n688 = Index Array(array=w1538, index=w1533) -> (element=w1537:dbl)
                n689 = local write "Position (mm) (Abs)"(w1537) -> ()
              }
            }
          }
          event "Save trace?": Value Change {
            n690 = event-data() -> ()  [unwired: 2 out]
            n691 = local read "Waveform Graph"() -> (w1545:cluster{i32, dbl, "Array":dbl[]})
            n692 = local read "t per div"() -> (w1544:dbl)
            n693 = Unbundle(w1545) -> (w1554:dbl, "Array"=w1553:dbl[])  [unwired: 1 out]
            n694 = for {
              tunnel: w1554 -> [w1556]
              tunnel: w1553 -> [_] mode=indexing
              tunnel: [w1555] -> w1550 mode=indexing
              i -> [w1557]
              n695 = Multiply(x=w1556, y=w1557) -> (x*y=w1555:dbl)
            }
            n696 = Select(t=1, s=w1546, f=w1544) -> (s? t:f=w1547:dbl)
            n697 = Multiply(x=w1550, y=w1547) -> (x*y=w1549:dbl[])
            n698 = Build Array(w1549, w1553) -> (w1552:dbl[][])
            n699 = Transpose 2D Array(2D array=w1552) -> (transposed array=w1551:dbl[][])
            n700 = call-poly <vilib>:"Write Delimited Spreadsheet.vi"("2D data"=w1551) -> ()  [unwired: 13 in, 2 out]
          }
          event "Therapy Burst Set Up.Divide prf by", "Therapy Burst Set Up.Therapy Delay (ms)", "Gate duration (mics)": Value Change {
            n701 = event-data() -> ()  [unwired: 2 out]
            n702 = Unbundle("Therapy Burst Set Up") -> ("Therapy Set Up"=w1570:T63, "Divide prf by"=w1571:i32, "Therapy Delay (ms)"=w1572:dbl, "Counter On (T)"=w1564:bool)
            n703 = Multiply(x="Gate duration (mics)", y=1e-06) -> (x*y=w1566:dbl)
            n704 = Unbundle By Name(w1570) -> ("Cycles"=w1568:sgl)
            n705 = call "ExtPRFCount.vi"("Therapy Delay (ms)"=w1572, "Start Counter?"=w1564, "Divide prf by"=w1571, "pulse width (s or cycles)"=w1566) -> ()  [unwired: 12 out]
            n706 = Multiply(x=w1563, y=w1568) -> (x*y=→"Lines in burst":dbl)
          }
          event "Therapy Burst Set Up.Therapy Set Up": Value Change {
            # "Set up burst parameters"
            # "Pause Therapy if needed."
            n707 = event-data() -> ("NewVal"=w1580:T63)  [unwired: 1 out]
            n708 = case shown="1" "Func Gen" {
              tunnel: w1580 -> [w1586 w1588]
              tunnel: "cycles (f), time(t)" -> [w1585 _]
              tunnel: w1582 -> [_ w1587]
              frame 0, Default {
                n709 = global read "MotionGlobals.vi" "33250(T)/33120(F)"() -> (w1583:bool)
                n710 = call "TherapyBurst.vi"("Input Cluster"=w1586, "VISA session in"="Therapy VISA session", "33250(T)/33120(F)"=w1583, "Trigger (F) Gate(T)"=w1585) -> ()  [unwired: 1 in, 4 out]
              }
              frame 1 {
                n711 = call "TaborBurst.vi"("Input Cluster"=w1588, "instrument in"=w1587) -> ()  [unwired: 1 in, 6 out]
              }
            }
          }
          event "Therapy Burst Set Up.Counter On (T)": Value Change {
            n712 = event-data() -> ("NewVal"=w1596:bool)  [unwired: 1 out]
            n713 = local read "CTR Tasks"() -> (w1595:refnum<k21>[])
            n714 = Index Array(array=w1595) -> (element=w1594:refnum<k21>)  [unwired: 1 in]
            n715 = case shown="False" w1596 {
              tunnel: w1594 -> [w1597 w1598]
              frame False {
                n716 = call <vilib>:"DAQmx Stop Task.vi"("task/channels in"=w1597) -> ()  [unwired: 1 in, 14 out]
              }
              frame True {
                n717 = call <vilib>:"DAQmx Start Task.vi"("task/channels in"=w1598) -> ()  [unwired: 1 in, 14 out]
              }
            }
          }
          event "Config Breath": Value Change {
            n718 = event-data() -> ()  [unwired: 2 out]
            n719 = global read "MotionGlobals.vi" "Breath Trig"() -> (w1604:T64)
            n720 = local read "Time scale per Div"() -> (w1605:dbl)
            n721 = case shown="1, Default" w1604 {
              tunnel: w1603 -> [_ w1606]
              frame 0 {
              }
              frame 1, Default {
                n722 = call "BreathTrig.vi"("SetUp Mode"=TRUE, "Digitizer Settings"=w1606) -> ()  [unwired: 2 in, 8 out]
              }
            }
            n723 = property on="Time scale per Div" class="Ring (strict)"("Val(Sgnl)"=w1605) -> ()  [unwired: 2 in, 2 out]
          }
          event "Attenuation": Value Change {
            n724 = event-data() -> ()  [unwired: 7 out]
            n725 = call "SetAttn.vi"("Attenuation"="Attenuation") -> ()  [unwired: 10 in, 1 out]
          }
          event "Set Spectrometer": Value Change {
            n726 = event-data() -> ()  [unwired: 7 out]
            n727 = global read "MotionGlobals.vi" "Main Spectrometer"() -> (w1619:T65)
            n728 = case shown="1" w1619 {
              frame 0, Default {
              }
              frame 1 {
                # "OceanSetUp_ViewLV"
              }
            }
          }
          event "ExitSendCmd": Value Change {
            n729 = event-data() -> ("NewVal"=w1624:bool)  [unwired: 1 out]
            n730 = property on="ExitSendCmd" class="Bool (strict)"("Value"=FALSE ("ExitSendCmd")) -> ()  [unwired: 2 in, 2 out]
          }
        }
        n731 = Build Array (concatenate)(w293, w286) -> (w292:dbl[][])
        n732 = Array Subset(array=w292, length (row)=20) -> (w291:dbl[][])  [unwired: 3 in]
      }
    }
    frame #5 {
      # "turn off prf"
      n733 = Unbundle By Name(w1631) -> ("Motion System"=w1630:T28)
      n734 = call "PRF_Off.vi"("Location"=w1628, "Motion Settings In"=w1631) -> ()  [unwired: 9 in, 1 out]
      n735 = Unbundle By Name(w1633) -> ("Main Digitizer"=w1632:T32)
      n736 = local read "CTR Tasks"() -> (w1629:refnum<k21>[])
      n737 = case shown="\"Acqiris Digitizer\", Default" w1632 {
        tunnel: w1633 -> [_ w1643]
        tunnel: w1627 -> [_ w1638]
        frame "Acqiris Digitizer", Default {
        }
        frame "AlazarTech" {
          n738 = Unbundle By Name(w1643) -> ("Digitizer ID Cluster.Acqiris/Alazar/SP ID"=w1642:u32[])
          n739 = Index Array(array=w1642) -> (element=w1640:u32)  [unwired: 1 in]
          n740 = Select(t=u32 14, s=w1638, f=u32 13) -> (s? t:f=w1635:u32)
          n741 = call "AlazarConfigureAuxIO.vi"("Parameter"=u32 0, "Mode"=w1635, "Handle"=w1640) -> ("Handle"=w1639:u64)  [unwired: 1 in, 2 out]
          n742 = call "AlazarAbortAsyncRead.vi"("Handle"=w1639) -> ()  [unwired: 1 in, 3 out]
        }
      }
      n743 = case shown="\"No Motion Card\"" w1630 {
        tunnel: w1634 -> [_ w1644]
        frame "MM3000", Default {
        }
        frame "No Motion Card" {
          n744 = call-poly <vilib>:"DAQmx Write.vi"("task/channels in"=w1644, "data"=FALSE) -> ()  [unwired: 11 in, 3 out]
        }
      }
      n745 = case shown="\"WCM Main\"" w1628 {
        tunnel: w1633 -> [w1648 _ _]
        tunnel: w1629 -> [w1646 _ w1651]
        frame "WCM Main" {
          n746 = Unbundle By Name(w1648) -> ("Dig Config"=w1647:T33)
          n747 = case shown="\"5-CH pulser w/ ann array\"" w1647 {
            tunnel: w1646 -> [_ w1649]
            frame "Single channel", Default {
            }
            frame "5-CH pulser w/ ann array" {
              n748 = for {
                tunnel: w1649 -> [w1650] mode=indexing
                n749 = call <vilib>:"DAQmx Clear Task.vi"("task in"=w1650) -> ()  [unwired: 14 in, 1 out]
              }
            }
          }
        }
        frame "SERI GP", Default {
        }
        frame "CUMC RT" {
          n750 = for {
            tunnel: w1651 -> [w1654] mode=indexing
            n751 = call <vilib>:"DAQmx Stop Task.vi"("task/channels in"=w1654) -> ("task out"=w1653:refnum<k21>, "error out"=w1652:errorcluster)  [unwired: 13 in]
            n752 = call <vilib>:"DAQmx Clear Task.vi"("task in"=w1653, "error in"=w1652) -> ()  [unwired: 13 in, 1 out]
          }
        }
      }
    }
    frame #6 {
      # "Stop counter afte therapy burst or EKG modes"
      n753 = global read "MotionGlobals.vi" "EKG Gate?"() -> (w1655:T66)
      n754 = Not Equal To 0?(x=w1655) -> (x != 0?=w1661:bool)
      n755 = local read "CTR Tasks"() -> (w1657:refnum<k21>[])
      n756 = Compound Arithmetic op=OR(w1658, w1662, w1661, w1660) -> (w1659:bool)
      n757 = case shown="\"Cytex\", Default" w1663 {
        tunnel: w1657 -> [_ w1664]
        frame "Cytex", Default {
        }
        frame "No Switch" {
          n758 = for {
            tunnel: w1664 -> [w1665] mode=indexing
            n759 = call <vilib>:"DAQmx Stop Task.vi"("task/channels in"=w1665) -> ()  [unwired: 1 in, 14 out]
          }
        }
      }
      n760 = case shown="False" w1659 {
        tunnel: w1657 -> [_ w1667]
        frame False {
        }
        frame True {
          n761 = Index Array(array=w1667) -> (element=w1666:refnum<k21>)  [unwired: 1 in]
          n762 = call <vilib>:"DAQmx Stop Task.vi"("task/channels in"=w1666) -> ()  [unwired: 1 in, 14 out]
        }
      }
      n763 = call <instrlib>:"ww128x Close.vi"("instrument handle"=w1656) -> ()  [unwired: 10 in, 1 out]
    }
  }
  "Digitizer Settings Out" <- w12
  "Motion Settings Out" <- w16
  "Ann Array Params out" <- w9
  "Dual XDCR Settings Out" <- w11
  n764 = global write "DigitizerGlobals.vi" "Digitizer Settings"(w12) -> ()
  n765 = global write "MotionGlobals.vi" "Motion Settings"(w16) -> ()
  n766 = global write "PulserGlobals.vi" "Pulser"(w8) -> ()
